vi "myRIO_BRig_RT_v0,76__PortC.vi"() -> ()   [LabVIEW 2014]
uses:
  <vilib>/Platform/TimedLoop/XDataNode/XDataNode.xnode
  <vilib>/Platform/TimedLoop/XDataNode/nitl_modes.ctl
  <vilib>/Platform/TimedLoop/XDataNode/XDNodeRunTimeDep.lvlib
  <vilib>/Platform/TimedLoop/XDataNode/wakeup.ctl
  <vilib>/Platform/TimedLoop/XDataNode/timing_clust.ctl
  <vilib>/rvi/interface/nirviReadWriteControl/nirviReadWriteControl.xnode
  <vilib>/rvi/interface/Simulation/niFpgaSimulationCallBeginRW.vi
  <vilib>/rvi/errors/niLvFpgaAdjustHostInterfaceError.vi
  <vilib>/rvi/interface/nirviCloseFPGA/nirviCloseFPGA.xnode
  <vilib>/myRIO/Instrument Drivers/Utilities/Utilities.lvlib
  <vilib>/rvi/interface/nirviOpenFPGA/nirviOpenFPGA.xnode
  myRIO_BRig_RT__Case_Exp_stateList.ctl
  <vilib>/WebDAVClient/Advanced/SessionHandle.ctl
  <vilib>/WebDAVClient/NI_WebDAV.lvlib
  myRIO_BRig_RT__Case_NonExp_stateList.ctl
  NiFpgaLv.dll
  <vilib>/Utility/error.llb/Error Cluster From Error Code.vi
  <vilib>/FPGAPlugInAG/Dynamic/niLvFpga_Close_Dynamic.vi
  myRIO_BRig_FPGA_v3,61__PortC__build.lvbitx
  myRIO_BRig_FPGA_v3,61__PortC.vi
  <vilib>/FPGAPlugInAG/myRIO-1900/niLvFpga_Open_myRIO-1900.vi
  <vilib>/rvi/interface/common/dynamic/niFpgaDynamicAddResources.vi
panel:
  in  "laser2_power_step":dbl
  in  "laser2_power_max":dbl
  in  "laser2_power_min":dbl
  in  "laser2_Tshutter":dbl=2.0
  in  "laser2_Freq":dbl=10.0
  in  "laser2_Tpeak":dbl=2.0
  in  "laser2_duration":u16
  in  "LC_l2_Sel_All_Count":u16
  in  "LC_l2_Sel_First_Count":u16
  in  "LC_l2_Sel_All_Probability":u16
  in  "LC_l2_Sel_All_Block":u16(slide) max=2 step=1 scale=0.0..2.0
  in  "LC_l2_Sel_All_OnOff":bool
  in  "LC_l2_Sel_First_Probability":u16
  in  "LC_l2_Sel_First_Block":u16(slide) max=2 step=1 scale=0.0..2.0
  in  "LC_l2_Sel_First_OnOff":bool
  in  "LC_l2_Sel_All_Tdelay":u16
  in  "LC_l2_Sel_First_Tdelay":u16
  in  "LC_l2_Cue1_All_Count":u16
  in  "LC_l2_Cue1_First_Count":u16
  in  "LC_l2_Cue1_All_delayOpt":bool
  in  "LC_l2_ENL1_All_delayOpt":bool
  in  "LC_l2_ENL1_All_Count":u16
  in  "LC_l2_ENL1_First_Count":u16
  in  "LC_l2_Cue1_First_delayOpt":bool
  in  "LC_l2_ENL1_First_delayOpt":bool
  in  "LC_l2_Cue1_All_Probability":u16
  in  "LC_l2_Cue1_All_Block":u16(slide) max=2 step=1 scale=0.0..2.0
  in  "LC_l2_Cue1_All_OnOff":bool
  in  "LC_l2_Cue1_First_Probability":u16
  in  "LC_l2_Cue1_First_Block":u16(slide) max=2 step=1 scale=0.0..2.0
  in  "LC_l2_Cue1_First_OnOff":bool
  in  "LC_l2_ENL1_All_Probability":u16 max=100 step=1
  in  "LC_l2_ENL1_All_Block":u16(slide) max=2 step=1 scale=0.0..2.0
  in  "LC_l2_ENL1_All_OnOff":bool
  in  "LC_l2_ENL1_First_Probability":u16 max=100 step=1
  in  "LC_l2_ENL1_First_Block":u16(slide) max=2 step=1 scale=0.0..2.0
  in  "LC_l2_Cue1_All_Tdelay":u16
  in  "LC_l2_ENL1_All_Tdelay":u16
  in  "LC_l2_Cue1_First_Tdelay":u16
  in  "LC_l2_ENL1_First_Tdelay":u16
  in  "LC_l2_ENL1_First_OnOff":bool
  in  "LC_l2_Wrong_Probability":u16
  in  "LC_l2_Wrong_Trial":u16(slide) max=2 step=1 scale=0.0..2.0
  in  "LC_l2_Wrong_Block":u16(slide) max=2 step=1 scale=0.0..2.0
  in  "LC_l2_Wrong_OnOff":bool
  in  "LC_l2_Reward_Probability":u16
  in  "LC_l2_Reward_Trial":u16(slide) max=2 step=1 scale=0.0..2.0
  in  "LC_l2_Reward_Block":u16(slide) max=2 step=1 scale=0.0..2.0
  in  "LC_l2_Reward_OnOff":bool
  in  "LC_l2_Wrong_Tdelay":u16
  in  "LC_l2_Reward_Tdelay":u16
  in  "LC_l1_Sel_All_Count":u16
  in  "LC_l1_Sel_First_Count":u16
  in  "LC_l1_Sel_All_Probability":u16
  in  "LC_l1_Sel_All_Block":u16(slide) max=2 step=1 scale=0.0..2.0
  in  "LC_l1_Sel_All_OnOff":bool
  in  "LC_l1_Sel_First_Probability":u16
  in  "LC_l1_Sel_First_Block":u16(slide) max=2 step=1 scale=0.0..2.0
  in  "LC_l1_Sel_First_OnOff":bool
  in  "LC_l1_Sel_All_Tdelay":u16
  in  "LC_l1_Sel_First_Tdelay":u16
  out "I_connect_TCP":bool
  out "error out 5":errorcluster
  in  "get_countPerMS":bool
  in  "count_warmup_R_reset":bool
  in  "count_warmup_L_reset":bool
  out "count_warmup_R":u16
  out "count_warmup_L":u16
  out "SolenoidReward":bool
  in  "SolenoidProbability_L":u16=50 caption="Reward Time [ms]" min=1 max=1000 step=1
  in  "SolenoidProbability_R":u16=50 caption="Reward Time [ms]" min=1 max=1000 step=1
  out "output_PortA":dbl caption="LaserPower"
  out "error out 4":errorcluster
  in  "laser1_power_step":dbl
  in  "laser1_power_max":dbl
  in  "Recording":bool
  out "error out 3":errorcluster
  out "error out 2":errorcluster
  in  "laser1_power_min":dbl
  in  "FPGA_count2ms":dbl=159.0
  in  "laser1_Tshutter":dbl=2.0
  in  "laser1_Freq":dbl=10.0
  in  "laser1_Tpeak":dbl=2.0
  in  "laser1_duration":u16
  out "error out":errorcluster
  in  "LC_l1_Cue1_All_Count":u16
  in  "LC_l1_Cue1_First_Count":u16
  in  "LC_l1_Cue1_All_delayOpt":bool
  in  "LC_l1_ENL1_All_delayOpt":bool
  in  "LC_l1_ENL1_All_Count":u16
  in  "LC_l1_ENL1_First_Count":u16
  in  "LC_l1_Cue1_First_delayOpt":bool
  in  "LC_l1_ENL1_First_delayOpt":bool
  in  "Tcycle_Cue_max":u16=1000 caption="Max" min=5 max=5000 step=5
  in  "Tcycle_Cue_min":u16=1000 caption="Min" min=5 max=5000 step=5
  in  "SendData":bool
  out "cSpout":enum16{"Left", "Right"}(ring) caption="Left or Right Spout"
  out "A4":u32 caption="LickCounter_Right"
  out "A2":u32 caption="LickCounter_Left"
  in  "laserResponse_wrong_LED":bool
  out "error_initTrial":errorcluster
  out "error_Selection_pre":errorcluster
  out "error_Selection":errorcluster
  out "SelectWrong":bool
  out "SelectReward":bool
  in  "Left(F)_or_Right(T)":bool
  in  "ignoreWrong":bool
  in  "SelectionState":bool
  in  "laserResponse_wrong":bool
  in  "laserResponse_reward":bool
  in  "laserResponse_reward_LED":bool
  out "nRewards_Right":u16 caption="# Rewards Total (Right)"
  out "nRewards_Left":u16 caption="# Rewards Total (Left)"
  out "nRewards_cur":u16 caption="# Rewards in Current Block"
  out "TpB_target":u16 caption="Target Trials Per Block"
  out "cState_NonExp":T1 caption="WarmUp State"
  out "iBlock":u16 caption="Current Block"
  out "cState":T2 caption="Experimental State"
  out "iTrial":u16 caption="Current Trial"
  in  "warmupType":u8(slide) max=2 step=1 scale=0.0..2.0
  in  "TestConnection":bool
  in  "warmup":bool caption="WarmUp"
  in  "Data Set Prefix":string="Exp1_TM2"
  out "Connected To Host?":bool
  in  "Host Password":string="sabalab"
  in  "Host UserName":string="Test2"
  in  "sp_RightSpout":u16(slide)=2 max=2 step=1 scale=0.0..2.0
  in  "sp_LeftSpout":u16(slide)=2 max=2 step=1 scale=0.0..2.0
  in  "BUR_max":u16 caption="Count Reward Structure  (0 = off)"
  in  "LC_l1_Wrong_Probability":u16
  in  "LC_l1_Wrong_Trial":u16(slide) max=2 step=1 scale=0.0..2.0
  in  "LC_l1_Wrong_Block":u16(slide) max=2 step=1 scale=0.0..2.0
  in  "LC_l1_Wrong_OnOff":bool
  in  "LC_l1_Reward_Probability":u16
  in  "LC_l1_Reward_Trial":u16(slide) max=2 step=1 scale=0.0..2.0
  in  "LC_l1_Reward_Block":u16(slide) max=2 step=1 scale=0.0..2.0
  in  "LC_l1_Reward_OnOff":bool
  in  "LC_l1_Cue1_All_Probability":u16
  in  "LC_l1_Cue1_All_Block":u16(slide) max=2 step=1 scale=0.0..2.0
  in  "LC_l1_Cue1_All_OnOff":bool
  in  "LC_l1_Cue1_First_Probability":u16
  in  "LC_l1_Cue1_First_Block":u16(slide) max=2 step=1 scale=0.0..2.0
  in  "LC_l1_Cue1_First_OnOff":bool
  in  "LC_l1_ENL1_All_Probability":u16 max=100 step=1
  in  "LC_l1_ENL1_All_Block":u16(slide) max=2 step=1 scale=0.0..2.0
  in  "LC_l1_ENL1_All_OnOff":bool
  in  "LC_l1_ENL1_First_Probability":u16 max=100 step=1
  in  "LC_l1_ENL1_First_Block":u16(slide) max=2 step=1 scale=0.0..2.0
  in  "Tcycle_Timeout":u16=1000 caption="Timeout Time [ms]" min=10 max=10000 step=1
  in  "Tcycle_Wrong":u16=1000 caption="Wrong Time [ms]" min=10 max=10000 step=1
  in  "Tcycle_Selection":u16=1000 caption="Answer Time [ms]" min=1 max=10000 step=1
  in  "Tcycle_RewardPost":u16=1000 caption="Consumption Time [ms]" min=250 max=10000 step=250
  in  "Tcycle_Reward_L":u16=500 caption="Reward Time [ms]" min=1 max=1000 step=1
  in  "Tcycle_Reward_R":u16=500 caption="Reward Time [ms]" min=1 max=1000 step=1
  in  "TpB_Max_R":u16=4 caption="Max TrialsPerBlock" min=1 max=12 step=1
  in  "TpB_Min_R":u16=4 caption="Min TrialsPerBlock" min=1 max=12 step=1
  in  "TpB_Max_L":u16=4 caption="Max TrialsPerBlock" min=1 max=12 step=1
  in  "TpB_Min_L":u16=4 caption="Min TrialsPerBlock" min=1 max=12 step=1
  in  "BUR_min":u16 caption="Count Reward Structure\n(0 = off)"
  in  "TrialUntilReward":bool caption="Ignore Wrong Selection"
  in  "CueCycles":u16=1 caption="Cue Structure" min=1 max=1 step=1
  in  "MTrig_Laser_Tcycle":u16=10 caption="Time [ms]"
  in  "MTrig_Laser_trig":bool
  in  "MTrig_Audio_trig__R":bool caption="Trigger Audio"
  in  "MTrig_Audio_trig__L":bool caption="Trigger Audio"
  in  "RewCalib_Trig_R":bool caption="Calibrate_R"
  in  "RewCalib_Trig_L":bool caption="Calibrate_L"
  in  "MTrig_Solenoid_Tcycle__R":u16=300 caption="Time [ms]"
  in  "MTrig_Solenoid_Tcycle__L":u16=300 caption="Time [ms]"
  in  "MTrig_Solenoid_trig__R":bool caption="Solenoid"
  in  "MTrig_Solenoid_trig__L":bool caption="Solenoid"
  in  "STOP_abort":bool caption="Stop LabView\n(Stops myRio and FPGA)"
  in  "STOP_endBlock":bool caption="Stop Experiment\n@ End of Block"
  in  "STOP_endTrial":bool caption="Stop Experiment\n@ End of Trial"
  in  "START":bool caption="Start Experiment"
  in  "Tcycle_CuePenalty":u16=1000 caption="Penalty" min=1 max=10000 step=1
  in  "Audio_Amp__R":u16=100 caption="Amp"
  in  "Audio_Freq__R":u8=5 caption="Freq [kHz]" max=14 step=1
  in  "Audio_Amp__L":u16=100 caption="Amp"
  in  "Audio_Freq__L":u8=5 caption="Freq [kHz]" max=14 step=1
  in  "LC_l1_Wrong_Tdelay":u16
  in  "LC_l1_Cue1_All_Tdelay":u16
  in  "LC_l1_ENL1_All_Tdelay":u16
  in  "LC_l1_Reward_Tdelay":u16
  in  "LC_l1_Cue1_First_Tdelay":u16
  in  "LC_l1_ENL1_First_Tdelay":u16
  in  "LC_l1_ENL1_First_OnOff":bool
  in  "Tcycle_ENLPenalty":u16=100 caption="Penalty" min=10 max=10000 step=10
  in  "Tcycle_ENL_max":u16=1000 caption="Max" min=250 max=10000 step=250
  in  "Tcycle_ENL_min":u16=1000 caption="Min" min=250 max=10000 step=250
  # "Communication (Host PC)"
  # "Recording Rig"
  # "Experimental Run"
  # "Current State"
  # "STOP experiment at"
  # "Global Parameters                                                         Trial Parameters"
  # "Left/Right        Give Reward?        Laser Power [V]"
  # "FPGA Count per [ms]"
  # "Experiment Task Structure"
  # "Timing [ms]"
  # "Block                   Trial            Target Trials       # Rewards \n                                                            Per Block             Current"
  # "Min            Max            Penalty"
  # "(1) = Switching\n(2) = Two Choice"
  # "WarmUp State"
  # "Lick Counter"
  # "Enforced\nNonLick"
  # "WarmUp"
  # "Left           Right"
  # "Cue then reward (no lick)\n \nLeft                    Right"
  # "# Rewards Total\n                                                                  Left                    Right"
  # "Cue"
  # "Experimental State"
  # "Selection\n \n\n \nReward\n    Dispense\n    Time\n \n    Dispense\n    Probability\n \n\n    Consumption\n    Time\n\nWrong Choice\n \n \nTimeout Penalty"
  # "Laser1 Control\n                               On/Off      Block        Probability [%]   Delay [ms]                              Count"
  # "Left                  Right"
  # "Manual Control"
  # "Enforced\nNonLick\n      1"
  # "Min"
  # "Max"
  # "from end"
  # "Solenoid\n \nLeft              Right"
  # "Switch\nTrial"
  # "Speaker\n \nLeft                    Right"
  # "Laser"
  # "from start"
  # "Trial Per Block Structure \n               Left                        Right"
  # "from end"
  # "NonSwitch\nTrials"
  # "from start"
  # "Time\n[ms]"
  # "Time\n[ms]"
  # "Time = Cue Min"
  # "Min"
  # "Cue 1"
  # "Power = Min"
  # "from end"
  # "Switch\nTrial"
  # "Max"
  # "from start"
  # "Speaker Parameters"
  # "Laser1 Parameters"
  # "Left                  Right"
  # "from end"
  # "Laser1 Response\n                               On/Off      Block       Trial       Probability [%]   Delay [ms]"
  # "Frequency\n[Hz]"
  # "NonSwitch\nTrials"
  # "Frequency\n[kHz]"
  # "from start"
  # "Timing [ms]\n Duration     Peak Width   Shutter"
  # "Selection Reward"
  # "Selection"
  # "Amp\n(0 - 32,000)"
  # "from start"
  # "Switch\nTrial"
  # "Laser Power [V]\nMin          Max              Step"
  # "Speaker\nPattern\nDuring Cue"
  # "Selection Wrong"
  # "from start"
  # "NonSwitch\nTrials"
  # "Laser2 Parameters"
  # "Laser2 Response\n                               On/Off      Block       Trial       Probability [%]   Delay [ms]"
  # "Laser2 Control\n                               On/Off      Block        Probability [%]   Delay [ms]                              Count"
  # "Frequency\n[Hz]"
  # "Selection Reward"
  # "Enforced\nNonLick\n      1"
  # "from end"
  # "Timing [ms]\n Duration     Peak Width   Shutter"
  # "Switch\nTrial"
  # "from start"
  # "Selection Wrong"
  # "from end"
  # "Laser Power [V]\nMin          Max              Step"
  # "NonSwitch\nTrials"
  # "from start"
  # "Cue 1"
  # "from end"
  # "Switch\nTrial"
  # "from start"
  # "from end"
  # "NonSwitch\nTrials"
  # "from start"
  # "Selection"
  # "from start"
  # "Switch\nTrial"
  # "from start"
  # "NonSwitch\nTrials"
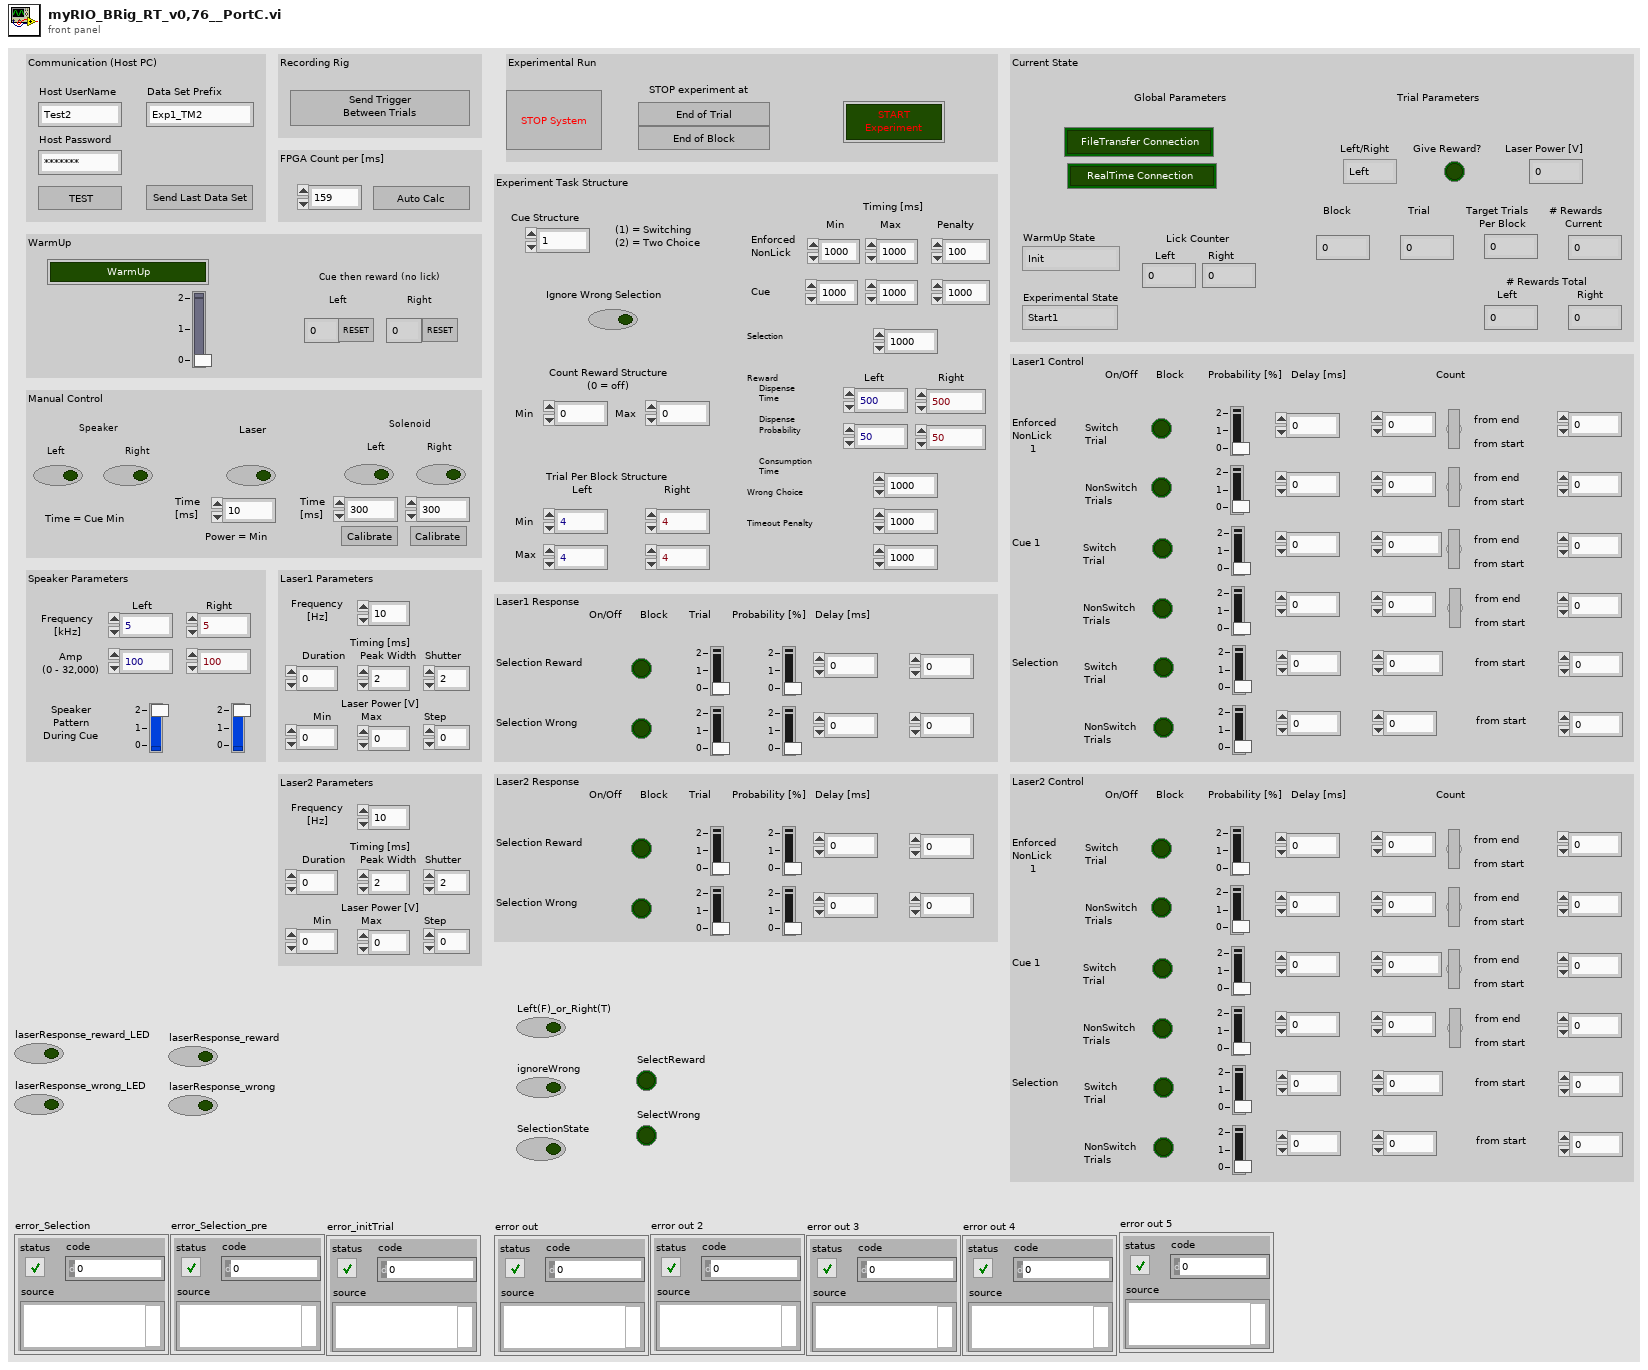
[diagram p1: front panel]
types:
  T1 = typedef "myRIO_BRig_RT__Case_NonExp_stateList.ctl" = enum16{"Init", "UploadSettings_pre", "UploadSettings_Read_dataExp", "UploadSettings_dataExp_1", "UploadSettings_dataExp_2", "UploadSettings_Read_dataLC", "UploadSettings_dataLC_1", "UploadSettings_dataLC_2", "UploadSettings_dataLC_3", "UploadSettings_dataLC_4", "UploadSettings_Read_dataMTrig", "UploadSettings_dataMTrig_1", "UploadSettings_post", "Idle_pre", "IdleEmpty", "IdleEmpty2", "IdleEmpty3", "IdleEmpty4", "Idle", "Idle_2", "Idle_3", "Idle_4", "Idle_5", "Idle_6", "Idle_post", "Cue_pre__pre", "Cue_pre", "Cue", "Cue_LED", "Cue_post", "RewardCalibration_pre", "DispenseWater_pre__pre", "DispenseWater_pre", "DispenseWater", "DispenseWater_post", "TestConnection", "SendData", "Get_FPGA_count_per_ms", "End"}
  T2 = typedef "myRIO_BRig_RT__Case_Exp_stateList.ctl" = enum16{"Start1", "Start2", "Start3", "saveSettings1", "saveSettings2", "saveSettings3", "saveSettings4", "saveSettings_LC_ENL_l1", "saveSettings_LC_ENL_l2", "saveSettings_LC_Cue_l1", "saveSettings_LC_Cue_l2", "saveSettings6_LC_l1_Other", "SaveSettings6_LC_l2_Other", "setSettings_Audio", "setSettings_Laser", "initBlock_pre", "initBlock", "initBlock2", "initBlock_post", "initTrial_pre", "initTrial", "initTrial2", "initTrial3", "initTrial4", "initTrial_LC_ENL1", "initTrial_LC_Cue1", "initTrial_LC_Cue1_2", "initTrial_LC_Sel", "initTrial_post", "ENL1_pre", "ENL1", "ENL1_post", "ENL1Penalty_pre", "ENL1Penalty", "ENL2_pre", "ENL2", "ENL2Penalty_pre", "ENL2Penalty", "Cue1_pre", "Cue1", "Cue1_post", "Cue1Penalty_pre", "Cue1Penalty", "Cue2_pre", "Cue2", "Cue2Penalty_pre", "Cue2Penalty", "Selection_pre", "Selection", "Select_post", "SelectReward_pre", "SelectReward", "SelectRewardPost_pre", "SelectRewardPost", "SelectWrong_pre", "SelectWrong", "SelectWrong_post", "SelectTimeout_pre", "SelectTimeout", "SelectTimeout_post", "endTrial_pre", "endTrial1", "endTrial2", "endTrial3", "endTrial_post", "endBlock_pre", "endBlock", "endBlock_post", "endExp", "commConnect", "commUpload_pre", "commUpload_dataBlock", "commUpload_dataCurrent", "commUpload_dataExp", "commUpload_dataLC", "commUpload_dataTrial", "commUpload_post", "saveData_pre", "saveData_dataBlock", "saveData_dataCurrent", "saveData_dataExp", "saveData_dataLC", "saveData_dataTrial", "saveData_post", "empty_endBlock1", "empty_endBlock2", "empty_endTrial1", "empty_endTrial2", "empty_endTrial3", "empty_endTrial4", "empty_endTrial5", "dummyState", "dummyState_endBlock"}
  T3 = typedef "XDNodeRunTimeDep.lvlib/timing_clust.ctl" = cluster{"Expected End [f-1]":u64, "Actual End [f-1]":u64, "Finished Late? [f-1]":bool, "Expected End [i-1]":u64, "Actual End [i-1]":u64, "Finished Late? [i-1]":bool, "Expected Start [i]":u64, "Actual Start [i]":u64, "Expected Start [f]":u64, "Actual Start [f]":u64, "Source Name":string, "Structure Name":string, "Period":i64, "Deadline":i64, "Offset":i64, "Start":i64, "Priority":i32, "Timeout":i32, "Mode":T4, "Wakeup Reason":T5, "Error":errorcluster, "Source Type":string, "Secondary Source Type":string, "Global End Time":u64, "Global Start Time":u64, "Frame Duration":u64, "Iteration Duration":u64, "Assigned CPU":i32, "I/O Scan Engine Mode":u32}
  T4 = typedef "XDNodeRunTimeDep.lvlib/nitl_modes.ctl" = enum32{"No Change", "Process missed periods, maintain original phase", "Discard missed periods, maintain original phase", "Process missed periods, ignore original phase", "Discard missed periods, ignore original phase"}
  T5 = typedef "XDNodeRunTimeDep.lvlib/wakeup.ctl" = enum32{"Normal", "Aborted", "Asynchronous wakeup", "Timing source error", "Timed loop error", "Timeout"}
  T6 = typedef "myRIO_BRig_RT__Case_Exp_stateList.ctl" = enum16{"Start1", "Start2", "Start3", "saveSettings1", "saveSettings2", "saveSettings3", "saveSettings4_LC_l1_ENL", "saveSettings4_LC_l2_ENL", "saveSettings5_LC_l1_Cue", "saveSettings5_LC_l2_Cue", "saveSettings6_LC_l1_Other", "SaveSettings6_LC_l2_Other", "setSettings_Audio", "setSettings_Laser", "initBlock_pre", "initBlock", "initBlock2", "initBlock_post", "initTrial_pre", "initTrial", "initTrial2", "initTrial3", "initTrial4", "initTrial_LC_ENL1", "initTrial_LC_Cue1", "initTrial_LC_Cue1_2", "initTrial_LC_Sel", "initTrial_post", "ENL1_pre", "ENL1", "ENL1_post", "ENL1Penalty_pre", "ENL1Penalty", "ENL2_pre", "ENL2", "ENL2Penalty_pre", "ENL2Penalty", "Cue1_pre", "Cue1", "Cue1_post", "Cue1Penalty_pre", "Cue1Penalty", "Cue2_pre", "Cue2", "Cue2Penalty_pre", "Cue2Penalty", "Selection_pre", "Selection", "Select_post", "SelectReward_pre", "SelectReward", "SelectRewardPost_pre", "SelectRewardPost", "SelectWrong_pre", "SelectWrong", "SelectWrong_post", "SelectTimeout_pre", "SelectTimeout", "SelectTimeout_post", "endTrial_pre", "endTrial1", "endTrial2", "endTrial3", "endTrial_post", "endBlock_pre", "endBlock", "endBlock_post", "endExp", "commConnect", "commUpload_pre", "commUpload_dataBlock", "commUpload_dataCurrent", "commUpload_dataExp", "commUpload_dataLC", "commUpload_dataTrial", "commUpload_post", "saveData_pre", "saveData_dataBlock", "saveData_dataCurrent", "saveData_dataExp", "saveData_dataLC", "saveData_dataTrial", "saveData_post", "empty_endBlock1", "empty_endBlock2", "empty_endTrial1", "empty_endTrial2", "empty_endTrial3", "empty_endTrial4", "empty_endTrial5", "dummyState", "dummyState_endBlock"}
  T7 = typedef "NI_WebDAV.lvlib/SessionHandle.ctl" = refnum<k1>
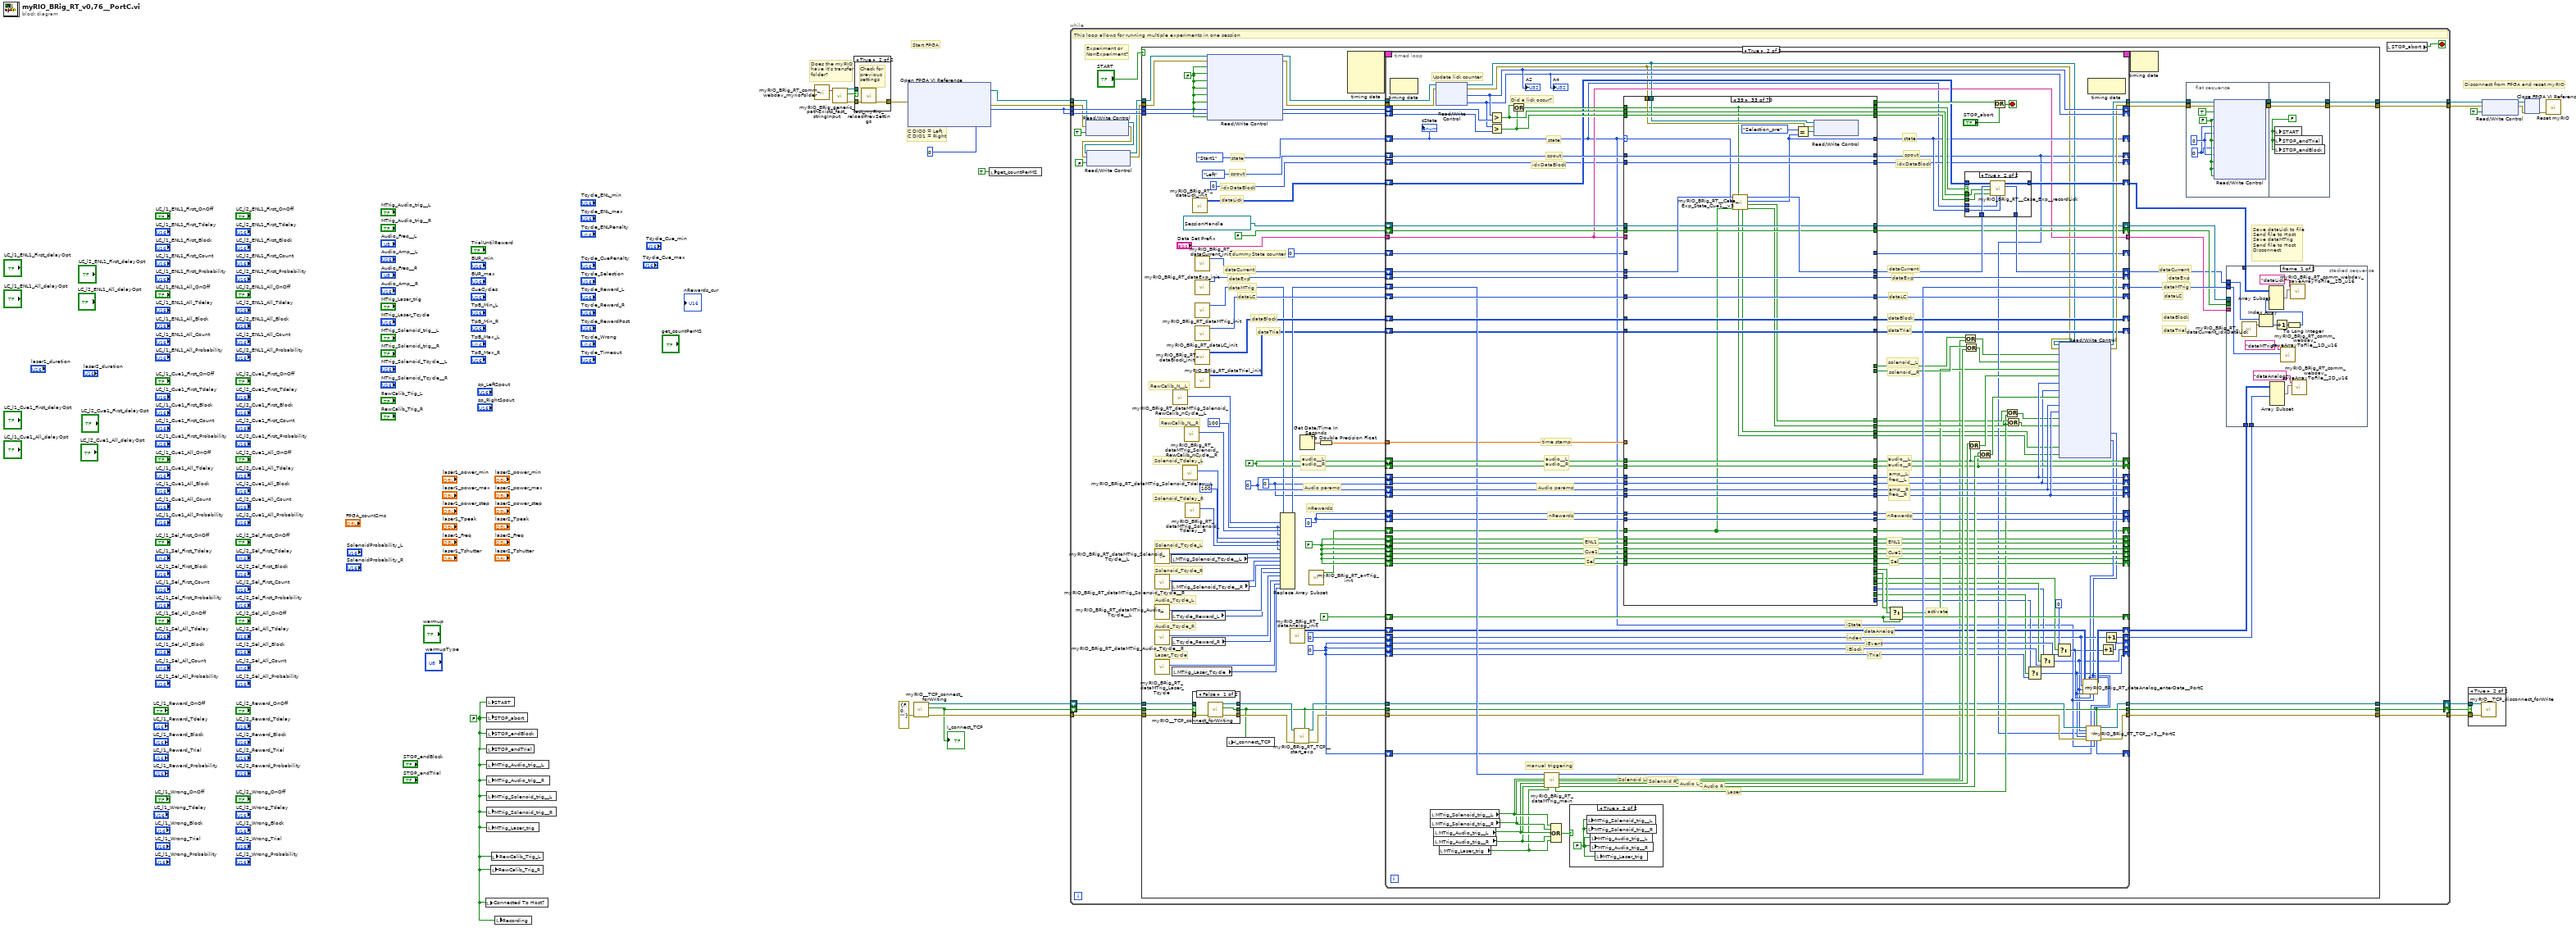
[diagram p0: block diagram]
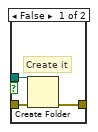
[diagram p3: hidden frame]
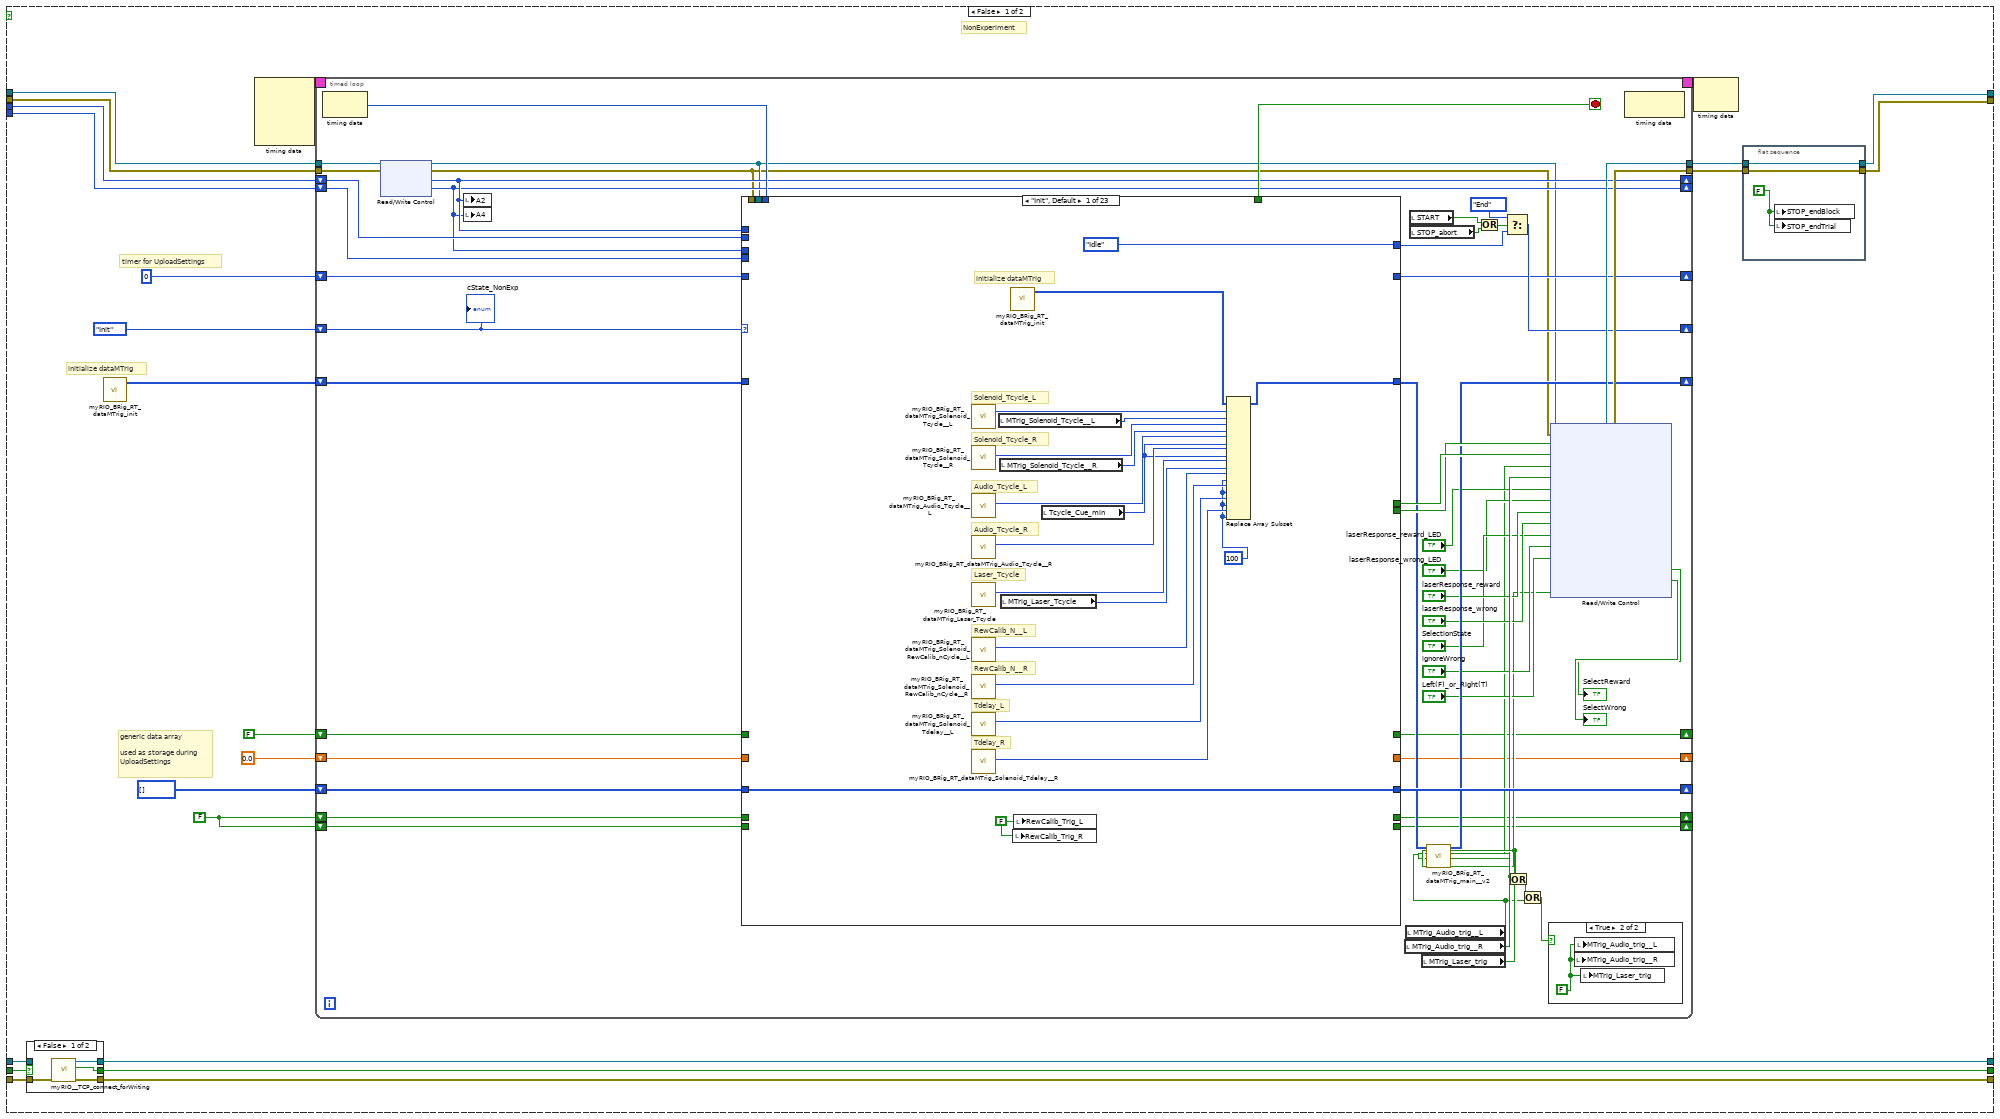
[diagram p4: hidden frame]
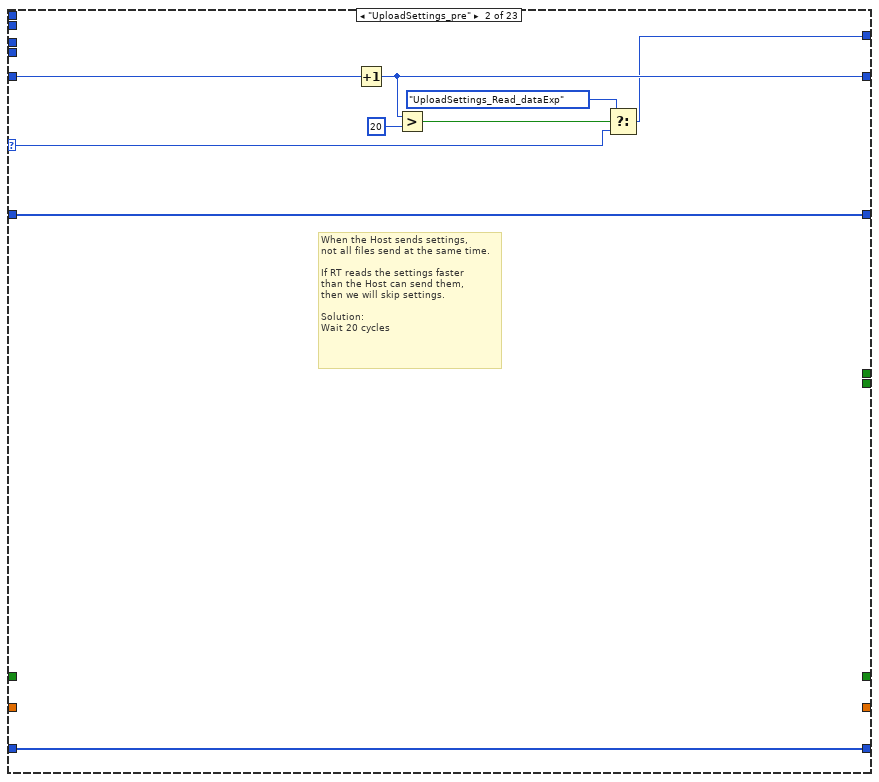
[diagram p7: hidden frame]
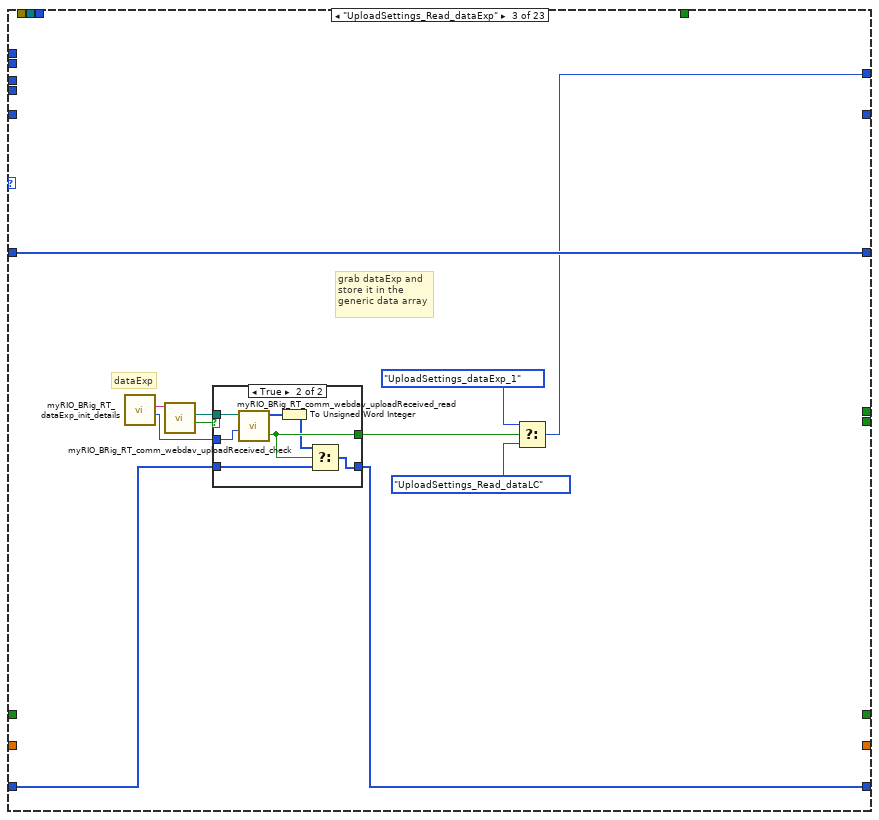
[diagram p8: hidden frame]
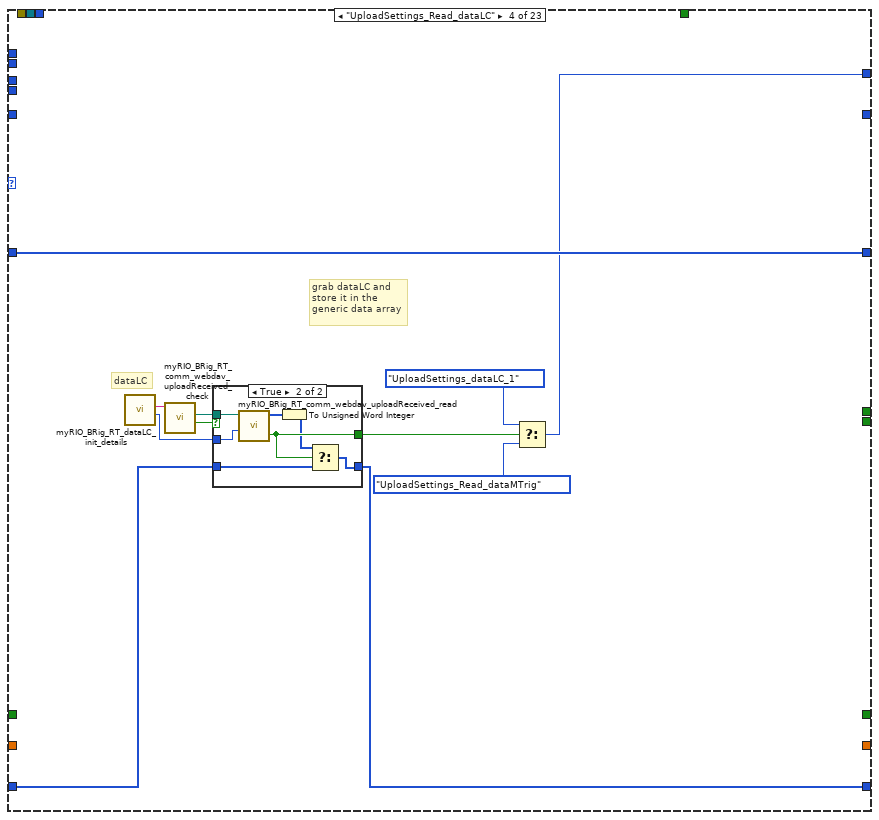
[diagram p10: hidden frame]
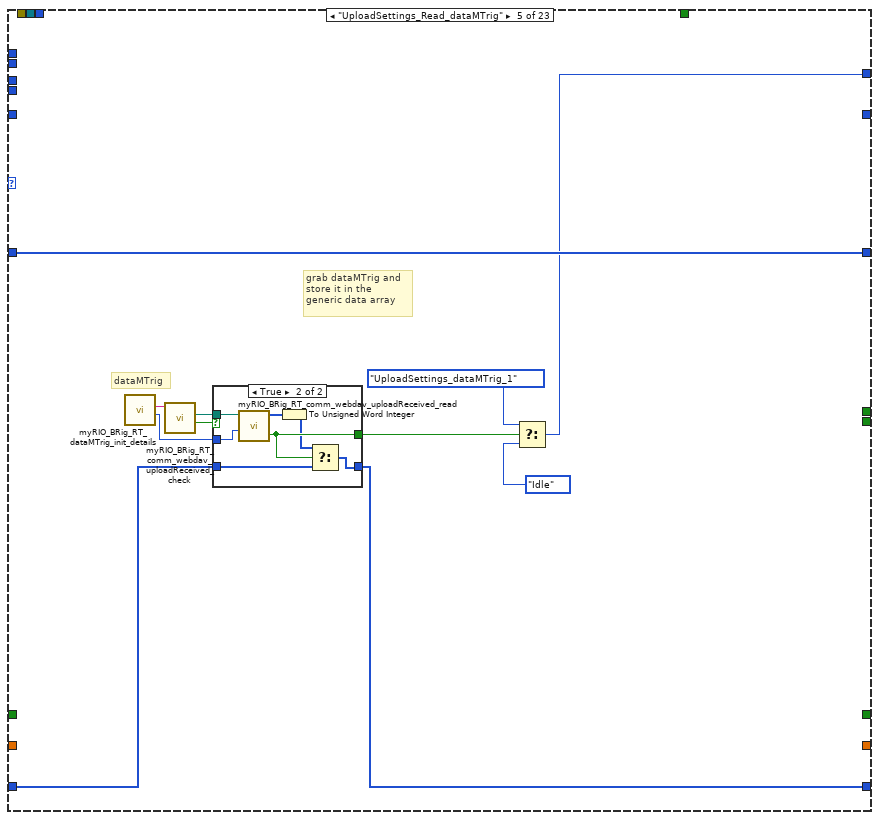
[diagram p12: hidden frame]
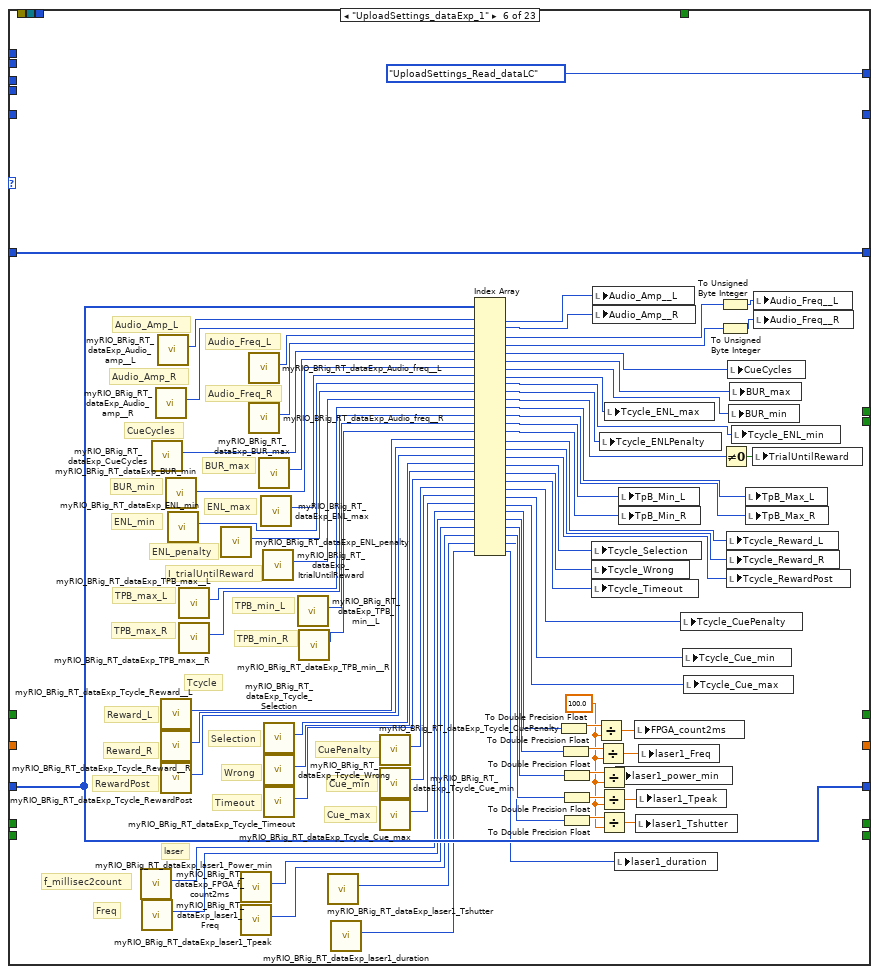
[diagram p14: hidden frame]
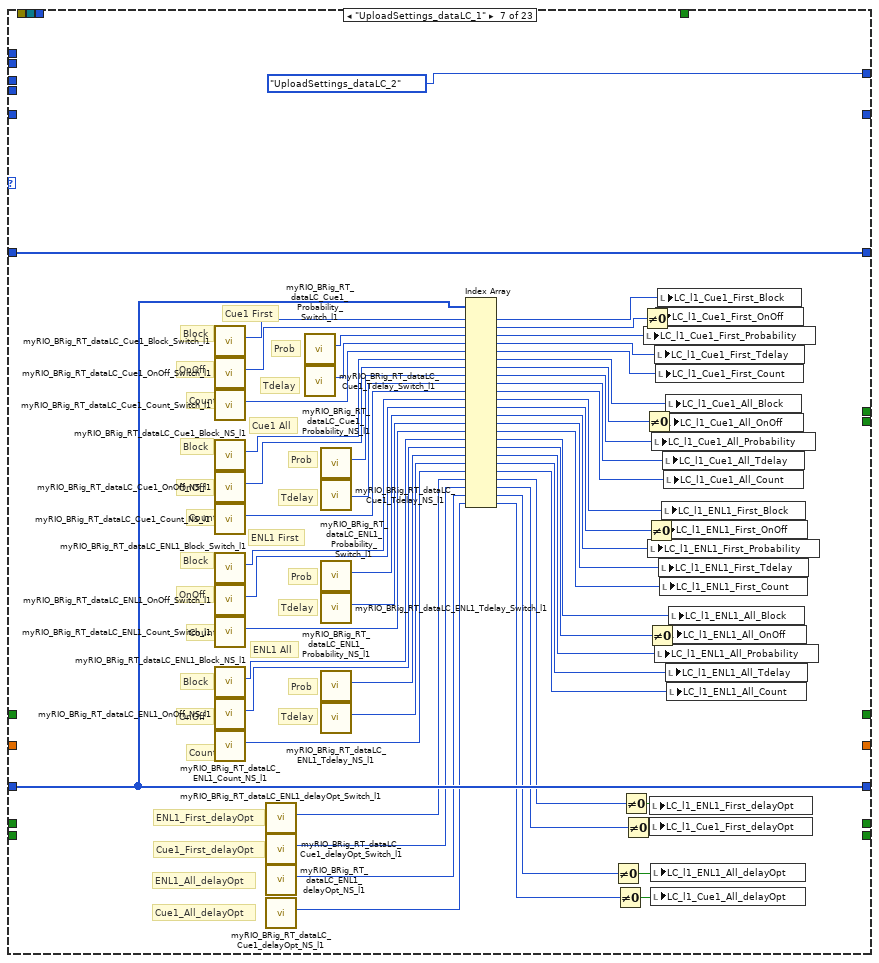
[diagram p15: hidden frame]
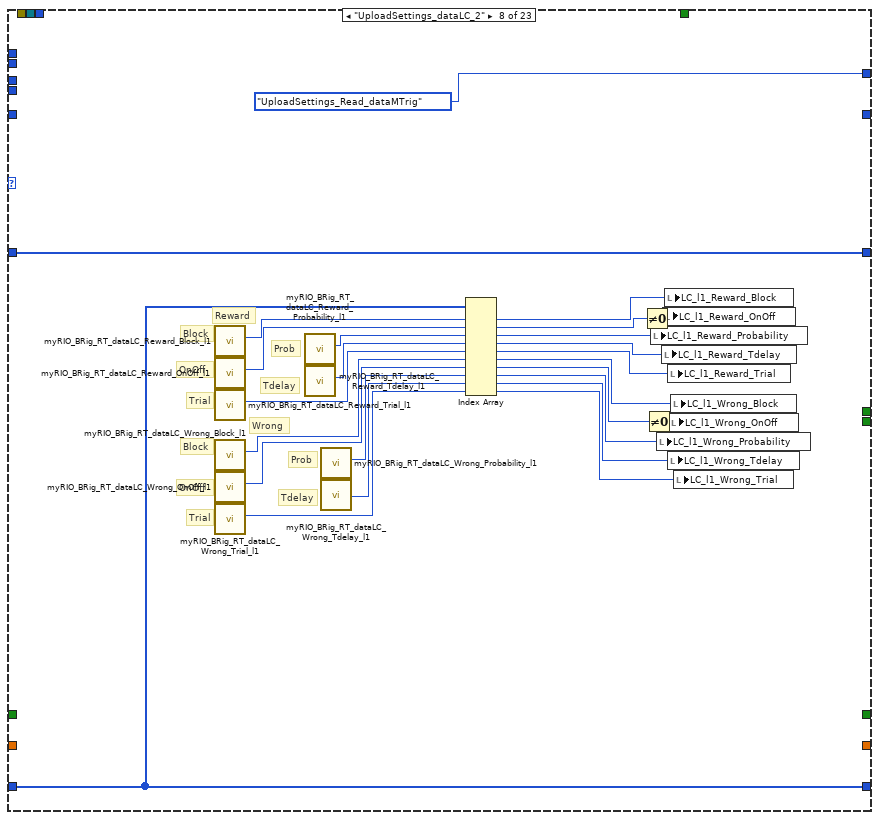
[diagram p16: hidden frame]
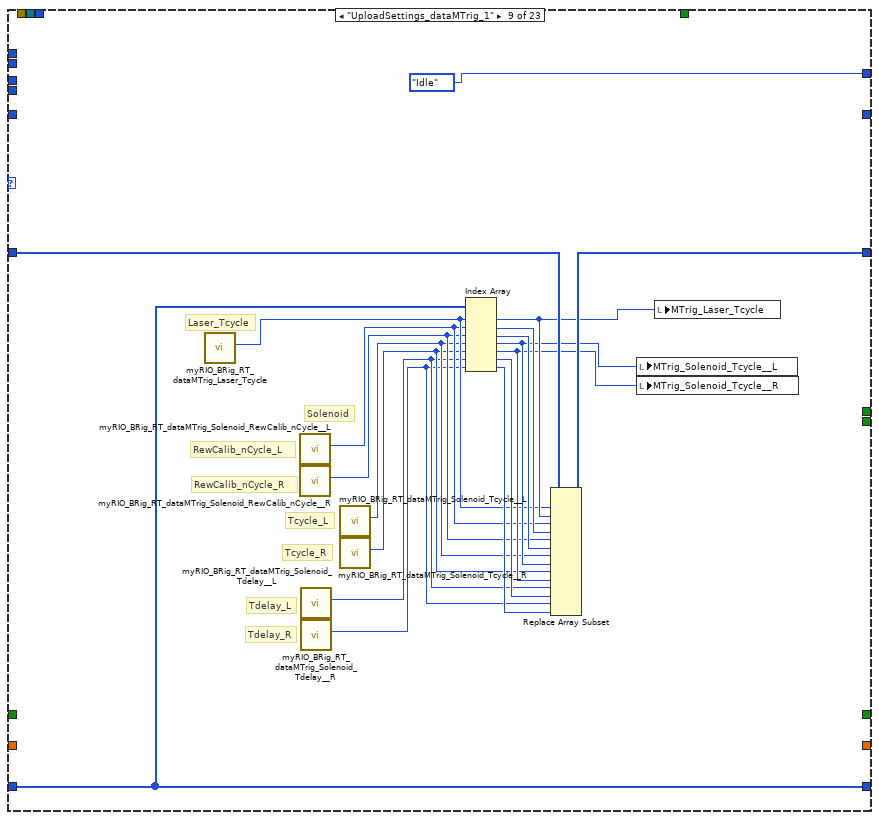
[diagram p17: hidden frame]
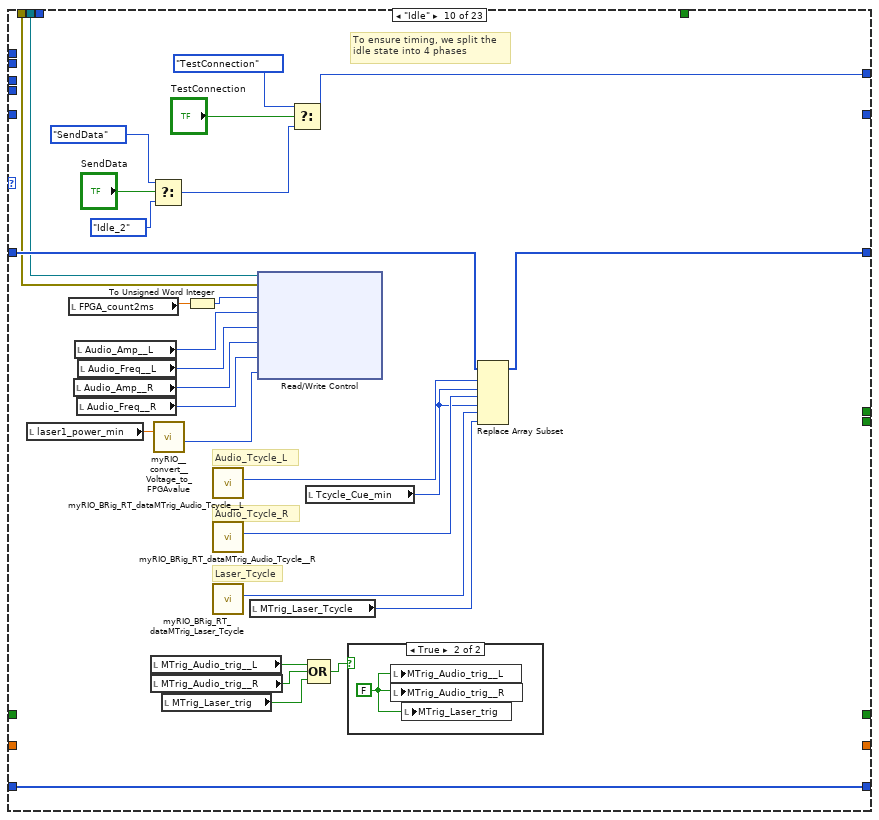
[diagram p18: hidden frame]
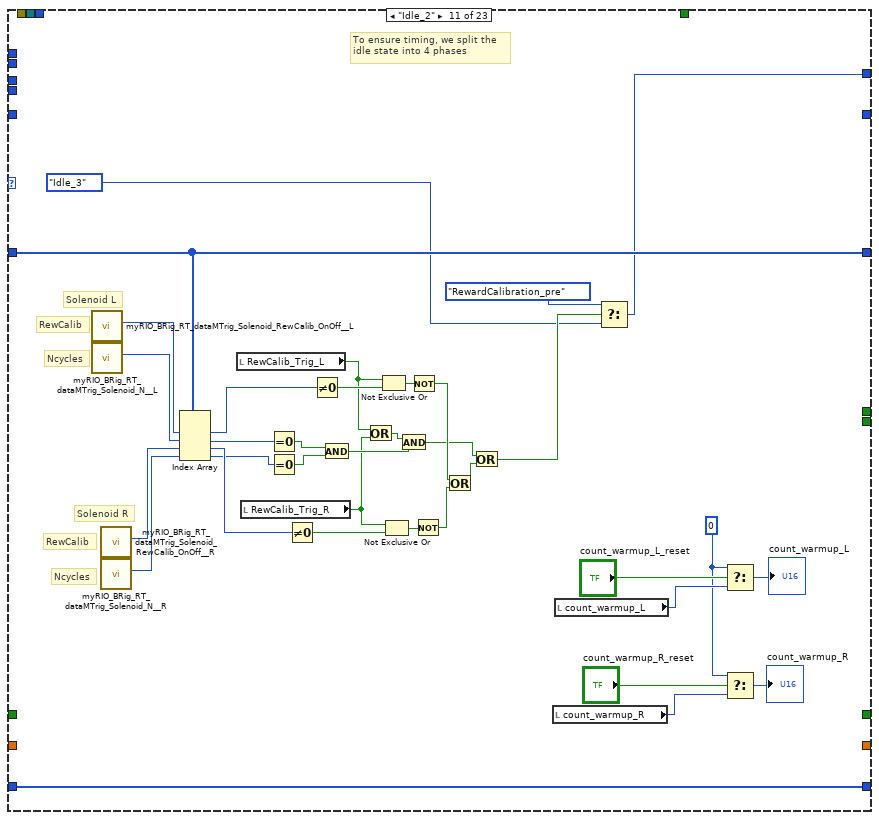
[diagram p20: hidden frame]
diagram:
  w17 = u32 0
  w1 = FALSE
  # "Does the myRIO\nhave it's transfer\nfolder?"
  # "C DIO0 = Left\nC DIO1 = Right"
  # "Start FPGA"
  # "Disconnect from FPGA and reset myRIO"
  n1 = local write "Connected To Host?"(w1) -> ()
  n2 = local write "START"(w1) -> ()
  n3 = local write "STOP_abort"(w1) -> ()
  n4 = local write "STOP_endBlock"(w1) -> ()
  n5 = local write "STOP_endTrial"(w1) -> ()
  n6 = local write "MTrig_Audio_trig__L"(w1) -> ()
  n7 = local write "MTrig_Audio_trig__R"(w1) -> ()
  n8 = local write "MTrig_Solenoid_trig__L"(w1) -> ()
  n9 = local write "MTrig_Solenoid_trig__R"(w1) -> ()
  n10 = local write "MTrig_Laser_trig"(w1) -> ()
  n11 = local write "RewCalib_Trig_R"(w1) -> ()
  n12 = local write "RewCalib_Trig_L"(w1) -> ()
  n13 = local write "Recording"(w1) -> ()
  n14 = call "myRIO_BRig_RT_comm_webdav_myrioFolder.vi"() -> ("output_myrioFolder"=w14:string)  [unwired: 11 in]
  n15 = call "myRIO_BRig_generic_pathExists_fast_stringInput.vi"("input_filePath"=w14) -> ("output_error"=w13:errorcluster, "output_Iexist"=w12:bool, "output_filePath"=w11:path)  [unwired: 8 in]
  n16 = case shown="True" w12 {
    tunnel: w11 -> [w26 _]
    tunnel: w13 -> [w25 w28]
    tunnel: [w24 w27] -> w9
    frame False {
      # "Create it"
      n17 = Create Folder(path (use dialog)=w26, error in=w25) -> (error out=w24:errorcluster)  [unwired: 1 in, 2 out]
    }
    frame True {
      # "Check for\nprevious\nsettings"
      n18 = call "test_myRio_reloadPrevSettings.vi"("input_error"=w28) -> ("output_error"=w27:errorcluster)  [unwired: 10 in]
    }
  }
  n19 = xnode "Open FPGA VI Reference"("error in"=w9) -> ("FPGA VI Reference Out"=w19:refnum<k20>, "error out"=w18:errorcluster)  [unwired: 1 in]
  n20 = call "myRIO__TCP_connect_forWriting.vi"("input_error"=errorcluster {"status"=FALSE, "code"=0, "source"=""}) -> ("output_error"=w7:errorcluster, "output_connected"=w6:bool, "output_hTCP"=w10:refnum<k5>)  [unwired: 8 in]
  "I_connect_TCP" <- w6
  n21 = local write "get_countPerMS"(TRUE ("get_countPerMS")) -> ()
  n22 = while {
    tunnel: w19 -> [w38]
    tunnel: w18 -> [w43]
    tunnel: w17 -> [w46]
    tunnel: w17 -> [w45]
    tunnel: [w36] -> w16
    tunnel: [w35] -> w15
    shift-right: [w32] -> w5
    shift-left: w6 -> [w33]
    tunnel: w7 -> [w31]
    shift-right: [w30] -> w4
    shift-left: w10 -> [w34]
    tunnel: [w29] -> w3
    stop <- w44 stop-if-true
    # "Experiment or\nNonExperiment?"
    # "This loop allows for running multiple experiments in one session"
    n23 = xnode "Read/Write Control"("FPGA VI Reference In"=w38, "error in"=w43, "Counts_Reset"=TRUE) -> ("FPGA VI Reference Out"=w40:refnum<k20>, "error out"=w41:errorcluster)
    n24 = xnode "Read/Write Control"("FPGA VI Reference In"=w40, "error in"=w41, "Counts_Reset"=FALSE) -> ("FPGA VI Reference Out"=w37:refnum<k20>, "error out"=w39:errorcluster)
    n25 = case shown="True" "START" {
      tunnel: w46 -> [w67 w996]
      tunnel: w45 -> [w66 w995]
      tunnel: w39 -> [w64 w946]
      tunnel: w37 -> [w65 w945]
      tunnel: [w62 w992] -> w36
      tunnel: [w60 w987] -> w35
      tunnel: w34 -> [w53 w933]
      tunnel: [w51 w937] -> w30
      tunnel: w33 -> [w52 w935]
      tunnel: [w50 w936] -> w32
      tunnel: w31 -> [w54 w934]
      tunnel: [w49 w932] -> w29
      frame False {
        w57 = FALSE
        # "generic data array\n\nused as storage during\nUploadSettings"
        # "timer for UploadSettings"
        # "initialize dataMTrig"
        # "NonExperiment"
        n26 = case shown="False" w52 {
          selector: w52 -> [_ w76]
          tunnel: w54 -> [w73 w78]
          tunnel: [w74 w78] -> w49
          tunnel: w53 -> [_ w77]
          tunnel: [w75 w77] -> w51
          tunnel: [w72 w76] -> w50
          frame False {
            n27 = call "myRIO__TCP_connect_forWriting.vi"("input_error"=w73) -> ("output_error"=w74:errorcluster, "output_connected"=w72:bool, "output_hTCP"=w75:refnum<k5>)  [unwired: 8 in]
          }
          frame True {
          }
        }
        n28 = call "myRIO_BRig_RT_dataMTrig_init.vi"() -> ("output_dataMTrig"=w68:u16[])  [unwired: 5 in]
        n29 = node-c288() -> (w71:T3)  [unwired: 4 in]
        n30 = timed-loop {
          timing: w71 -> [_]
          timing-out: [_] -> w70
          shift-right: [w121] -> _
          shift-left: w68 -> [w133]
          shift-right: [w110] -> _
          shift-left: myRIO_BRig_RT__Case_NonExp_stateList."Init" ("Enum") -> [w127]
          shift-right: [w94] -> _
          shift-left: w67 -> [w95]
          shift-right: [w92] -> _
          shift-left: w66 -> [w93]
          tunnel: [w129] -> w63
          tunnel: [w128] -> w61
          tunnel: w64 -> [w131]
          tunnel: w65 -> [w130]
          shift-right: [w126] -> _
          shift-left: u16[] [] ("output_data") -> [w125]
          shift-right: [w96] -> _
          shift-left: u16 0 ("Audio_Amp__L") -> [w97]
          shift-right: [w89] -> _
          shift-left: w57 -> [w91]
          shift-right: [w88] -> _
          shift-left: w57 -> [w90]
          shift-right: [w84] -> _
          shift-left: FALSE -> [w85]
          shift-right: [w82] -> _
          shift-left: 0.0 -> [w83]
          stop <- w134 stop-if-true
          n31 = node-c288() -> (w132:i64)  [unwired: 1 in]
          n32 = xnode "Read/Write Control"("FPGA VI Reference In"=w130, "error in"=w131) -> ("FPGA VI Reference Out"=w87:refnum<k20>, "error out"=w86:errorcluster, "A2_LickL"=w94:u32, "A4_LickR"=w92:u32)
          n33 = local write "A2"(w94) -> ()
          n34 = local write "A4"(w92) -> ()
          n35 = case shown="\"Init\", Default" w127 {
            selector: w127 -> [_ w159 _ _ _ _ _ _ _ _ _ _ _ _ w590 _ _ w798 _ _ _ w873 w917]
            tunnel: [myRIO_BRig_RT__Case_NonExp_stateList."Idle" ("Enum") w157 w164 w183 w202 myRIO_BRig_RT__Case_NonExp_stateList."UploadSettings_Read_dataLC" ("Enum") myRIO_BRig_RT__Case_NonExp_stateList."UploadSettings_dataLC_2" ("Enum") myRIO_BRig_RT__Case_NonExp_stateList."UploadSettings_Read_dataMTrig" ("f") myRIO_BRig_RT__Case_NonExp_stateList."Idle" ("Enum") w421 w438 w477 w558 myRIO_BRig_RT__Case_NonExp_stateList."Cue" ("t") w585 myRIO_BRig_RT__Case_NonExp_stateList."DispenseWater_pre" ("Enum") w743 w796 w819 myRIO_BRig_RT__Case_NonExp_stateList."Idle" ("Enum") myRIO_BRig_RT__Case_NonExp_stateList."Idle" ("Enum") w872 w917] -> w111
            tunnel: [w146 w156 w174 w193 w212 w297 w356 w381 w397 w425 w453 w482 w556 w574 w591 w653 w780 w803 w830 w865 w871 w884 w915] -> w122
            tunnel: [_ _ _ _ _ _ _ _ _ _ _ _ _ _ _ _ _ _ _ _ _ _ TRUE] -> w134
            tunnel: w133 -> [_ w156 w174 w193 w212 w297 w356 w381 w398 w424 w453 w483 w556 w575 w592 w639 w776 w804 w831 w865 w871 w884 w915]
            tunnel: w132 -> [_ _ _ _ _ _ _ _ _ _ _ _ _ _ _ _ _ w808 _ _ _ _ _]
            tunnel: [w139 w155 w165 w184 w203 w246 w312 w357 w382 w416 w437 w471 w555 w564 w599 w634 w728 w781 w812 w857 w869 w883 w914] -> w126
            tunnel: w125 -> [w139 w155 w166 w185 w204 w246 w312 w357 w382 w416 w437 w471 w555 w564 w599 w634 w728 w781 w812 w857 w869 w883 w914]
            tunnel: [_ _ _ _ _ _ _ _ _ _ _ _ _ _ _ _ _ w805 _ _ _ _ _] -> w124
            tunnel: [_ _ _ _ _ _ _ _ _ _ _ _ _ _ _ _ _ w787 _ _ _ _ _] -> w123
            tunnel: w97 -> [_ w163 _ _ _ _ _ _ _ _ _ _ _ _ _ _ _ _ _ _ _ _ _]
            tunnel: [_ w162 _ _ _ _ _ _ _ _ _ _ _ _ _ _ _ _ _ _ _ _ _] -> w96
            tunnel: w95 -> [_ _ _ _ _ _ _ _ _ _ _ _ _ _ w596 _ _ _ _ _ _ _ _]
            tunnel: w94 -> [_ _ _ _ _ _ _ _ _ _ _ _ _ _ w597 _ _ _ _ _ _ _ _]
            tunnel: w93 -> [_ _ _ _ _ _ _ _ _ _ _ _ _ _ w594 _ _ _ _ _ _ _ _]
            tunnel: w92 -> [_ _ _ _ _ _ _ _ _ _ _ _ _ _ w595 _ _ _ _ _ _ _ _]
            tunnel: w91 -> [_ _ _ _ _ _ _ _ _ _ _ _ _ _ w582 _ _ _ _ _ _ _ _]
            tunnel: w90 -> [_ _ _ _ _ _ _ _ _ _ _ _ _ _ w581 _ _ _ _ _ _ _ _]
            tunnel: [_ _ _ _ _ _ _ _ _ _ _ _ _ w563 w582 _ _ _ _ _ _ _ _] -> w89
            tunnel: [_ _ _ _ _ _ _ _ _ _ _ _ _ w562 w581 _ _ _ _ _ _ _ _] -> w88
            tunnel: w87 -> [_ _ _ _ _ _ _ _ _ w407 _ _ _ _ _ _ _ _ _ _ _ w878 _]
            tunnel: w86 -> [_ _ _ _ _ _ _ _ _ w406 _ _ _ _ _ _ _ _ _ _ _ w877 _]
            tunnel: w85 -> [_ _ _ _ _ _ _ _ _ _ _ _ _ _ _ _ _ _ _ _ _ w882 _]
            tunnel: [_ _ _ _ _ _ _ _ _ _ _ _ _ _ _ _ _ _ _ _ _ TRUE _] -> w84
            tunnel: w83 -> [_ _ _ _ _ _ _ _ _ _ _ _ _ _ _ _ _ _ _ _ _ w880 _]
            tunnel: [_ _ _ _ _ _ _ _ _ _ _ _ _ _ _ _ _ _ _ _ _ w879 _] -> w82
            frame "Init", Default {
              w140 = FALSE ("RewCalib_Trig_L")
              w136 = u16 100 ("new element/subarray")
              # "Tdelay_R"
              # "Tdelay_L"
              # "RewCalib_N__R"
              # "RewCalib_N__L"
              # "Solenoid_Tcycle_R"
              # "Solenoid_Tcycle_L"
              # "Laser_Tcycle"
              # "Audio_Tcycle_R"
              # "Audio_Tcycle_L"
              # "initialize dataMTrig"
              n36 = call "myRIO_BRig_RT_dataMTrig_Solenoid_Tcycle__L.vi"() -> ("output_Solenoid_Tcycle__L"=w148:i32)  [unwired: 11 in]
              n37 = call "myRIO_BRig_RT_dataMTrig_Solenoid_Tcycle__R.vi"() -> ("output_Solenoid_Tcycle__R"=w149:i32)  [unwired: 11 in]
              n38 = call "myRIO_BRig_RT_dataMTrig_Audio_Tcycle__L.vi"() -> ("output_Audio_Tcycle__L"=w150:i32)  [unwired: 11 in]
              n39 = call "myRIO_BRig_RT_dataMTrig_Audio_Tcycle__R.vi"() -> ("output_Audio_Tcycle__R"=w151:i32)  [unwired: 11 in]
              n40 = call "myRIO_BRig_RT_dataMTrig_Laser_Tcycle.vi"() -> ("output_Laser_Tcycle"=w152:i32)  [unwired: 11 in]
              n41 = call "myRIO_BRig_RT_dataMTrig_Solenoid_RewCalib_nCycle__L.vi"() -> ("output_Solenoid_RewCalib_nCycle__L"=w144:i32)  [unwired: 11 in]
              n42 = call "myRIO_BRig_RT_dataMTrig_Solenoid_RewCalib_nCycle__R.vi"() -> ("output_Solenoid_RewCalib_nCycle__R"=w143:i32)  [unwired: 11 in]
              n43 = call "myRIO_BRig_RT_dataMTrig_Solenoid_Tdelay__L.vi"() -> ("output_Solenoid_Tdelay__L"=w142:i32)  [unwired: 11 in]
              n44 = call "myRIO_BRig_RT_dataMTrig_Solenoid_Tdelay__R.vi"() -> ("output_Solenoid_Tdelay__R"=w141:i32)  [unwired: 11 in]
              n45 = local read "MTrig_Solenoid_Tcycle__L"() -> (w153:u16)
              n46 = local read "MTrig_Solenoid_Tcycle__R"() -> (w154:u16)
              n47 = local read "MTrig_Laser_Tcycle"() -> (w137:u16)
              n48 = call "myRIO_BRig_RT_dataMTrig_init.vi"() -> ("output_dataMTrig"=w147:u16[])  [unwired: 5 in]
              n49 = local write "RewCalib_Trig_R"(w140) -> ()
              n50 = local write "RewCalib_Trig_L"(w140) -> ()
              n51 = local read "Tcycle_Cue_min"() -> (w138:u16)
              n52 = Replace Array Subset(array=w147, new element #1=w153, index #1=w148, new element #2=w154, index #2=w149, new element #3=w138, index #3=w150, new element #4=w138, index #4=w151, new element #5=w137, index #5=w152, new element #6=w136, index #6=w144, new element #7=w136, index #7=w143, new element #8=w136, index #8=w142, new element #9=w136, index #9=w141) -> (w146:u16[])
            }
            frame "UploadSettings_pre" {
              # "When the Host sends settings,\nnot all files send at the same time.\n\nIf RT reads the settings faster\nthan the Host can send them,\nthen we will skip settings.\n\nSolution:\nWait 20 cycles"
              n53 = Increment(x=w163) -> (x+1=w162:u16)
              n54 = Greater?(x=w162, y=u16 20) -> (0:w160:bool)
              n55 = Select(t=myRIO_BRig_RT__Case_NonExp_stateList."UploadSettings_Read_dataExp", s=w160, f=w159) -> (s? t:f=w157:T1)
            }
            frame "UploadSettings_Read_dataExp" {
              # "grab dataExp and\nstore it in the\ngeneric data array"
              # "dataExp"
              n56 = call "myRIO_BRig_RT_dataExp_init_details.vi"() -> ("output_dataSize"=w170:i32, "output_dataName"=w173:string)  [unwired: 10 in]
              n57 = call "myRIO_BRig_RT_comm_webdav_uploadReceived_check.vi"("input_dataName"=w173) -> ("output_Iexist"=w172:bool, "output_dataPath"=w171:path)  [unwired: 9 in]
              n58 = case shown="True" w172 {
                tunnel: w171 -> [_ w182]
                tunnel: w170 -> [_ w181]
                tunnel: [_ w180] -> w169
                tunnel: w166 -> [w175 w179]
                tunnel: [w175 w176] -> w165
                frame False {
                }
                frame True {
                  n59 = call "myRIO_BRig_RT_comm_webdav_uploadReceived_read.vi"("input_dataSize"=w181, "input_filePath"=w182) -> ("output_Ivalid"=w180:bool, "output_data"=w178:i64[])  [unwired: 8 in]
                  n60 = To Unsigned Word Integer(number=w178) -> (unsigned 16bit integer=w177:u16[])
                  n61 = Select(t=w177, s=w180, f=w179) -> (s? t:f=w176:u16[])
                }
              }
              n62 = Select(t=myRIO_BRig_RT__Case_NonExp_stateList."UploadSettings_dataExp_1", s=w169, f=myRIO_BRig_RT__Case_NonExp_stateList."UploadSettings_Read_dataLC" ("t")) -> (s? t:f=w164:T1)
            }
            frame "UploadSettings_Read_dataLC" {
              # "grab dataLC and\nstore it in the\ngeneric data array"
              # "dataLC"
              n63 = call "myRIO_BRig_RT_dataLC_init_details.vi"() -> ("output_dataSize"=w189:i32, "output_dataName"=w192:string)  [unwired: 10 in]
              n64 = call "myRIO_BRig_RT_comm_webdav_uploadReceived_check.vi"("input_dataName"=w192) -> ("output_Iexist"=w191:bool, "output_dataPath"=w190:path)  [unwired: 9 in]
              n65 = case shown="True" w191 {
                tunnel: w190 -> [_ w201]
                tunnel: w189 -> [_ w200]
                tunnel: [_ w199] -> w188
                tunnel: w185 -> [w194 w198]
                tunnel: [w194 w195] -> w184
                frame False {
                }
                frame True {
                  n66 = call "myRIO_BRig_RT_comm_webdav_uploadReceived_read.vi"("input_dataSize"=w200, "input_filePath"=w201) -> ("output_Ivalid"=w199:bool, "output_data"=w197:i64[])  [unwired: 8 in]
                  n67 = To Unsigned Word Integer(number=w197) -> (unsigned 16bit integer=w196:u16[])
                  n68 = Select(t=w196, s=w199, f=w198) -> (s? t:f=w195:u16[])
                }
              }
              n69 = Select(t=myRIO_BRig_RT__Case_NonExp_stateList."UploadSettings_dataLC_1", s=w188, f=myRIO_BRig_RT__Case_NonExp_stateList."UploadSettings_Read_dataMTrig" ("t")) -> (s? t:f=w183:T1)
            }
            frame "UploadSettings_Read_dataMTrig" {
              # "grab dataMTrig and\nstore it in the\ngeneric data array"
              # "dataMTrig"
              n70 = call "myRIO_BRig_RT_dataMTrig_init_details.vi"() -> ("output_dataSize"=w208:i32, "output_dataName"=w211:string)  [unwired: 10 in]
              n71 = call "myRIO_BRig_RT_comm_webdav_uploadReceived_check.vi"("input_dataName"=w211) -> ("output_Iexist"=w210:bool, "output_dataPath"=w209:path)  [unwired: 9 in]
              n72 = case shown="True" w210 {
                tunnel: w209 -> [_ w220]
                tunnel: w208 -> [_ w219]
                tunnel: [_ w218] -> w207
                tunnel: w204 -> [w213 w217]
                tunnel: [w213 w214] -> w203
                frame False {
                }
                frame True {
                  n73 = call "myRIO_BRig_RT_comm_webdav_uploadReceived_read.vi"("input_dataSize"=w219, "input_filePath"=w220) -> ("output_Ivalid"=w218:bool, "output_data"=w216:i64[])  [unwired: 8 in]
                  n74 = To Unsigned Word Integer(number=w216) -> (unsigned 16bit integer=w215:u16[])
                  n75 = Select(t=w215, s=w218, f=w217) -> (s? t:f=w214:u16[])
                }
              }
              n76 = Select(t=myRIO_BRig_RT__Case_NonExp_stateList."UploadSettings_dataMTrig_1", s=w207, f=myRIO_BRig_RT__Case_NonExp_stateList."Idle" ("t")) -> (s? t:f=w202:T1)
            }
            frame "UploadSettings_dataExp_1" {
              w229 = 100.0 ("y")
              # "Freq"
              # "f_millisec2count"
              # "laser"
              # "Cue_max"
              # "Cue_min"
              # "CuePenalty"
              # "Timeout"
              # "Wrong"
              # "Selection"
              # "RewardPost"
              # "Reward_R"
              # "Reward_L"
              # "Tcycle"
              # "TPB_min_R"
              # "TPB_min_L"
              # "TPB_max_R"
              # "TPB_max_L"
              # "I_trialUntilReward"
              # "ENL_penalty"
              # "ENL_min"
              # "ENL_max"
              # "BUR_max"
              # "BUR_min"
              # "CueCycles"
              # "Audio_Freq_R"
              # "Audio_Freq_L"
              # "Audio_Amp_R"
              # "Audio_Amp_L"
              n77 = call "myRIO_BRig_RT_dataExp_FPGA_f_count2ms.vi"() -> ("output_FPGA_f_count2ms"=w243:i32)  [unwired: 11 in]
              n78 = call "myRIO_BRig_RT_dataExp_laser1_Freq.vi"() -> ("output_laser1_Freq"=w242:i32)  [unwired: 11 in]
              n79 = call "myRIO_BRig_RT_dataExp_CueCycles.vi"() -> ("output_CueCycles"=w289:i32)  [unwired: 11 in]
              n80 = call "myRIO_BRig_RT_dataExp_Audio_amp__R.vi"() -> ("output_Audio_amp__R"=w293:i32)  [unwired: 11 in]
              n81 = call "myRIO_BRig_RT_dataExp_Audio_amp__L.vi"() -> ("output_Audio_amp__L"=w295:i32)  [unwired: 11 in]
              n82 = call "myRIO_BRig_RT_dataExp_Tcycle_Reward__L.vi"() -> ("output_Tcycle_Reward__L"=w266:i32)  [unwired: 11 in]
              n83 = call "myRIO_BRig_RT_dataExp_Tcycle_Reward__R.vi"() -> ("output_Tcycle_Reward__R"=w265:i32)  [unwired: 11 in]
              n84 = call "myRIO_BRig_RT_dataExp_Tcycle_RewardPost.vi"() -> ("output_Tcycle_RewardPost"=w264:i32)  [unwired: 11 in]
              n85 = call "myRIO_BRig_RT_dataExp_BUR_min.vi"() -> ("output_BUR_min"=w286:i32)  [unwired: 11 in]
              n86 = call "myRIO_BRig_RT_dataExp_ENL_min.vi"() -> ("output_ENL_min"=w282:i32)  [unwired: 11 in]
              n87 = call "myRIO_BRig_RT_dataExp_TPB_max__L.vi"() -> ("output_TPB_max__L"=w274:i32)  [unwired: 11 in]
              n88 = call "myRIO_BRig_RT_dataExp_TPB_max__R.vi"() -> ("output_TPB_max__R"=w273:i32)  [unwired: 11 in]
              n89 = call "myRIO_BRig_RT_dataExp_ENL_penalty.vi"() -> ("output_ENL_penalty"=w281:i32)  [unwired: 11 in]
              n90 = call "myRIO_BRig_RT_dataExp_laser1_Power_min.vi"() -> ("output_laser1_Power_min"=w241:i32)  [unwired: 11 in]
              n91 = call "myRIO_BRig_RT_dataExp_laser1_Tpeak.vi"() -> ("output_laser1_Tpeak"=w240:i32)  [unwired: 11 in]
              n92 = call "myRIO_BRig_RT_dataExp_Audio_freq__L.vi"() -> ("output_Audio_freq__L"=w291:i32)  [unwired: 11 in]
              n93 = call "myRIO_BRig_RT_dataExp_Audio_freq__R.vi"() -> ("output_Audio_freq__R"=w290:i32)  [unwired: 11 in]
              n94 = call "myRIO_BRig_RT_dataExp_BUR_max.vi"() -> ("output_BUR_max"=w287:i32)  [unwired: 11 in]
              n95 = call "myRIO_BRig_RT_dataExp_ENL_max.vi"() -> ("output_ENL_max"=w283:i32)  [unwired: 11 in]
              n96 = call "myRIO_BRig_RT_dataExp_ItrialUntilReward.vi"() -> ("output_I_trialUntilReward"=w277:i32)  [unwired: 11 in]
              n97 = call "myRIO_BRig_RT_dataExp_Tcycle_Selection.vi"() -> ("output_Tcycle_Selection"=w263:i32)  [unwired: 11 in]
              n98 = call "myRIO_BRig_RT_dataExp_Tcycle_Wrong.vi"() -> ("output_Tcycle_Wrong"=w262:i32)  [unwired: 11 in]
              n99 = call "myRIO_BRig_RT_dataExp_Tcycle_Timeout.vi"() -> ("output_Tcycle_Timeout"=w261:i32)  [unwired: 11 in]
              n100 = call "myRIO_BRig_RT_dataExp_TPB_min__L.vi"() -> ("output_TPB_min__L"=w272:i32)  [unwired: 11 in]
              n101 = call "myRIO_BRig_RT_dataExp_TPB_min__R.vi"() -> ("output_TPB_min__R"=w271:i32)  [unwired: 11 in]
              n102 = call "myRIO_BRig_RT_dataExp_laser1_Tshutter.vi"() -> ("output_laser1_Tshutter"=w239:i32)  [unwired: 11 in]
              n103 = call "myRIO_BRig_RT_dataExp_laser1_duration.vi"() -> ("output_laser1_duration"=w238:i32)  [unwired: 11 in]
              n104 = call "myRIO_BRig_RT_dataExp_Tcycle_CuePenalty.vi"() -> ("output_Tcycle_CuePenalty"=w254:i32)  [unwired: 11 in]
              n105 = call "myRIO_BRig_RT_dataExp_Tcycle_Cue_min.vi"() -> ("output_Tcycle_Cue_min"=w253:i32)  [unwired: 11 in]
              n106 = call "myRIO_BRig_RT_dataExp_Tcycle_Cue_max.vi"() -> ("output_Tcycle_Cue_max"=w252:i32)  [unwired: 11 in]
              n107 = Index Array(array=w246, index #1=w295, index #2=w293, index #3=w291, index #4=w290, index #5=w289, index #6=w287, index #7=w286, index #8=w283, index #9=w282, index #10=w281, index #11=w277, index #12=w274, index #13=w273, index #14=w272, index #15=w271, index #16=w266, index #17=w265, index #18=w264, index #19=w263, index #20=w262, index #21=w261, index #22=w254, index #23=w253, index #24=w252, index #25=w243, index #26=w242, index #27=w241, index #28=w240, index #29=w239, index #30=w238) -> (element #1=w294:u16, element #2=w292:u16, element #3=w249:u16, element #4=w248:u16, element #5=w288:u16, element #6=w285:u16, element #7=w284:u16, element #8=w280:u16, element #9=w279:u16, element #10=w278:u16, element #11=w275:u16, element #12=w270:u16, element #13=w269:u16, element #14=w268:u16, element #15=w267:u16, element #16=w260:u16, element #17=w259:u16, element #18=w258:u16, element #19=w257:u16, element #20=w256:u16, element #21=w255:u16, element #22=w251:u16, element #23=w245:u16, element #24=w244:u16, element #25=w237:u16, element #26=w228:u16, element #27=w227:u16, element #28=w226:u16, element #29=w225:u16, element #30=w221:u16)
              n108 = To Double Precision Float(number=w237) -> (double precision float=w236:dbl)
              n109 = To Double Precision Float(number=w228) -> (double precision float=w234:dbl)
              n110 = To Double Precision Float(number=w227) -> (double precision float=w232:dbl)
              n111 = To Double Precision Float(number=w226) -> (double precision float=w231:dbl)
              n112 = To Double Precision Float(number=w225) -> (double precision float=w230:dbl)
              n113 = local write "Tcycle_Selection"(w257) -> ()
              n114 = local write "Tcycle_Wrong"(w256) -> ()
              n115 = local write "Tcycle_Timeout"(w255) -> ()
              n116 = local write "Audio_Amp__L"(w294) -> ()
              n117 = local write "Audio_Amp__R"(w292) -> ()
              n118 = Divide(x=w236, y=w229) -> (x/y=w235:dbl)
              n119 = Divide(x=w234, y=w229) -> (x/y=w233:dbl)
              n120 = Divide(x=w232, y=w229) -> (x/y=w224:dbl)
              n121 = Divide(x=w231, y=w229) -> (x/y=w223:dbl)
              n122 = Divide(x=w230, y=w229) -> (x/y=w222:dbl)
              n123 = local write "Tcycle_ENLPenalty"(w278) -> ()
              n124 = local write "Tcycle_ENL_max"(w280) -> ()
              n125 = local write "laser1_duration"(w221) -> ()
              n126 = local write "laser1_power_min"(w224) -> ()
              n127 = local write "TpB_Min_L"(w268) -> ()
              n128 = local write "TpB_Min_R"(w267) -> ()
              n129 = local write "FPGA_count2ms"(w235) -> ()
              n130 = local write "laser1_Tshutter"(w222) -> ()
              n131 = local write "laser1_Tpeak"(w223) -> ()
              n132 = local write "laser1_Freq"(w233) -> ()
              n133 = local write "Tcycle_CuePenalty"(w251) -> ()
              n134 = local write "Tcycle_Cue_min"(w245) -> ()
              n135 = local write "Tcycle_Cue_max"(w244) -> ()
              n136 = To Unsigned Byte Integer(number=w249) -> (unsigned 8bit integer=w250:u8)
              n137 = To Unsigned Byte Integer(number=w248) -> (unsigned 8bit integer=w247:u8)
              n138 = Not Equal To 0?(x=w275) -> (x != 0?=w276:bool)
              n139 = local write "Tcycle_Reward_L"(w260) -> ()
              n140 = local write "Tcycle_Reward_R"(w259) -> ()
              n141 = local write "Tcycle_RewardPost"(w258) -> ()
              n142 = local write "CueCycles"(w288) -> ()
              n143 = local write "BUR_min"(w284) -> ()
              n144 = local write "BUR_max"(w285) -> ()
              n145 = local write "Tcycle_ENL_min"(w279) -> ()
              n146 = local write "TpB_Max_L"(w270) -> ()
              n147 = local write "TpB_Max_R"(w269) -> ()
              n148 = local write "TrialUntilReward"(w276) -> ()
              n149 = local write "Audio_Freq__L"(w250) -> ()
              n150 = local write "Audio_Freq__R"(w247) -> ()
            }
            frame "UploadSettings_dataLC_1" {
              # "Cue1_All_delayOpt"
              # "ENL1_All_delayOpt"
              # "Cue1_First_delayOpt"
              # "ENL1_First_delayOpt"
              # "ENL1 First"
              # "Cue1 All"
              # "Cue1 First"
              # "Count"
              # "Tdelay"
              # "Prob"
              # "OnOff"
              # "Block"
              # "ENL1 All"
              # "Count"
              # "Tdelay"
              # "Prob"
              # "OnOff"
              # "Block"
              # "Count"
              # "Tdelay"
              # "Prob"
              # "Block"
              # "OnOff"
              # "Count"
              # "Tdelay"
              # "Prob"
              # "OnOff"
              # "Block"
              n151 = call "myRIO_BRig_RT_dataLC_Cue1_Block_Switch_l1.vi"() -> ("output_Cue1_Block_Switch_l1"=w354:i32)  [unwired: 11 in]
              n152 = call "myRIO_BRig_RT_dataLC_Cue1_OnOff_Switch_l1.vi"() -> ("output_Cue1_OnOff_Switch_l1"=w352:i32)  [unwired: 11 in]
              n153 = call "myRIO_BRig_RT_dataLC_Cue1_Count_Switch_l1.vi"() -> ("output_Cue1_Count_Switch_l1"=w349:i32)  [unwired: 11 in]
              n154 = call "myRIO_BRig_RT_dataLC_Cue1_Block_NS_l1.vi"() -> ("output_Cue1_Block_NS_l1"=w336:i32)  [unwired: 11 in]
              n155 = call "myRIO_BRig_RT_dataLC_Cue1_OnOff_NS_l1.vi"() -> ("output_Cue1_OnOff_NS_l1"=w335:i32)  [unwired: 11 in]
              n156 = call "myRIO_BRig_RT_dataLC_Cue1_Count_NS_l1.vi"() -> ("output_Cue1_Count_NS_l1"=w346:i32)  [unwired: 11 in]
              n157 = call "myRIO_BRig_RT_dataLC_ENL1_Block_Switch_l1.vi"() -> ("output_ENL1_Block_Switch_l1"=w334:i32)  [unwired: 11 in]
              n158 = call "myRIO_BRig_RT_dataLC_ENL1_OnOff_Switch_l1.vi"() -> ("output_ENL1_OnOff_Switch_l1"=w345:i32)  [unwired: 11 in]
              n159 = call "myRIO_BRig_RT_dataLC_ENL1_Count_Switch_l1.vi"() -> ("output_ENL1_Count_Switch_l1"=w342:i32)  [unwired: 11 in]
              n160 = call "myRIO_BRig_RT_dataLC_ENL1_Block_NS_l1.vi"() -> ("output_ENL1_All_Block"=w341:i32)  [unwired: 11 in]
              n161 = call "myRIO_BRig_RT_dataLC_ENL1_OnOff_NS_l1.vi"() -> ("output_ENL1_OnOff_NS_l1"=w340:i32)  [unwired: 11 in]
              n162 = call "myRIO_BRig_RT_dataLC_ENL1_Count_NS_l1.vi"() -> ("output_ENL1_Count_NS_l1"=w337:i32)  [unwired: 11 in]
              n163 = call "myRIO_BRig_RT_dataLC_ENL1_delayOpt_Switch_l1.vi"() -> ("output_ENL1_delayOpt_Switch_l1"=w311:i32)  [unwired: 11 in]
              n164 = call "myRIO_BRig_RT_dataLC_Cue1_delayOpt_Switch_l1.vi"() -> ("output_Cue1_delayOpt_Switch_l1"=w310:i32)  [unwired: 11 in]
              n165 = call "myRIO_BRig_RT_dataLC_ENL1_delayOpt_NS_l1.vi"() -> ("output_ENL1_delayOpt_NS_l1"=w303:i32)  [unwired: 11 in]
              n166 = call "myRIO_BRig_RT_dataLC_Cue1_delayOpt_NS_l1.vi"() -> ("output_Cue1_delayOpt_NS_l1"=w302:i32)  [unwired: 11 in]
              n167 = call "myRIO_BRig_RT_dataLC_Cue1_Probability_Switch_l1.vi"() -> ("output_Cue1_Probability_Switch_l1"=w351:i32)  [unwired: 11 in]
              n168 = call "myRIO_BRig_RT_dataLC_Cue1_Tdelay_Switch_l1.vi"() -> ("output_Cue1_Tdelay_Switch_l1"=w350:i32)  [unwired: 11 in]
              n169 = call "myRIO_BRig_RT_dataLC_Cue1_Probability_NS_l1.vi"() -> ("output_Cue1_l1_All_Probability"=w348:i32)  [unwired: 11 in]
              n170 = call "myRIO_BRig_RT_dataLC_Cue1_Tdelay_NS_l1.vi"() -> ("output_Cue1_Tdelay_NS_l1"=w347:i32)  [unwired: 11 in]
              n171 = call "myRIO_BRig_RT_dataLC_ENL1_Probability_Switch_l1.vi"() -> ("output_ENL1_Probability_Switch_l1"=w344:i32)  [unwired: 11 in]
              n172 = call "myRIO_BRig_RT_dataLC_ENL1_Tdelay_Switch_l1.vi"() -> ("output_ENL1_Tdelay_Switch_l1"=w343:i32)  [unwired: 11 in]
              n173 = call "myRIO_BRig_RT_dataLC_ENL1_Probability_NS_l1.vi"() -> ("output_ENL1_Probability_NS_l1"=w339:i32)  [unwired: 11 in]
              n174 = call "myRIO_BRig_RT_dataLC_ENL1_Tdelay_NS_l1.vi"() -> ("output_ENL1_Tdelay_NS_l1"=w338:i32)  [unwired: 11 in]
              n175 = Index Array(array=w312, index #1=w354, index #2=w352, index #3=w351, index #4=w350, index #5=w349, index #6=w336, index #7=w335, index #8=w348, index #9=w347, index #10=w346, index #11=w334, index #12=w345, index #13=w344, index #14=w343, index #15=w342, index #16=w341, index #17=w340, index #18=w339, index #19=w338, index #20=w337, index #21=w311, index #22=w310, index #23=w303, index #24=w302) -> (element #1=w353:u16, element #2=w332:u16, element #3=w331:u16, element #4=w330:u16, element #5=w329:u16, element #6=w325:u16, element #7=w324:u16, element #8=w323:u16, element #9=w322:u16, element #10=w321:u16, element #11=w320:u16, element #12=w319:u16, element #13=w318:u16, element #14=w317:u16, element #15=w304:u16, element #16=w316:u16, element #17=w315:u16, element #18=w314:u16, element #19=w313:u16, element #20=w305:u16, element #21=w308:u16, element #22=w306:u16, element #23=w299:u16, element #24=w298:u16)
              n176 = Not Equal To 0?(x=w299) -> (x != 0?=w301:bool)
              n177 = Not Equal To 0?(x=w298) -> (x != 0?=w300:bool)
              n178 = Not Equal To 0?(x=w308) -> (x != 0?=w309:bool)
              n179 = Not Equal To 0?(x=w306) -> (x != 0?=w307:bool)
              n180 = Not Equal To 0?(x=w332) -> (x != 0?=w333:bool)
              n181 = local write "LC_l1_Cue1_First_Probability"(w331) -> ()
              n182 = Not Equal To 0?(x=w324) -> (x != 0?=w328:bool)
              n183 = Not Equal To 0?(x=w319) -> (x != 0?=w327:bool)
              n184 = Not Equal To 0?(x=w315) -> (x != 0?=w326:bool)
              n185 = local write "LC_l1_ENL1_First_Probability"(w318) -> ()
              n186 = local write "LC_l1_ENL1_First_delayOpt"(w309) -> ()
              n187 = local write "LC_l1_Cue1_First_delayOpt"(w307) -> ()
              n188 = local write "LC_l1_ENL1_All_delayOpt"(w301) -> ()
              n189 = local write "LC_l1_Cue1_All_delayOpt"(w300) -> ()
              n190 = local write "LC_l1_Cue1_All_Probability"(w323) -> ()
              n191 = local write "LC_l1_Cue1_First_Tdelay"(w330) -> ()
              n192 = local write "LC_l1_ENL1_All_Probability"(w314) -> ()
              n193 = local write "LC_l1_Cue1_First_OnOff"(w333) -> ()
              n194 = local write "LC_l1_Cue1_First_Count"(w329) -> ()
              n195 = local write "LC_l1_Cue1_First_Block"(w353) -> ()
              n196 = local write "LC_l1_ENL1_First_Tdelay"(w317) -> ()
              n197 = local write "LC_l1_ENL1_First_OnOff"(w327) -> ()
              n198 = local write "LC_l1_ENL1_First_Count"(w304) -> ()
              n199 = local write "LC_l1_ENL1_First_Block"(w320) -> ()
              n200 = local write "LC_l1_Cue1_All_Tdelay"(w322) -> ()
              n201 = local write "LC_l1_Cue1_All_OnOff"(w328) -> ()
              n202 = local write "LC_l1_Cue1_All_Count"(w321) -> ()
              n203 = local write "LC_l1_Cue1_All_Block"(w325) -> ()
              n204 = local write "LC_l1_ENL1_All_Tdelay"(w313) -> ()
              n205 = local write "LC_l1_ENL1_All_OnOff"(w326) -> ()
              n206 = local write "LC_l1_ENL1_All_Count"(w305) -> ()
              n207 = local write "LC_l1_ENL1_All_Block"(w316) -> ()
            }
            frame "UploadSettings_dataLC_2" {
              # "Wrong"
              # "Reward"
              # "Trial"
              # "Tdelay"
              # "Prob"
              # "Block"
              # "OnOff"
              # "Trial"
              # "Tdelay"
              # "Prob"
              # "OnOff"
              # "Block"
              n208 = call "myRIO_BRig_RT_dataLC_Reward_Block_l1.vi"() -> ("output_Reward_Block_l1"=w379:i32)  [unwired: 11 in]
              n209 = call "myRIO_BRig_RT_dataLC_Reward_OnOff_l1.vi"() -> ("output_Reward_OnOff_l1"=w377:i32)  [unwired: 11 in]
              n210 = call "myRIO_BRig_RT_dataLC_Reward_Trial_l1.vi"() -> ("output_Reward_Trial_l1"=w374:i32)  [unwired: 11 in]
              n211 = call "myRIO_BRig_RT_dataLC_Wrong_Block_l1.vi"() -> ("output_Wrong_Block_l1"=w370:i32)  [unwired: 11 in]
              n212 = call "myRIO_BRig_RT_dataLC_Wrong_OnOff_l1.vi"() -> ("output_Wrong_OnOff_l1"=w369:i32)  [unwired: 11 in]
              n213 = call "myRIO_BRig_RT_dataLC_Wrong_Trial_l1.vi"() -> ("output_Wrong_Trial_l1"=w371:i32)  [unwired: 11 in]
              n214 = call "myRIO_BRig_RT_dataLC_Reward_Probability_l1.vi"() -> ("output_Reward_Probability_l1"=w376:i32)  [unwired: 11 in]
              n215 = call "myRIO_BRig_RT_dataLC_Reward_Tdelay_l1.vi"() -> ("output_Reward_Tdelay_l1"=w375:i32)  [unwired: 11 in]
              n216 = call "myRIO_BRig_RT_dataLC_Wrong_Probability_l1.vi"() -> ("output_Wrong_Probability_l1"=w373:i32)  [unwired: 11 in]
              n217 = call "myRIO_BRig_RT_dataLC_Wrong_Tdelay_l1.vi"() -> ("output_Wrong_Tdelay_l1"=w372:i32)  [unwired: 11 in]
              n218 = Index Array(array=w357, index #1=w379, index #2=w377, index #3=w376, index #4=w375, index #5=w374, index #6=w370, index #7=w369, index #8=w373, index #9=w372, index #10=w371) -> (element #1=w378:u16, element #2=w367:u16, element #3=w366:u16, element #4=w365:u16, element #5=w364:u16, element #6=w362:u16, element #7=w361:u16, element #8=w360:u16, element #9=w359:u16, element #10=w358:u16)
              n219 = Not Equal To 0?(x=w367) -> (x != 0?=w368:bool)
              n220 = Not Equal To 0?(x=w361) -> (x != 0?=w363:bool)
              n221 = local write "LC_l1_Reward_Probability"(w366) -> ()
              n222 = local write "LC_l1_Wrong_Probability"(w360) -> ()
              n223 = local write "LC_l1_Reward_Tdelay"(w365) -> ()
              n224 = local write "LC_l1_Reward_OnOff"(w368) -> ()
              n225 = local write "LC_l1_Reward_Block"(w378) -> ()
              n226 = local write "LC_l1_Reward_Trial"(w364) -> ()
              n227 = local write "LC_l1_Wrong_Tdelay"(w359) -> ()
              n228 = local write "LC_l1_Wrong_OnOff"(w363) -> ()
              n229 = local write "LC_l1_Wrong_Block"(w362) -> ()
              n230 = local write "LC_l1_Wrong_Trial"(w358) -> ()
            }
            frame "UploadSettings_dataMTrig_1" {
              # "Tdelay_R"
              # "Tdelay_L"
              # "Tcycle_R"
              # "Tcycle_L"
              # "RewCalib_nCycle_R"
              # "RewCalib_nCycle_L"
              # "Solenoid"
              # "Laser_Tcycle"
              n231 = call "myRIO_BRig_RT_dataMTrig_Laser_Tcycle.vi"() -> ("output_Laser_Tcycle"=w389:i32)  [unwired: 11 in]
              n232 = call "myRIO_BRig_RT_dataMTrig_Solenoid_RewCalib_nCycle__L.vi"() -> ("output_Solenoid_RewCalib_nCycle__L"=w388:i32)  [unwired: 11 in]
              n233 = call "myRIO_BRig_RT_dataMTrig_Solenoid_RewCalib_nCycle__R.vi"() -> ("output_Solenoid_RewCalib_nCycle__R"=w387:i32)  [unwired: 11 in]
              n234 = call "myRIO_BRig_RT_dataMTrig_Solenoid_Tdelay__L.vi"() -> ("output_Solenoid_Tdelay__L"=w384:i32)  [unwired: 11 in]
              n235 = call "myRIO_BRig_RT_dataMTrig_Solenoid_Tdelay__R.vi"() -> ("output_Solenoid_Tdelay__R"=w383:i32)  [unwired: 11 in]
              n236 = call "myRIO_BRig_RT_dataMTrig_Solenoid_Tcycle__L.vi"() -> ("output_Solenoid_Tcycle__L"=w386:i32)  [unwired: 11 in]
              n237 = call "myRIO_BRig_RT_dataMTrig_Solenoid_Tcycle__R.vi"() -> ("output_Solenoid_Tcycle__R"=w385:i32)  [unwired: 11 in]
              n238 = Index Array(array=w382, index #1=w389, index #2=w388, index #3=w387, index #4=w386, index #5=w385, index #6=w384, index #7=w383) -> (element #1=w396:u16, element #2=w395:u16, element #3=w394:u16, element #4=w393:u16, element #5=w392:u16, element #6=w391:u16, element #7=w390:u16)
              n239 = Replace Array Subset(array=w398, new element #1=w396, index #1=w389, new element #2=w395, index #2=w388, new element #3=w394, index #3=w387, new element #4=w393, index #4=w386, new element #5=w392, index #5=w385, new element #6=w391, index #6=w384, new element #7=w390, index #7=w383) -> (w397:u16[])
              n240 = local write "MTrig_Solenoid_Tcycle__L"(w393) -> ()
              n241 = local write "MTrig_Solenoid_Tcycle__R"(w392) -> ()
              n242 = local write "MTrig_Laser_Tcycle"(w396) -> ()
            }
            frame "Idle" {
              # "To ensure timing, we split the\nidle state into 4 phases"
              # "Laser_Tcycle"
              # "Audio_Tcycle_R"
              # "Audio_Tcycle_L"
              n243 = local read "laser1_power_min"() -> (w401:dbl)
              n244 = local read "FPGA_count2ms"() -> (w409:dbl)
              n245 = local read "Audio_Amp__R"() -> (w403:u16)
              n246 = local read "Audio_Amp__L"() -> (w405:u16)
              n247 = local read "Audio_Freq__R"() -> (w402:u8)
              n248 = local read "Audio_Freq__L"() -> (w404:u8)
              n249 = local read "MTrig_Audio_trig__L"() -> (w417:bool)
              n250 = local read "MTrig_Audio_trig__R"() -> (w419:bool)
              n251 = Select(t=myRIO_BRig_RT__Case_NonExp_stateList."SendData" ("Enum"), s="SendData", f=myRIO_BRig_RT__Case_NonExp_stateList."Idle_2" ("Enum")) -> (s? t:f=w412:T1)
              n252 = call "myRIO__convert__Voltage_to_FPGAvalue.vi"("input_voltage"=w401) -> ("output_PortC"=w400:i16)  [unwired: 9 in, 1 out]
              n253 = local read "MTrig_Laser_trig"() -> (w418:bool)
              n254 = To Unsigned Word Integer(number=w409) -> (unsigned 16bit integer=w408:u16)
              n255 = call "myRIO_BRig_RT_dataMTrig_Audio_Tcycle__L.vi"() -> ("output_Audio_Tcycle__L"=w428:i32)  [unwired: 11 in]
              n256 = call "myRIO_BRig_RT_dataMTrig_Audio_Tcycle__R.vi"() -> ("output_Audio_Tcycle__R"=w427:i32)  [unwired: 11 in]
              n257 = call "myRIO_BRig_RT_dataMTrig_Laser_Tcycle.vi"() -> ("output_Laser_Tcycle"=w426:i32)  [unwired: 11 in]
              n258 = local read "MTrig_Laser_Tcycle"() -> (w410:u16)
              n259 = xnode "Read/Write Control"("FPGA VI Reference In"=w407, "error in"=w406, "k1__counter_per_ms"=w408, "audioAmp_L"=w405, "audioFreq_L_kHz"=w404, "audioAmp_R"=w403, "audioFreq_R_kHz"=w402, "AnaOut_0"=w400) -> ()  [unwired: 2 out]
              n260 = Select(t=myRIO_BRig_RT__Case_NonExp_stateList."TestConnection" ("Enum"), s="TestConnection", f=w412) -> (s? t:f=w421:T1)
              n261 = local read "Tcycle_Cue_min"() -> (w411:u16)
              n262 = Compound Arithmetic op=OR(w417, w419, w418) -> (w420:bool)
              n263 = case shown="True" w420 {
                frame False {
                }
                frame True {
                  w429 = FALSE
                  n264 = local write "MTrig_Audio_trig__L"(w429) -> ()
                  n265 = local write "MTrig_Audio_trig__R"(w429) -> ()
                  n266 = local write "MTrig_Laser_trig"(w429) -> ()
                }
              }
              n267 = Replace Array Subset(array=w424, new element #1=w411, index #1=w428, new element #2=w411, index #2=w427, new element #3=w410, index #3=w426) -> (w425:u16[])
            }
            frame "Idle_2" {
              w431 = u16 0 ("t")
              # "To ensure timing, we split the\nidle state into 4 phases"
              # "Ncycles"
              # "Ncycles"
              # "RewCalib"
              # "RewCalib"
              # "Solenoid R"
              # "Solenoid L"
              n268 = call "myRIO_BRig_RT_dataMTrig_Solenoid_RewCalib_OnOff__L.vi"() -> ("output_Solenoid_RewCalib_OnOff__L"=w462:i32)  [unwired: 11 in]
              n269 = call "myRIO_BRig_RT_dataMTrig_Solenoid_N__L.vi"() -> ("output_Solenoid_N__L"=w450:i32)  [unwired: 11 in]
              n270 = call "myRIO_BRig_RT_dataMTrig_Solenoid_RewCalib_OnOff__R.vi"() -> ("output_Solenoid_RewCalib_OnOff__R"=w447:i32)  [unwired: 11 in]
              n271 = call "myRIO_BRig_RT_dataMTrig_Solenoid_N__R.vi"() -> ("output_Solenoid_N__R"=w446:i32)  [unwired: 11 in]
              n272 = Index Array(array=w453, index #1=w462, index #2=w450, index #3=w447, index #4=w446) -> (element #1=w449:u16, element #2=w444:u16, element #3=w445:u16, element #4=w443:u16)
              n273 = local read "RewCalib_Trig_L"() -> (w442:bool)
              n274 = local read "RewCalib_Trig_R"() -> (w441:bool)
              n275 = Equal To 0?(x=w444) -> (x = 0?=w452:bool)
              n276 = Equal To 0?(x=w443) -> (x = 0?=w451:bool)
              n277 = Not Equal To 0?(x=w445) -> (x != 0?=w463:bool)
              n278 = Not Equal To 0?(x=w449) -> (x != 0?=w464:bool)
              n279 = And(x=w452, y=w451) -> (x .and. y?=w456:bool)
              n280 = Or(x=w442, y=w441) -> (x .or. y?=w457:bool)
              n281 = Not Exclusive Or(1:w464, 2:w442) -> (0:w459:bool)
              n282 = Not Exclusive Or(1:w463, 2:w441) -> (0:w461:bool)
              n283 = And(x=w457, y=w456) -> (x .and. y?=w439:bool)
              n284 = Not(x=w459) -> (.not. x?=w458:bool)
              n285 = Not(x=w461) -> (.not. x?=w460:bool)
              n286 = Or(x=w458, y=w460) -> (x .or. y?=w440:bool)
              n287 = Or(x=w439, y=w440) -> (x .or. y?=w455:bool)
              n288 = local read "count_warmup_R"() -> (w430:u16)
              n289 = local read "count_warmup_L"() -> (w435:u16)
              n290 = Select(t=myRIO_BRig_RT__Case_NonExp_stateList."RewardCalibration_pre" ("Enum"), s=w455, f=myRIO_BRig_RT__Case_NonExp_stateList."Idle_3" ("Enum")) -> (s? t:f=w438:T1)
              n291 = Select(t=w431, s="count_warmup_L_reset", f=w435) -> (s? t:f=→"count_warmup_L":u16)
              n292 = Select(t=w431, s="count_warmup_R_reset", f=w430) -> (s? t:f=→"count_warmup_R":u16)
            }
            frame "Idle_3" {
              w487 = u8 0 ("f")
              # "To ensure timing, we split the\nidle state into 4 phases"
              n293 = local read "MTrig_Solenoid_trig__L"() -> (w478:bool)
              n294 = local read "MTrig_Solenoid_trig__R"() -> (w488:bool)
              n295 = local read "warmupType"() -> (w470:u8)
              n296 = local read "warmup"() -> (w480:bool)
              n297 = Not Equal To 0?(x=w470) -> (x != 0?=w469:bool)
              n298 = Not(x=w469) -> (.not. x?=w481:bool)
              n299 = Select(t=u8 1, s=w478, f=w487) -> (s? t:f=w486:u8)
              n300 = Select(t=u8 2, s=w488, f=w487) -> (s? t:f=w485:u8)
              n301 = And(x=w480, y=w481) -> (x .and. y?=w479:bool)
              n302 = And(x=w480, y=w469) -> (x .and. y?=w474:bool)
              n303 = Add(x=w486, y=w485) -> (x+y=w484:u8)
              n304 = case shown="3" w484 {
                tunnel: w483 -> [w491 w495 w513 w531]
                tunnel: [w491 w494 w512 w530] -> w482
                tunnel: w479 -> [_ w493 w511 w529]
                tunnel: [_ TRUE TRUE TRUE] -> w476
                frame 0, Default {
                }
                frame 1 {
                  n305 = case shown="True" w493 {
                    tunnel: w495 -> [w504 w509]
                    tunnel: [w503 w508] -> w494
                    frame True {
                      # "Audio_L"
                      # "Solenoid_L"
                      n306 = call "myRIO_BRig_RT_dataMTrig_Solenoid_N__L.vi"() -> ("output_Solenoid_N__L"=w500:i32)  [unwired: 11 in]
                      n307 = call "myRIO_BRig_RT_dataMTrig_Audio_N__L.vi"() -> ("output_Audio_N__L"=w498:i32)  [unwired: 11 in]
                      n308 = Index Array(array=w504, index #1=w500, index #2=w498) -> (element #1=w502:u16, element #2=w501:u16)
                      n309 = Increment(x=w502) -> (x+1=w499:u16)
                      n310 = Increment(x=w501) -> (x+1=w497:u16)
                      n311 = Replace Array Subset(array=w504, new element #1=w499, index #1=w500, new element #2=w497, index #2=w498) -> (w503:u16[])
                    }
                    frame False {
                      # "Solenoid_L"
                      n312 = call "myRIO_BRig_RT_dataMTrig_Solenoid_N__L.vi"() -> ("output_Solenoid_N__L"=w506:i32)  [unwired: 11 in]
                      n313 = Index Array(array=w509, index=w506) -> (element=w507:u16)
                      n314 = Increment(x=w507) -> (x+1=w505:u16)
                      n315 = Replace Array Subset(array=w509, new element=w505, index=w506) -> (w508:u16[])
                    }
                  }
                  n316 = local write "MTrig_Solenoid_trig__L"(FALSE) -> ()
                }
                frame 2 {
                  n317 = case shown="True" w511 {
                    tunnel: w513 -> [w522 w527]
                    tunnel: [w521 w526] -> w512
                    frame True {
                      # "Audio_R"
                      # "Solenoid_R"
                      n318 = call "myRIO_BRig_RT_dataMTrig_Solenoid_N__R.vi"() -> ("output_Solenoid_N__R"=w518:i32)  [unwired: 11 in]
                      n319 = call "myRIO_BRig_RT_dataMTrig_Audio_N__R.vi"() -> ("output_Audio_N__R"=w517:i32)  [unwired: 11 in]
                      n320 = Index Array(array=w522, index #1=w518, index #2=w517) -> (element #1=w520:u16, element #2=w519:u16)
                      n321 = Increment(x=w519) -> (x+1=w515:u16)
                      n322 = Increment(x=w520) -> (x+1=w516:u16)
                      n323 = Replace Array Subset(array=w522, new element #1=w516, index #1=w518, new element #2=w515, index #2=w517) -> (w521:u16[])
                    }
                    frame False {
                      # "Solenoid_R"
                      n324 = call "myRIO_BRig_RT_dataMTrig_Solenoid_N__R.vi"() -> ("output_Solenoid_N__R"=w523:i32)  [unwired: 11 in]
                      n325 = Index Array(array=w527, index=w523) -> (element=w525:u16)
                      n326 = Increment(x=w525) -> (x+1=w524:u16)
                      n327 = Replace Array Subset(array=w527, new element=w524, index=w523) -> (w526:u16[])
                    }
                  }
                  n328 = local write "MTrig_Solenoid_trig__R"(FALSE) -> ()
                }
                frame 3 {
                  w532 = FALSE
                  n329 = case shown="True" w529 {
                    tunnel: w531 -> [w546 w554]
                    tunnel: [w545 w553] -> w530
                    frame True {
                      # "Audio_R"
                      # "Solenoid_R"
                      # "Audio_L"
                      # "Solenoid_L"
                      n330 = call "myRIO_BRig_RT_dataMTrig_Solenoid_N__L.vi"() -> ("output_Solenoid_N__L"=w540:i32)  [unwired: 11 in]
                      n331 = call "myRIO_BRig_RT_dataMTrig_Audio_N__L.vi"() -> ("output_Audio_N__L"=w538:i32)  [unwired: 11 in]
                      n332 = call "myRIO_BRig_RT_dataMTrig_Solenoid_N__R.vi"() -> ("output_Solenoid_N__R"=w536:i32)  [unwired: 11 in]
                      n333 = call "myRIO_BRig_RT_dataMTrig_Audio_N__R.vi"() -> ("output_Audio_N__R"=w535:i32)  [unwired: 11 in]
                      n334 = Index Array(array=w546, index #1=w540, index #2=w538, index #3=w536, index #4=w535) -> (element #1=w544:u16, element #2=w543:u16, element #3=w542:u16, element #4=w541:u16)
                      n335 = Increment(x=w541) -> (x+1=w533:u16)
                      n336 = Increment(x=w544) -> (x+1=w539:u16)
                      n337 = Increment(x=w543) -> (x+1=w537:u16)
                      n338 = Increment(x=w542) -> (x+1=w534:u16)
                      n339 = Replace Array Subset(array=w546, new element #1=w539, index #1=w540, new element #2=w537, index #2=w538, new element #3=w534, index #3=w536, new element #4=w533, index #4=w535) -> (w545:u16[])
                    }
                    frame False {
                      # "Solenoid_R"
                      # "Solenoid_L"
                      n340 = call "myRIO_BRig_RT_dataMTrig_Solenoid_N__L.vi"() -> ("output_Solenoid_N__L"=w550:i32)  [unwired: 11 in]
                      n341 = call "myRIO_BRig_RT_dataMTrig_Solenoid_N__R.vi"() -> ("output_Solenoid_N__R"=w547:i32)  [unwired: 11 in]
                      n342 = Index Array(array=w554, index #1=w550, index #2=w547) -> (element #1=w552:u16, element #2=w551:u16)
                      n343 = Increment(x=w552) -> (x+1=w549:u16)
                      n344 = Increment(x=w551) -> (x+1=w548:u16)
                      n345 = Replace Array Subset(array=w554, new element #1=w549, index #1=w550, new element #2=w548, index #2=w547) -> (w553:u16[])
                    }
                  }
                  n346 = local write "MTrig_Solenoid_trig__L"(w532) -> ()
                  n347 = local write "MTrig_Solenoid_trig__R"(w532) -> ()
                }
              }
              n348 = local read "get_countPerMS"() -> (w468:bool)
              n349 = Select(t=myRIO_BRig_RT__Case_NonExp_stateList."Get_FPGA_count_per_ms" ("Enum"), s=w468, f=myRIO_BRig_RT__Case_NonExp_stateList."Idle_4" ("Enum")) -> (s? t:f=w466:T1)
              n350 = Select(t=myRIO_BRig_RT__Case_NonExp_stateList."Cue_pre", s=w474, f=myRIO_BRig_RT__Case_NonExp_stateList."DispenseWater_pre" ("Enum")) -> (s? t:f=w472:T1)
              n351 = Select(t=w472, s=w476, f=w466) -> (s? t:f=w477:T1)
            }
            frame "Idle_4" {
              # "use dataMTrig as it is one of the last to transfer"
              # "To ensure timing, we split the\nidle state into 4 phases"
              n352 = call "myRIO_BRig_RT_comm_webdav_uploadReceived_check_v2,0.vi"("input_dataName"="dataMTrig") -> ("output_Iexist"=w560:bool)  [unwired: 9 in, 1 out]
              n353 = Select(t=myRIO_BRig_RT__Case_NonExp_stateList."UploadSettings_pre" ("Enum"), s=w560, f=myRIO_BRig_RT__Case_NonExp_stateList."Idle") -> (s? t:f=w558:T1)
            }
            frame "Cue_pre" {
              w570 = u16 1 ("t")
              w569 = u16 0 ("new element/subarray")
              w566 = u16 0 ("new element/subarray")
              # "Ncycle"
              # "count"
              # "Audio_R"
              # "Solenoid_R"
              # "Solenoid_L"
              # "Ncycle"
              # "count"
              # "Audio_L"
              n354 = call "myRIO_BRig_RT_dataMTrig_Solenoid_N__L.vi"() -> ("output_Solenoid_N__L"=w579:i32)  [unwired: 11 in]
              n355 = call "myRIO_BRig_RT_dataMTrig_Solenoid_N__R.vi"() -> ("output_Solenoid_N__R"=w578:i32)  [unwired: 11 in]
              n356 = Index Array(array=w575, index #1=w579, index #2=w578) -> (element #1=w577:u16, element #2=w576:u16)
              n357 = Not Equal To 0?(x=w576) -> (x != 0?=w562:bool)
              n358 = Not Equal To 0?(x=w577) -> (x != 0?=w563:bool)
              n359 = Select(t=w570, s=w563, f=w569) -> (s? t:f=w571:u16)
              n360 = Select(t=w570, s=w562, f=w569) -> (s? t:f=w565:u16)
              n361 = call "myRIO_BRig_RT_dataMTrig_Audio_c__L.vi"() -> ("output_Audio_c__L"=w573:i32)  [unwired: 11 in]
              n362 = call "myRIO_BRig_RT_dataMTrig_Audio_N__L.vi"() -> ("output_Audio_N__L"=w572:i32)  [unwired: 11 in]
              n363 = call "myRIO_BRig_RT_dataMTrig_Audio_c__R.vi"() -> ("output_Audio_c__R"=w568:i32)  [unwired: 11 in]
              n364 = call "myRIO_BRig_RT_dataMTrig_Audio_N__R.vi"() -> ("output_Audio_N__R"=w567:i32)  [unwired: 11 in]
              n365 = Replace Array Subset(array=w575, new element #1=w566, index #1=w573, new element #2=w571, index #2=w572, new element #3=w566, index #3=w568, new element #4=w565, index #4=w567) -> (w574:u16[])
            }
            frame "Cue" {
              # "lick did not occur or warmupType==1"
              # "lick occurred?"
              # "Ncycle"
              # "Audio_R"
              # "Ncycle"
              # "Audio_L"
              n366 = local read "warmupType"() -> (w589:u8)
              n367 = Greater?(x=w595, y=w594) -> (0:w598:bool)
              n368 = Greater?(x=w597, y=w596) -> (0:w593:bool)
              n369 = Or(x=w593, y=w598) -> (x .or. y?=w587:bool)
              n370 = Equal?(x=w589, y=u8 1) -> (x = y?=w583:bool)
              n371 = Not(x=w587) -> (.not. x?=w586:bool)
              n372 = call "myRIO_BRig_RT_dataMTrig_Audio_N__L.vi"() -> ("output_Audio_N__L"=w601:i32)  [unwired: 11 in]
              n373 = call "myRIO_BRig_RT_dataMTrig_Audio_N__R.vi"() -> ("output_Audio_N__R"=w600:i32)  [unwired: 11 in]
              n374 = Or(x=w586, y=w583) -> (x .or. y?=w584:bool)
              n375 = case shown="True" w584 {
                tunnel: w601 -> [w607 w625]
                tunnel: w600 -> [w606 w624]
                tunnel: w592 -> [w609 w619]
                tunnel: [w608 w619] -> w591
                tunnel: w590 -> [_ w617]
                tunnel: [myRIO_BRig_RT__Case_NonExp_stateList."Idle" ("t") w616] -> w585
                tunnel: w583 -> [_ w615]
                tunnel: w582 -> [_ w611]
                tunnel: w581 -> [_ w610]
                frame False {
                  w602 = u16 0 ("new element/subarray")
                  # "lick occurred and warmupType==2"
                  n376 = call "myRIO_BRig_RT_dataMTrig_Solenoid_N__R.vi"() -> ("output_Solenoid_N__R"=w603:i32)  [unwired: 11 in]
                  n377 = call "myRIO_BRig_RT_dataMTrig_Solenoid_N__L.vi"() -> ("output_Solenoid_N__L"=w604:i32)  [unwired: 11 in]
                  n378 = Replace Array Subset(array=w609, new element #1=w602, index #1=w607, new element #2=w602, index #2=w606, new element #3=w602, index #3=w604, new element #4=w602, index #4=w603) -> (w608:u16[])
                }
                frame True {
                  n379 = Not(x=w615) -> (.not. x?=w614:bool)
                  n380 = Index Array(array=w619, index #1=w625, index #2=w624) -> (element #1=w623:u16, element #2=w622:u16)
                  n381 = Equal To 0?(x=w623) -> (x = 0?=w621:bool)
                  n382 = Equal To 0?(x=w622) -> (x = 0?=w620:bool)
                  n383 = And(x=w621, y=w620) -> (x .and. y?=w613:bool)
                  n384 = And(x=w613, y=w614) -> (x .and. y?=w612:bool)
                  n385 = case shown="True" w612 {
                    tunnel: w611 -> [_ w633]
                    tunnel: w610 -> [_ w628]
                    frame False {
                    }
                    frame True {
                      n386 = local read "count_warmup_R"() -> (w626:u16)
                      n387 = local read "count_warmup_L"() -> (w631:u16)
                      n388 = Increment(x=w626) -> (x+1=w629:u16)
                      n389 = Increment(x=w631) -> (x+1=w632:u16)
                      n390 = Select(t=w629, s=w628, f=w626) -> (s? t:f=w627:u16)
                      n391 = Select(t=w632, s=w633, f=w631) -> (s? t:f=w630:u16)
                      n392 = local write "count_warmup_R"(w627) -> ()
                      n393 = local write "count_warmup_L"(w630) -> ()
                    }
                  }
                  n394 = Select(t=myRIO_BRig_RT__Case_NonExp_stateList."DispenseWater_pre", s=w613, f=w617) -> (s? t:f=w616:T1)
                }
              }
            }
            frame "RewardCalibration_pre" {
              (unwired) FALSE
              w635 = FALSE
              w646 = u8 0
              w662 = u8 0
              # "Are we starting a RewardCalibration?\nOr are we stopping a RewardCalibration?\nOr is a RewardCalibration over?"
              # "RewCalib\nOnOff"
              # "N"
              # "Solenoid R"
              # "RewCalib\nOnOff"
              # "N"
              # "Solenoid L"
              n395 = local read "RewCalib_Trig_L"() -> (w669:bool)
              n396 = local read "RewCalib_Trig_R"() -> (w638:bool)
              n397 = call "myRIO_BRig_RT_dataMTrig_Solenoid_N__R.vi"() -> ("output_Solenoid_N__R"=w640:i32)  [unwired: 11 in]
              n398 = call "myRIO_BRig_RT_dataMTrig_Solenoid_RewCalib_OnOff__R.vi"() -> ("output_Solenoid_RewCalib_OnOff__R"=w637:i32)  [unwired: 11 in]
              n399 = call "myRIO_BRig_RT_dataMTrig_Solenoid_N__L.vi"() -> ("output_Solenoid_N__L"=w655:i32)  [unwired: 11 in]
              n400 = call "myRIO_BRig_RT_dataMTrig_Solenoid_RewCalib_OnOff__L.vi"() -> ("output_Solenoid_RewCalib_OnOff__L"=w656:i32)  [unwired: 11 in]
              n401 = Index Array(array=w639, index #1=w640, index #2=w637) -> (element #1=w650:u16, element #2=w645:u16)
              n402 = Index Array(array=w639, index #1=w655, index #2=w656) -> (element #1=w666:u16, element #2=w661:u16)
              n403 = Equal To 0?(x=w650) -> (x = 0?=w651:bool)
              n404 = Not Equal To 0?(x=w645) -> (x != 0?=w648:bool)
              n405 = Equal To 0?(x=w666) -> (x = 0?=w667:bool)
              n406 = Not Equal To 0?(x=w661) -> (x != 0?=w664:bool)
              n407 = local write "MTrig_Solenoid_trig__L"(w635) -> ()
              n408 = local write "MTrig_Solenoid_trig__R"(w635) -> ()
              n409 = Select(t=u8 1, s=w638, f=w646) -> (s? t:f=w642:u8)
              n410 = Select(t=u8 1, s=w669, f=w662) -> (s? t:f=w658:u8)
              n411 = Select(t=u8 2, s=w651, f=w646) -> (s? t:f=w643:u8)
              n412 = Select(t=u8 4, s=w648, f=w646) -> (s? t:f=w644:u8)
              n413 = Select(t=u8 2, s=w667, f=w662) -> (s? t:f=w659:u8)
              n414 = Select(t=u8 4, s=w664, f=w662) -> (s? t:f=w660:u8)
              n415 = Compound Arithmetic op=ADD(w642, w643, w644) -> (w641:u8)
              n416 = Compound Arithmetic op=ADD(w658, w659, w660) -> (w657:u8)
              n417 = case shown="7" w657 {
                tunnel: w639 -> [w699 w704 w706 w711 w716 w718 w721 w726]
                tunnel: [w699 w705 w706 w712 w717 w718 w722 w727] -> w654
                tunnel: w656 -> [_ w702 _ w709 w714 _ w720 w725]
                tunnel: w655 -> [_ w703 _ w710 w715 _ _ _]
                frame 0, Default {
                }
                frame 1 {
                  n418 = Replace Array Subset(array=w704, new element #1=u16 100 ("new element/subarray"), index #1=w703, new element #2=u16 1 ("new element/subarray"), index #2=w702) -> (w705:u16[])
                }
                frame 2 {
                }
                frame 3 {
                  n419 = Replace Array Subset(array=w711, new element #1=u16 100 ("new element/subarray"), index #1=w710, new element #2=u16 1 ("new element/subarray"), index #2=w709) -> (w712:u16[])
                }
                frame 4 {
                  w713 = u16 0 ("new element/subarray")
                  n420 = Replace Array Subset(array=w716, new element #1=w713, index #1=w715, new element #2=w713, index #2=w714) -> (w717:u16[])
                }
                frame 5 {
                }
                frame 6 {
                  n421 = Replace Array Subset(array=w721, new element=u16 0 ("new element/subarray"), index=w720) -> (w722:u16[])
                }
                frame 7 {
                  n422 = local write "RewCalib_Trig_L"(FALSE ("RewCalib_Trig_L")) -> ()
                  n423 = Replace Array Subset(array=w726, new element=u16 0 ("new element/subarray"), index=w725) -> (w727:u16[])
                }
              }
              n424 = case shown="7" w641 {
                tunnel: w654 -> [w670 w675 w677 w682 w687 w689 w692 w697]
                tunnel: [w670 w676 w677 w683 w688 w689 w693 w698] -> w653
                tunnel: w637 -> [_ w673 _ w680 w685 _ w691 w696]
                tunnel: w640 -> [_ w674 _ w681 w686 _ _ _]
                frame 0, Default {
                }
                frame 1 {
                  n425 = Replace Array Subset(array=w675, new element #1=u16 100 ("new element/subarray"), index #1=w674, new element #2=u16 1 ("new element/subarray"), index #2=w673) -> (w676:u16[])
                }
                frame 2 {
                }
                frame 3 {
                  n426 = Replace Array Subset(array=w682, new element #1=u16 100 ("new element/subarray"), index #1=w681, new element #2=u16 1 ("new element/subarray"), index #2=w680) -> (w683:u16[])
                }
                frame 4 {
                  w684 = u16 0 ("new element/subarray")
                  n427 = Replace Array Subset(array=w687, new element #1=w684, index #1=w686, new element #2=w684, index #2=w685) -> (w688:u16[])
                }
                frame 5 {
                }
                frame 6 {
                  n428 = Replace Array Subset(array=w692, new element=u16 0 ("new element/subarray"), index=w691) -> (w693:u16[])
                }
                frame 7 {
                  n429 = local write "RewCalib_Trig_R"(FALSE ("RewCalib_Trig_L")) -> ()
                  n430 = Replace Array Subset(array=w697, new element=u16 0 ("new element/subarray"), index=w696) -> (w698:u16[])
                }
              }
            }
            frame "DispenseWater_pre" {
              w734 = u16 0 ("t")
              w777 = u16 0 ("new element/subarray")
              # "just trust me on this one"
              # "RewCalib\nOnOff"
              # "RewCalib\nOnOff"
              # "nCycle"
              # "Solenoid__R"
              # "Tdelay"
              # "delay"
              # "nCycle"
              # "Solenoid__L"
              # "Tdelay"
              # "delay"
              # "Solenoid__R"
              # "count"
              # "Solenoid_Tcycle_R"
              # "Solenoid_Tcycle_L"
              # "Solenoid__L"
              # "count"
              n431 = call "myRIO_BRig_RT_dataMTrig_Solenoid_RewCalib_OnOff__L.vi"() -> ("output_Solenoid_RewCalib_OnOff__L"=w741:i32)  [unwired: 11 in]
              n432 = call "myRIO_BRig_RT_dataMTrig_Solenoid_N__L.vi"() -> ("output_Solenoid_N__L"=w732:i32)  [unwired: 11 in]
              n433 = call "myRIO_BRig_RT_dataMTrig_Solenoid_delay__L.vi"() -> ("output_Solenoid_delay__L"=w775:i32)  [unwired: 11 in]
              n434 = call "myRIO_BRig_RT_dataMTrig_Solenoid_Tdelay__L.vi"() -> ("output_Solenoid_Tdelay__L"=w774:i32)  [unwired: 11 in]
              n435 = call "myRIO_BRig_RT_dataMTrig_Solenoid_N__R.vi"() -> ("output_Solenoid_N__R"=w730:i32)  [unwired: 11 in]
              n436 = call "myRIO_BRig_RT_dataMTrig_Solenoid_delay__R.vi"() -> ("output_Solenoid_delay__R"=w764:i32)  [unwired: 11 in]
              n437 = call "myRIO_BRig_RT_dataMTrig_Solenoid_Tdelay__R.vi"() -> ("output_Solenoid_Tdelay__R"=w763:i32)  [unwired: 11 in]
              n438 = call "myRIO_BRig_RT_dataMTrig_Solenoid_RewCalib_OnOff__R.vi"() -> ("output_Solenoid_RewCalib_OnOff__R"=w737:i32)  [unwired: 11 in]
              n439 = Index Array(array=w776, index #1=w732, index #2=w775, index #3=w774, index #4=w730, index #5=w764, index #6=w763, index #7=w741, index #8=w737) -> (element #1=w733:u16, element #2=w773:u16, element #3=w768:u16, element #4=w736:u16, element #5=w758:u16, element #6=w757:u16, element #7=w742:u16, element #8=w739:u16)
              n440 = Equal To 0?(x=w773) -> (x = 0?=w772:bool)
              n441 = Equal To 0?(x=w758) -> (x = 0?=w762:bool)
              n442 = local read "RewCalib_Trig_L"() -> (w753:bool)
              n443 = local read "RewCalib_Trig_R"() -> (w748:bool)
              n444 = Not Equal To 0?(x=w733) -> (x != 0?=w771:bool)
              n445 = Not Equal To 0?(x=w736) -> (x != 0?=w761:bool)
              n446 = local read "MTrig_Solenoid_Tcycle__L"() -> (w770:u16)
              n447 = local read "MTrig_Solenoid_Tcycle__R"() -> (w756:u16)
              n448 = Not Equal To 0?(x=w742) -> (x != 0?=w752:bool)
              n449 = Not Equal To 0?(x=w739) -> (x != 0?=w750:bool)
              n450 = Not(x=w753) -> (.not. x?=w751:bool)
              n451 = Not(x=w748) -> (.not. x?=w749:bool)
              n452 = And(x=w752, y=w751) -> (x .and. y?=w747:bool)
              n453 = And(x=w750, y=w749) -> (x .and. y?=w746:bool)
              n454 = call "myRIO_BRig_RT_dataMTrig_Solenoid_c__L.vi"() -> ("output_Solenoid_c__L"=w779:i32)  [unwired: 11 in]
              n455 = call "myRIO_BRig_RT_dataMTrig_Solenoid_c__R.vi"() -> ("output_Solenoid_c__R"=w778:i32)  [unwired: 11 in]
              n456 = Select(t=w770, s=w771, f=u16 0) -> (s? t:f=w767:u16)
              n457 = Or(x=w747, y=w746) -> (x .or. y?=w735:bool)
              n458 = Select(t=w756, s=w761, f=u16 0) -> (s? t:f=w759:u16)
              n459 = Select(t=w767, s=w772, f=w768) -> (s? t:f=w765:u16)
              n460 = Select(t=w759, s=w762, f=w757) -> (s? t:f=w754:u16)
              n461 = call "myRIO_BRig_RT_dataMTrig_Solenoid_Tcycle__L.vi"() -> ("output_Solenoid_Tcycle__L"=w766:i32)  [unwired: 11 in]
              n462 = call "myRIO_BRig_RT_dataMTrig_Solenoid_Tcycle__R.vi"() -> ("output_Solenoid_Tcycle__R"=w755:i32)  [unwired: 11 in]
              n463 = Select(t=w734, s=w735, f=w733) -> (s? t:f=w731:u16)
              n464 = Select(t=w734, s=w735, f=w736) -> (s? t:f=w729:u16)
              n465 = Select(t=myRIO_BRig_RT__Case_NonExp_stateList."Idle" ("Enum"), s=w735, f=myRIO_BRig_RT__Case_NonExp_stateList."DispenseWater" ("Enum")) -> (s? t:f=w743:T1)
              n466 = Select(t=w734, s=w735, f=w742) -> (s? t:f=w740:u16)
              n467 = Select(t=w734, s=w735, f=w739) -> (s? t:f=w738:u16)
              n468 = Replace Array Subset(array=w776, new element #1=w777, index #1=w779, new element #2=w777, index #2=w778, new element #3=w765, index #3=w766, new element #4=w754, index #4=w755, new element #5=w740, index #5=w741, new element #6=w738, index #6=w737, new element #7=w731, index #7=w732, new element #8=w729, index #8=w730) -> (w780:u16[])
            }
            frame "DispenseWater" {
              # "D"
              # "C"
              # "B"
              # "A"
              # "(A) Add COUNT and INCREMENT\n(B) Is (A) smaller than Tcycle?\n(C) Are we dispensing water or in the delay phase?\n(D) If (A) is smaller than Tcycle   AND   if we are dispensing water\n      then send TRUE to solenoid"
              # "delay"
              # "Tcycle"
              # "Solenoid__R"
              # "count"
              # "delay"
              # "Tcycle"
              # "Solenoid__L"
              # "count"
              n469 = To Unsigned Word Integer(number=w808) -> (unsigned 16bit integer=w790:u16)
              n470 = call "myRIO_BRig_RT_dataMTrig_Solenoid_delay__R.vi"() -> ("output_Solenoid_delay__R"=w794:i32)  [unwired: 11 in]
              n471 = call "myRIO_BRig_RT_dataMTrig_Solenoid_c__R.vi"() -> ("output_Solenoid_c__R"=w793:i32)  [unwired: 11 in]
              n472 = call "myRIO_BRig_RT_dataMTrig_Solenoid_Tcycle__R.vi"() -> ("output_Solenoid_Tcycle__R"=w795:i32)  [unwired: 11 in]
              n473 = call "myRIO_BRig_RT_dataMTrig_Solenoid_delay__L.vi"() -> ("output_Solenoid_delay__L"=w810:i32)  [unwired: 11 in]
              n474 = call "myRIO_BRig_RT_dataMTrig_Solenoid_c__L.vi"() -> ("output_Solenoid_c__L"=w802:i32)  [unwired: 11 in]
              n475 = call "myRIO_BRig_RT_dataMTrig_Solenoid_Tcycle__L.vi"() -> ("output_Solenoid_Tcycle__L"=w811:i32)  [unwired: 11 in]
              n476 = Index Array(array=w804, index #1=w802, index #2=w811, index #3=w810, index #4=w793, index #5=w795, index #6=w794) -> (element #1=w809:u16, element #2=w799:u16, element #3=w807:u16, element #4=w789:u16, element #5=w786:u16, element #6=w785:u16)
              n477 = Add(x=w809, y=w790) -> (x+y=w800:u16)
              n478 = Add(x=w789, y=w790) -> (x+y=w791:u16)
              n479 = Less?(x=w800, y=w799) -> (x < y?=w783:bool)
              n480 = Equal To 0?(x=w807) -> (x = 0?=w806:bool)
              n481 = Less?(x=w791, y=w786) -> (x < y?=w784:bool)
              n482 = Equal To 0?(x=w785) -> (x = 0?=w792:bool)
              n483 = And(x=w783, y=w806) -> (x .and. y?=w805:bool)
              n484 = Or(x=w783, y=w784) -> (x .or. y?=w782:bool)
              n485 = And(x=w784, y=w792) -> (x .and. y?=w787:bool)
              n486 = Select(t=w800, s=w783, f=w799) -> (s? t:f=w801:u16)
              n487 = Select(t=w791, s=w784, f=w786) -> (s? t:f=w788:u16)
              n488 = Replace Array Subset(array=w804, new element #1=w801, index #1=w802, new element #2=w788, index #2=w793) -> (w803:u16[])
              n489 = Select(t=w798, s=w782, f=myRIO_BRig_RT__Case_NonExp_stateList."DispenseWater_post" ("Enum")) -> (s? t:f=w796:T1)
            }
            frame "DispenseWater_post" {
              # "nCycle"
              # "delay"
              # "Solenoid__R"
              # "nCycle"
              # "delay"
              # "Solenoid__L"
              n490 = call "myRIO_BRig_RT_dataMTrig_Solenoid_N__L.vi"() -> ("output_Solenoid_N__L"=w829:i32)  [unwired: 11 in]
              n491 = call "myRIO_BRig_RT_dataMTrig_Solenoid_delay__L.vi"() -> ("output_Solenoid_delay__L"=w828:i32)  [unwired: 11 in]
              n492 = call "myRIO_BRig_RT_dataMTrig_Solenoid_N__R.vi"() -> ("output_Solenoid_N__R"=w825:i32)  [unwired: 11 in]
              n493 = call "myRIO_BRig_RT_dataMTrig_Solenoid_delay__R.vi"() -> ("output_Solenoid_delay__R"=w824:i32)  [unwired: 11 in]
              n494 = Index Array(array=w831, index #1=w829, index #2=w828, index #3=w825, index #4=w824) -> (element #1=w833:u16, element #2=w832:u16, element #3=w816:u16, element #4=w818:u16)
              n495 = Not Equal To 0?(x=w833) -> (x != 0?=w834:bool)
              n496 = Not Equal To 0?(x=w816) -> (x != 0?=w817:bool)
              n497 = case shown="True" w817 {
                selector: w817 -> [_ w838]
                tunnel: w816 -> [w836 w844]
                tunnel: w818 -> [_ w845]
                tunnel: [w836 w842] -> w815
                tunnel: [u16 0 w841] -> w814
                tunnel: [_ w838] -> w813
                frame False {
                }
                frame True {
                  n498 = Equal To 0?(x=w845) -> (x = 0?=w837:bool)
                  n499 = Decrement(x=w844) -> (x-1=w843:u16)
                  n500 = Select(t=w843, s=w837, f=w844) -> (s? t:f=w842:u16)
                  n501 = Select(t=u16 1, s=w837, f=u16 0) -> (s? t:f=w841:u16)
                }
              }
              n502 = case shown="True" w834 {
                selector: w834 -> [_ w849]
                tunnel: w833 -> [w847 w855]
                tunnel: w832 -> [_ w856]
                tunnel: [w847 w853] -> w827
                tunnel: [u16 0 w852] -> w826
                tunnel: [_ w849] -> w823
                frame False {
                }
                frame True {
                  n503 = Equal To 0?(x=w856) -> (x = 0?=w848:bool)
                  n504 = Decrement(x=w855) -> (x-1=w854:u16)
                  n505 = Select(t=w854, s=w848, f=w855) -> (s? t:f=w853:u16)
                  n506 = Select(t=u16 1, s=w848, f=u16 0) -> (s? t:f=w852:u16)
                }
              }
              n507 = Or(x=w823, y=w813) -> (x .or. y?=w822:bool)
              n508 = Replace Array Subset(array=w831, new element #1=w827, index #1=w829, new element #2=w826, index #2=w828, new element #3=w815, index #3=w825, new element #4=w814, index #4=w824) -> (w830:u16[])
              n509 = Select(t=myRIO_BRig_RT__Case_NonExp_stateList."DispenseWater_pre" ("Enum"), s=w822, f=myRIO_BRig_RT__Case_NonExp_stateList."Idle" ("Enum")) -> (s? t:f=w819:T1)
            }
            frame "TestConnection" {
              n510 = local read "Host Password"() -> (w863:string)
              n511 = local read "Host UserName"() -> (w864:string)
              n512 = call "myRIO_BRig_RT_comm_webdav_testConnect.vi"("input_password"=w863, "input_username"=w864) -> ("output_Iconnected"=w861:bool)  [unwired: 9 in]
              n513 = Select(t="Connection accepted!" ("message"), s=w861, f="Error!") -> (s? t:f=w859:string)
              n514 = One Button Dialog(message=w859) -> ()  [unwired: 1 in, 1 out]
            }
            frame "SendData" {
              n515 = local read "Data Set Prefix"() -> (w866:string)
              n516 = local read "Host Password"() -> (w867:string)
              n517 = local read "Host UserName"() -> (w868:string)
              n518 = call "myRIO_BRig_RT_comm_webdav_sendData_all.vi"("Host Filename Prefix"=w866, "Host Password"=w867, "Host UserName"=w868) -> ()  [unwired: 9 in]
            }
            frame "Get_FPGA_count_per_ms" {
              n519 = case shown="False" w882 {
                selector: w882 -> [w885 _]
                tunnel: w880 -> [_ w898]
                tunnel: [w889 w898] -> w879
                tunnel: w878 -> [w888 w896]
                tunnel: w877 -> [w887 w895]
                tunnel: [w886 w893] -> w876
                tunnel: [w885 w892] -> w875
                frame False {
                  n520 = Get Date/Time In Seconds() -> (seconds since 1Jan1904=w890:timestamp)
                  n521 = xnode "Read/Write Control"("FPGA VI Reference In"=w888, "error in"=w887, "timeTrial"=TRUE) -> ("error out"=w886:errorcluster)  [unwired: 1 out]
                  n522 = To Double Precision Float(number=w890) -> (double precision float=w889:dbl)
                  n523 = local write "get_countPerMS"(w885) -> ()
                }
                frame True {
                  w894 = 1.0
                  n524 = Get Date/Time In Seconds() -> (seconds since 1Jan1904=w899:timestamp)
                  n525 = To Double Precision Float(number=w899) -> (double precision float=w900:dbl)
                  n526 = Subtract(x=w900, y=w898) -> (x-y=w897:dbl)
                  n527 = Less Or Equal?(x=w894, y=w897) -> (x <= y?=w892:bool)
                  n528 = case shown="True" w892 {
                    tunnel: w896 -> [_ w913]
                    tunnel: w895 -> [w901 w912]
                    tunnel: w894 -> [_ w903]
                    tunnel: [w901 w902] -> w893
                    frame False {
                    }
                    frame True {
                      n529 = xnode "Read/Write Control"("FPGA VI Reference In"=w913, "error in"=w912) -> ("FPGA VI Reference Out"=w910:refnum<k20>, "error out"=w909:errorcluster, "count_timeTrial"=w904:u32)
                      n530 = Multiply(x=w903, y=1000.0) -> (x*y=w907:dbl)
                      n531 = To Double Precision Float(number=w904) -> (double precision float=w906:dbl)
                      n532 = Divide(x=w906, y=w907) -> (x/y=w908:dbl)
                      n533 = local write "FPGA_count2ms"(w908) -> ()
                      n534 = xnode "Read/Write Control"("FPGA VI Reference In"=w910, "error in"=w909, "timeTrial"=FALSE) -> ("error out"=w902:errorcluster)  [unwired: 1 out]
                    }
                  }
                }
              }
              "error out 5" <- w876
              n535 = Select(t=myRIO_BRig_RT__Case_NonExp_stateList."Idle" ("Enum"), s=w875, f=w873) -> (s? t:f=w872:T1)
            }
            frame "End" {
            }
          }
          n536 = local read "MTrig_Audio_trig__R"() -> (w119:bool)
          n537 = local read "MTrig_Audio_trig__L"() -> (w118:bool)
          n538 = local read "START"() -> (w114:bool)
          n539 = local read "STOP_abort"() -> (w113:bool)
          n540 = local read "MTrig_Laser_trig"() -> (w120:bool)
          n541 = call "myRIO_BRig_RT_dataMTrig_main__v2.vi"("input_dataMTrig"=w122, "input_Audio_trig_L"=w118, "input_Audio_trig_R"=w119, "input_Laser_trig"=w120) -> ("output_dataMTrig"=w121:u16[], "output_Audio_L"=w98:bool, "output_Audio_R"=w109:bool, "output_Laser"=w101:bool)  [unwired: 12 in]
          n542 = Or(x=w114, y=w113) -> (x .or. y?=w112:bool)
          n543 = Select(t=myRIO_BRig_RT__Case_NonExp_stateList."End" ("Enum"), s=w112, f=w111) -> (s? t:f=w110:T1)
          n544 = Or(x=w119, y=w120) -> (x .or. y?=w117:bool)
          n545 = Or(x=w117, y=w118) -> (x .or. y?=w116:bool)
          n546 = case shown="True" w116 {
            frame False {
            }
            frame True {
              w135 = FALSE
              n547 = local write "MTrig_Audio_trig__R"(w135) -> ()
              n548 = local write "MTrig_Audio_trig__L"(w135) -> ()
              n549 = local write "MTrig_Laser_trig"(w135) -> ()
            }
          }
          n550 = xnode "Read/Write Control"("FPGA VI Reference In"=w87, "error in"=w86, "A1_SR"=w123, "A3_SL"=w124, "audioTrigger_L"=w98, "audioTrigger_R"=w109, "laserResponse_reward_LED"="laserResponse_reward_LED", "laserResponse_wrong_LED"="laserResponse_wrong_LED", "laserResponse_reward"="laserResponse_reward", "laserResponse_wrong"="laserResponse_wrong", "SelectionState"="SelectionState", "ignoreWrong"="ignoreWrong", "Left(F)_or_Right(T)"="Left(F)_or_Right(T)", "laser1_On"=w101) -> ("FPGA VI Reference Out"=w129:refnum<k20>, "error out"=w128:errorcluster, "SelectReward"=→"SelectReward":bool, "SelectWrong"=→"SelectWrong":bool)
          n551 = node-c288() -> ()  [unwired: 1 in, 1 out]
          "cState_NonExp" <- w127
        }
        n552 = node-c288(w70) -> ()  [unwired: 1 out]
        n553 = flat-sequence {
          tunnel: w63 -> [w81]
          tunnel: [w81] -> w62
          tunnel: w61 -> [w80]
          tunnel: [w80] -> w60
          frame #0 {
            w79 = FALSE
            n554 = local write "STOP_endBlock"(w79) -> ()
            n555 = local write "STOP_endTrial"(w79) -> ()
          }
        }
      }
      frame True {
        w924 = u16 0
        w943 = u8 0
        w944 = FALSE ("SelectionState")
        w949 = u16 0 ("idxDataBlock")
        w951 = u16 100 ("new element/subarray")
        w952 = u16 100 ("new element/subarray")
        w972 = T7 refnum items=["Session NI_WebDAV"] ("output_hSession")
        w981 = FALSE
        w982 = u16 0
        w931 = FALSE
        # "dummyState counter"
        # "audio__L\naudio__R"
        # "Audio params"
        # "nRewards"
        # "idxDataBlock"
        # "Solenoid_Tdelay_R"
        # "Solenoid_Tdelay_L"
        # "RewCalib_N__R"
        # "RewCalib_N__L"
        # "Save dataLick to file\nSend file to Host\nSave dataMTrig\nSend file to Host\nDisconnect"
        # "dataTrial"
        # "dataTrial"
        # "Solenoid_Tcycle_R"
        # "Solenoid_Tcycle_L"
        # "Laser_Tcycle"
        # "Audio_Tcycle_R"
        # "Audio_Tcycle_L"
        # "dataLick"
        # "dataLC"
        # "dataLC"
        # "dataBlock"
        # "dataBlock"
        # "dataMTrig"
        # "dataMTrig"
        # "dataExp"
        # "dataCurrent"
        # "dataExp"
        # "dataCurrent"
        # "spout"
        # "state"
        n556 = call "myRIO_BRig_RT_dataMTrig_Solenoid_Tcycle__L.vi"() -> ("output_Solenoid_Tcycle__L"=w978:i32)  [unwired: 11 in]
        n557 = call "myRIO_BRig_RT_dataMTrig_Solenoid_Tcycle__R.vi"() -> ("output_Solenoid_Tcycle__R"=w977:i32)  [unwired: 11 in]
        n558 = call "myRIO_BRig_RT_dataMTrig_Audio_Tcycle__L.vi"() -> ("output_Audio_Tcycle__L"=w976:i32)  [unwired: 11 in]
        n559 = call "myRIO_BRig_RT_dataMTrig_Audio_Tcycle__R.vi"() -> ("output_Audio_Tcycle__R"=w975:i32)  [unwired: 11 in]
        n560 = call "myRIO_BRig_RT_dataMTrig_Laser_Tcycle.vi"() -> ("output_Laser_Tcycle"=w974:i32)  [unwired: 11 in]
        n561 = local read "MTrig_Solenoid_Tcycle__L"() -> (w957:u16)
        n562 = local read "MTrig_Solenoid_Tcycle__R"() -> (w956:u16)
        n563 = local read "Tcycle_Reward_L"() -> (w953:u16)
        n564 = local read "Tcycle_Reward_R"() -> (w954:u16)
        n565 = local read "MTrig_Laser_Tcycle"() -> (w955:u16)
        n566 = call "myRIO_BRig_RT_dataMTrig_Solenoid_RewCalib_nCycle__L.vi"() -> ("output_Solenoid_RewCalib_nCycle__L"=w960:i32)  [unwired: 11 in]
        n567 = call "myRIO_BRig_RT_dataMTrig_Solenoid_Tdelay__L.vi"() -> ("output_Solenoid_Tdelay__L"=w962:i32)  [unwired: 11 in]
        n568 = call "myRIO_BRig_RT_dataMTrig_Solenoid_RewCalib_nCycle__R.vi"() -> ("output_Solenoid_RewCalib_nCycle__R"=w961:i32)  [unwired: 11 in]
        n569 = call "myRIO_BRig_RT_dataMTrig_Solenoid_Tdelay__R.vi"() -> ("output_Solenoid_Tdelay__R"=w963:i32)  [unwired: 11 in]
        n570 = case shown="False" w935 {
          selector: w935 -> [_ w1004]
          tunnel: w934 -> [w1001 w1006]
          tunnel: [w1002 w1006] -> w929
          tunnel: w933 -> [_ w1005]
          tunnel: [w1003 w1005] -> w930
          tunnel: [w1000 w1004] -> w928
          frame False {
            n571 = call "myRIO__TCP_connect_forWriting.vi"("input_error"=w1001) -> ("output_error"=w1002:errorcluster, "output_connected"=w1000:bool, "output_hTCP"=w1003:refnum<k5>)  [unwired: 8 in]
          }
          frame True {
          }
        }
        n572 = call "myRIO_BRig_RT_dataLick_init.vi"() -> ("output_dataLick"=w984:u16[][])  [unwired: 11 in]
        n573 = call "myRIO_BRig_RT_dataCurrent_init.vi"() -> ("output_dataCurrent"=w991:u16[])  [unwired: 11 in]
        n574 = call "myRIO_BRig_RT_dataExp_init.vi"() -> ("output_dataExp"=w990:u16[])  [unwired: 11 in]
        n575 = call "myRIO_BRig_RT_dataMTrig_init.vi"() -> ("output_dataMTrig"=w980:u16[])  [unwired: 5 in]
        n576 = call "myRIO_BRig_RT_dataLC_init.vi"() -> ("output_dataLC"=w988:u16[])  [unwired: 11 in]
        n577 = call "myRIO_BRig_RT_dataBlock_init.vi"() -> ("output_dataBlock"=w989:u16[][])  [unwired: 11 in]
        n578 = call "myRIO_BRig_RT_dataTrial_init.vi"() -> ("output_dataTrial"=w973:u16[][])  [unwired: 11 in]
        n579 = xnode "Read/Write Control"("FPGA VI Reference In"=w945, "error in"=w946, "SelectionState"=w944, "laserResponse_reward"=w944, "laserResponse_wrong"=w944, "laserResponse_reward_LED"=w944, "laserResponse_wrong_LED"=w944, "Left(F)_or_Right(T)"=w944, "ignoreWrong"=w944, "SelectionState"=w944) -> ("FPGA VI Reference Out"=w947:refnum<k20>, "error out"=w948:errorcluster)
        n580 = local write "I_connect_TCP"(w928) -> ()
        n581 = Replace Array Subset(array=w980, new element #1=w952, index #1=w960, new element #2=w952, index #2=w961, new element #3=w951, index #3=w962, new element #4=w951, index #4=w963, new element #5=w957, index #5=w978, new element #6=w956, index #6=w977, new element #7=w953, index #7=w976, new element #8=w954, index #8=w975, new element #9=w955, index #9=w974) -> (w979:u16[])
        n582 = call "myRIO_BRig_RT_dataAnalog_init.vi"() -> ("output_dataAnalog"=w940:u16[][])  [unwired: 11 in]
        n583 = call "myRIO_BRig_RT_TCP__start_exp.vi"("input_hTCP"=w930, "input_I_connected_TCP"=w928, "input_error"=w929) -> ("output_hTCP"=w927:refnum<k5>, "output_error"=w926:errorcluster)  [unwired: 11 in]
        n584 = Get Date/Time In Seconds() -> (seconds since 1Jan1904=w959:timestamp)
        n585 = call "myRIO_BRig_RT_arrTrig_init.vi"() -> ("output_arrTrig"=w923:bool[])  [unwired: 11 in]
        n586 = To Double Precision Float(number=w959) -> (double precision float=w958:dbl)
        n587 = node-c288() -> (w999:T3)  [unwired: 4 in]
        n588 = timed-loop {
          timing: w999 -> [_]
          timing-out: [_] -> w998
          shift-right: [w1129] -> _
          shift-left: myRIO_BRig_RT__Case_Exp_stateList."Start1" ("Enum") -> [w1064]
          shift-right: [w1061] -> _
          shift-left: enum16{"Left", "Right"}."Left" -> [w1178]
          tunnel: w947 -> [w1176]
          tunnel: w948 -> [w1175]
          shift-right: [w1170] -> _
          shift-left: w996 -> [w1174]
          shift-right: [w1169] -> _
          shift-left: w995 -> [w1173]
          tunnel: [w1152] -> w993
          tunnel: [w1153] -> w994
          shift-right: [w1154] -> w964
          shift-left: w991 -> [w1121]
          shift-right: [w1168] -> _
          shift-left: w990 -> [w1118]
          shift-right: [w1141] -> w968
          shift-left: w979 -> [w1142]
          shift-right: [w1166] -> _
          shift-left: w989 -> [w1167]
          shift-right: [w1164] -> _
          shift-left: w988 -> [w1165]
          shift-right: [w1156] -> w970
          shift-left: w984 -> [w1157]
          shift-right: [w1143] -> _
          shift-left: w982 -> [w1151]
          shift-right: [w1115] -> _
          shift-left: w943 -> [w1150]
          shift-right: [w1144] -> _
          shift-left: w982 -> [w1149]
          shift-right: [w1145] -> _
          shift-left: w943 -> [w1148]
          shift-right: [w1116] -> _
          shift-left: w981 -> [w1146]
          shift-right: [w1117] -> _
          shift-left: w981 -> [w1147]
          shift-right: [w1127] -> _
          shift-left: w973 -> [w1128]
          shift-right: [w1126] -> w966
          shift-left: w972 -> [w1124]
          shift-right: [w1125] -> w967
          shift-left: FALSE ("output_Iconnected") -> [w1123]
          tunnel: "Data Set Prefix" -> [w1122]
          tunnel: [w1122] -> w965
          shift-right: [w1100] -> _
          shift-left: w931 -> [w1120]
          tunnel: w958 -> [w1119]
          shift-right: [w1113] -> _
          shift-left: 0 ("idxDataBlock") -> [w1114]
          shift-right: [w1110] -> _
          shift-left: w949 -> [w1112]
          shift-right: [w1109] -> _
          shift-left: w949 -> [w1111]
          shift-right: [w1099] -> _
          shift-left: w931 -> [w1105]
          shift-right: [w1102] -> _
          shift-left: w931 -> [w1104]
          shift-right: [w1101] -> _
          shift-left: w931 -> [w1103]
          shift-right: [w1087] -> w938
          shift-left: 0 -> [w1071]
          shift-right: [w1062] -> _
          shift-left: w924 -> [w1082]
          shift-right: [w1063] -> _
          shift-left: w924 -> [w1078]
          shift-right: [w1091] -> _
          shift-left: FALSE -> [w1091]
          shift-right: [w1077] -> _
          shift-left: w924 -> [w1085]
          shift-right: [w1088] -> w939
          shift-left: w940 -> [w1089]
          tunnel: w927 -> [w1076]
          tunnel: [w1075] -> w937
          tunnel: w928 -> [w1072]
          tunnel: [w1072] -> w936
          tunnel: w926 -> [w1074]
          tunnel: [w1073] -> w932
          shift-right: [w1067] -> _
          shift-left: w931 -> [w1068]
          shift-right: [w1065] -> _
          shift-left: w931 -> [w1066]
          shift-right: [w1059] -> _
          shift-left: u16 0 -> [w1060]
          shift-right: [w1057] -> _
          shift-left: w924 -> [w1058]
          shift-right: [w1054] -> _
          shift-left: w923 -> [w1055]
          stop <- w1163 stop-if-true
          # "Sel"
          # "Sel"
          # "Cue1"
          # "Cue1"
          # "ENL1"
          # "ENL1"
          # "iState"
          # "dataAnalog"
          # "index"
          # "iEvent"
          # "iBlock"
          # "iTrial"
          # "Laser"
          # "Audio R"
          # "Audio L"
          # "Solenoid R"
          # "Solenoid L"
          # "manual triggering"
          # "dataTrial"
          # "dataBlock"
          # "nRewards"
          # "dataExp"
          # "dataCurrent"
          # "audio__L\naudio__R"
          # "time stamp"
          # "Audio params"
          # "nRewards"
          # "idxDataBlock"
          # "idxDataBlock"
          # "activate"
          # "audio__L\naudio__R"
          # "amp__R\nfreq__R"
          # "amp__L\nfreq__L"
          # "dataLC"
          # "solenoid__R"
          # "solenoid__L"
          # "Did a lick occur?"
          # "Update lick counter"
          # "spout"
          # "spout"
          # "state"
          # "state"
          n589 = node-c288() -> ()  [unwired: 1 in, 1 out]
          n590 = local read "MTrig_Solenoid_trig__L"() -> (w1139:bool)
          n591 = local read "MTrig_Solenoid_trig__R"() -> (w1138:bool)
          n592 = local read "MTrig_Audio_trig__L"() -> (w1137:bool)
          n593 = local read "MTrig_Audio_trig__R"() -> (w1136:bool)
          n594 = xnode "Read/Write Control"("FPGA VI Reference In"=w1176, "error in"=w1175) -> ("FPGA VI Reference Out"=w1108:refnum<k20>, "error out"=w1107:errorcluster, "A2_LickL"=w1170:u32, "A4_LickR"=w1169:u32)
          "A2" <- w1170
          "A4" <- w1169
          n595 = local read "MTrig_Laser_trig"() -> (w1135:bool)
          n596 = Greater?(x=w1170, y=w1174) -> (0:w1172:bool)
          n597 = Greater?(x=w1169, y=w1173) -> (0:w1171:bool)
          n598 = Or(x=w1172, y=w1171) -> (x .or. y?=w1177:bool)
          n599 = call "myRIO_BRig_RT_dataMTrig_main.vi"("input_dataMTrig"=w1142, "input_Solenoid_trig_L"=w1139, "input_Solenoid_trig_R"=w1138, "input_Audio_trig_L"=w1137, "input_Audio_trig_R"=w1136, "input_Laser_trig"=w1135) -> ("output_Laser"=w1097:bool, "output_dataMTrig"=w1141:u16[], "output_Solenoid_L"=w1053:bool, "output_Solenoid_R"=w1131:bool, "output_Audio_L"=w1133:bool, "output_Audio_R"=w1134:bool)  [unwired: 8 in]
          n600 = Compound Arithmetic op=OR(w1139, w1138, w1137, w1136, w1135) -> (w1140:bool)
          n601 = case shown="True" w1140 {
            frame False {
            }
            frame True {
              w1179 = FALSE
              n602 = local write "MTrig_Solenoid_trig__L"(w1179) -> ()
              n603 = local write "MTrig_Solenoid_trig__R"(w1179) -> ()
              n604 = local write "MTrig_Audio_trig__L"(w1179) -> ()
              n605 = local write "MTrig_Audio_trig__R"(w1179) -> ()
              n606 = local write "MTrig_Laser_trig"(w1179) -> ()
            }
          }
          n607 = case shown="39" w1064 {
            selector: w1064 -> [_ _ _ _ _ _ _ _ _ _ _ _ _ _ _ _ _ _ _ _ _ _ _ _ w2147 _ w2214 _ _ _ _ _ w2359 _ w2436 _ _ _ _ _ w2591 _ w2665 _ w2729 _ w2773 _ _ w2843 _ _ _ _ _ w3014 _ _ _ _ _ _ _ _ _ _ _ _ w3295 w3328]
            tunnel: [myRIO_BRig_RT__Case_Exp_stateList."Start2" ("Enum") myRIO_BRig_RT__Case_Exp_stateList."Start3" ("Enum") myRIO_BRig_RT__Case_Exp_stateList."saveSettings1" ("Enum") myRIO_BRig_RT__Case_Exp_stateList."saveSettings2" ("Enum") myRIO_BRig_RT__Case_Exp_stateList."saveSettings3" ("Enum") myRIO_BRig_RT__Case_Exp_stateList."saveSettings4_LC_l1_ENL" ("Enum") myRIO_BRig_RT__Case_Exp_stateList."saveSettings4_LC_l2_ENL" ("Enum") myRIO_BRig_RT__Case_Exp_stateList."saveSettings5_LC_l1_Cue" ("Enum") myRIO_BRig_RT__Case_Exp_stateList."saveSettings5_LC_l2_Cue" ("Enum") myRIO_BRig_RT__Case_Exp_stateList."saveSettings6_LC_l1_Other" ("Enum") myRIO_BRig_RT__Case_Exp_stateList."SaveSettings6_LC_l2_Other" ("Enum") myRIO_BRig_RT__Case_Exp_stateList."setSettings_Audio" ("Enum") myRIO_BRig_RT__Case_Exp_stateList."setSettings_Laser" ("Enum") myRIO_BRig_RT__Case_Exp_stateList."commConnect" ("Enum") w1871 myRIO_BRig_RT__Case_Exp_stateList."initTrial" ("Enum") w1916 myRIO_BRig_RT__Case_Exp_stateList."initTrial3" ("Enum") myRIO_BRig_RT__Case_Exp_stateList."initTrial_LC_ENL1" ("Enum") myRIO_BRig_RT__Case_Exp_stateList."ENL1_pre" ("Enum") myRIO_BRig_RT__Case_Exp_stateList."initTrial_LC_Cue1" ("Enum") myRIO_BRig_RT__Case_Exp_stateList."initTrial_LC_Sel" ("Enum") myRIO_BRig_RT__Case_Exp_stateList."initTrial4" ("Enum") w2106 w2144 myRIO_BRig_RT__Case_Exp_stateList."ENL1Penalty" ("Enum") w2215 myRIO_BRig_RT__Case_Exp_stateList."endExp" ("Enum") myRIO_BRig_RT__Case_Exp_stateList."endExp" ("Enum") myRIO_BRig_RT__Case_Exp_stateList."endExp" ("Enum") myRIO_BRig_RT__Case_Exp_stateList."endExp" ("Enum") w2311 w2358 myRIO_BRig_RT__Case_Exp_stateList."Cue1Penalty" ("Enum") w2434 myRIO_BRig_RT__Case_Exp_stateList."endExp" ("Enum") myRIO_BRig_RT__Case_Exp_stateList."endExp" ("Enum") myRIO_BRig_RT__Case_Exp_stateList."endExp" ("Enum") myRIO_BRig_RT__Case_Exp_stateList."endExp" ("Enum") w2531 w2597 myRIO_BRig_RT__Case_Exp_stateList."SelectReward" ("Enum") w2666 myRIO_BRig_RT__Case_Exp_stateList."SelectRewardPost" ("Enum") w2730 myRIO_BRig_RT__Case_Exp_stateList."SelectWrong" ("Enum") w2769 myRIO_BRig_RT__Case_Exp_stateList."endTrial1" ("Enum") myRIO_BRig_RT__Case_Exp_stateList."SelectTimeout" ("Enum") w2845 myRIO_BRig_RT__Case_Exp_stateList."endTrial1" ("Enum") myRIO_BRig_RT__Case_Exp_stateList."endTrial2" ("Enum") myRIO_BRig_RT__Case_Exp_stateList."endTrial3" ("Enum") w2931 w2997 w3014 myRIO_BRig_RT__Case_Exp_stateList."initBlock" ("Enum") w3041 myRIO_BRig_RT__Case_Exp_stateList."commUpload_dataExp" ("Enum") myRIO_BRig_RT__Case_Exp_stateList."endBlock" ("Enum") myRIO_BRig_RT__Case_Exp_stateList."commUpload_dataLC" ("Enum") myRIO_BRig_RT__Case_Exp_stateList."commUpload_dataTrial" ("Enum") myRIO_BRig_RT__Case_Exp_stateList."commUpload_dataCurrent" ("Enum") myRIO_BRig_RT__Case_Exp_stateList."saveData_dataCurrent" ("Enum") myRIO_BRig_RT__Case_Exp_stateList."saveData_dataExp" ("Enum") myRIO_BRig_RT__Case_Exp_stateList."saveData_dataLC" ("Enum") myRIO_BRig_RT__Case_Exp_stateList."saveData_dataTrial" ("Enum") myRIO_BRig_RT__Case_Exp_stateList."commUpload_pre" ("Enum") w3294 w3327] -> w1129
            tunnel: [w1205 w1224 w1246 w1301 w1349 w1417 w1481 w1545 w1609 w1673 w1716 w1760 w1786 w1842 w1848 w1879 w1898 w1932 w1963 w1999 w2024 w2050 w2080 w2122 w2160 w2191 w2219 w2235 w2257 w2276 w2295 w2330 w2380 w2405 w2433 w2454 w2475 w2494 w2513 w2542 w2615 w2640 w2663 w2677 w2727 w2751 w2783 w2804 w2824 w2855 w2878 w2890 w2909 w2951 w2970 w3013 w3030 w3044 w3078 w3099 w3120 w3141 w3162 w3190 w3210 w3237 w3257 w3281 w3315 w3348] -> w1061
            tunnel: w1178 -> [w1205 w1224 w1246 w1301 w1349 w1417 w1481 w1545 w1609 w1673 w1716 w1760 w1786 w1842 w1870 w1879 w1898 w1932 w1963 w1999 w2024 w2050 w2080 w2122 w2160 w2191 w2219 w2235 w2257 w2276 w2295 w2330 w2380 w2405 w2433 w2454 w2475 w2494 w2513 w2542 w2615 w2640 w2663 w2677 w2727 w2751 w2783 w2804 w2824 w2855 w2878 w2890 w2909 w2951 w2970 w3013 w3030 w3044 w3078 w3099 w3120 w3141 w3162 w3190 w3210 w3237 w3257 w3281 w3315 w3348]
            tunnel: w1177 -> [w1208 w1227 w1243 w1304 w1352 w1420 w1484 w1548 w1612 w1676 w1719 w1763 w1789 w1845 w1864 w1890 w1917 w1950 w1979 w2013 w2037 w2063 w2093 w2109 w2141 w2194 w2222 w2241 w2260 w2279 w2298 w2310 w2357 w2413 w2440 w2459 w2478 w2497 w2516 w2540 w2613 w2650 w2673 w2708 w2735 w2762 w2786 w2803 w2836 w2860 w2875 w2898 w2908 w2962 w2996 w3017 w3027 w3053 w3081 w3102 w3123 w3144 w3165 w3193 w3213 w3240 w3260 w3284 w3318 w3351]
            tunnel: w1172 -> [w1207 w1226 w1244 w1303 w1351 w1419 w1483 w1547 w1611 w1675 w1718 w1762 w1788 w1844 w1863 w1889 w1918 w1949 w1980 w2014 w2038 w2064 w2094 w2132 w2162 w2193 w2221 w2240 w2259 w2278 w2297 w2344 w2381 w2412 w2439 w2458 w2477 w2496 w2515 w2541 w2612 w2649 w2672 w2707 w2734 w2761 w2785 w2802 w2835 w2859 w2876 w2899 w2907 w2961 w2995 w3016 w3028 w3054 w3080 w3101 w3122 w3143 w3164 w3192 w3212 w3239 w3259 w3283 w3317 w3350]
            tunnel: w1171 -> [w1206 w1225 w1245 w1302 w1350 w1418 w1482 w1546 w1610 w1674 w1717 w1761 w1787 w1843 w1862 w1888 w1919 w1948 w1981 w2015 w2039 w2065 w2095 w2131 w2161 w2192 w2220 w2239 w2258 w2277 w2296 w2343 w2382 w2411 w2438 w2457 w2476 w2495 w2514 w2559 w2616 w2648 w2671 w2706 w2733 w2760 w2784 w2801 w2834 w2858 w2877 w2900 w2906 w2960 w2994 w3015 w3029 w3055 w3079 w3100 w3121 w3142 w3163 w3191 w3211 w3238 w3258 w3282 w3316 w3349]
            tunnel: [w1208 w1227 w1243 w1304 w1352 w1420 w1484 w1548 w1612 w1676 w1719 w1763 w1789 w1845 w1864 w1890 w1917 w1950 w1979 w2013 w2037 w2063 w2093 w2109 w2141 w2194 w2222 w2241 w2260 w2279 w2298 w2310 w2357 w2413 w2440 w2459 w2478 w2497 w2516 w2540 w2613 w2650 w2673 w2708 w2735 w2762 w2786 w2803 w2836 w2860 w2875 w2898 w2908 w2962 w2996 w3017 w3027 w3053 w3081 w3102 w3123 w3144 w3165 w3193 w3213 w3240 w3260 w3284 w3318 w3351] -> w1160
            tunnel: [w1207 w1226 w1244 w1303 w1351 w1419 w1483 w1547 w1611 w1675 w1718 w1762 w1788 w1844 w1863 w1889 w1918 w1949 w1980 w2014 w2038 w2064 w2094 w2132 w2162 w2193 w2221 w2240 w2259 w2278 w2297 w2344 w2381 w2412 w2439 w2458 w2477 w2496 w2515 w2541 w2612 w2649 w2672 w2707 w2734 w2761 w2785 w2802 w2835 w2859 w2876 w2899 w2907 w2961 w2995 w3016 w3028 w3054 w3080 w3101 w3122 w3143 w3164 w3192 w3212 w3239 w3259 w3283 w3317 w3350] -> w1159
            tunnel: [w1206 w1225 w1245 w1302 w1350 w1418 w1482 w1546 w1610 w1674 w1717 w1761 w1787 w1843 w1862 w1888 w1919 w1948 w1981 w2015 w2039 w2065 w2095 w2131 w2161 w2192 w2220 w2239 w2258 w2277 w2296 w2343 w2382 w2411 w2438 w2457 w2476 w2495 w2514 w2559 w2616 w2648 w2671 w2706 w2733 w2760 w2784 w2801 w2834 w2858 w2877 w2900 w2906 w2960 w2994 w3015 w3029 w3055 w3079 w3100 w3121 w3142 w3163 w3191 w3211 w3238 w3258 w3282 w3316 w3349] -> w1158
            tunnel: w1121 -> [w1204 w1223 w1242 w1268 w1325 w1394 w1480 w1544 w1608 w1672 w1715 w1759 w1784 w1818 w1869 w1878 w1915 w1921 w1964 w1994 w2021 w2049 w2079 w2121 w2146 w2185 w2218 w2236 w2256 w2275 w2294 w2314 w2377 w2404 w2437 w2455 w2474 w2493 w2512 w2526 w2593 w2632 w2668 w2679 w2732 w2752 w2782 w2800 w2825 w2857 w2874 w2887 w2911 w2933 w2968 w3012 w3031 w3056 w3075 w3096 w3117 w3138 w3149 w3179 w3198 w3222 w3254 w3270 w3293 w3326]
            tunnel: w1118 -> [w1203 w1222 w1241 w1299 w1347 w1414 w1478 w1542 w1606 w1670 w1713 w1757 w1777 w1838 w1868 w1887 w1914 w1929 w1962 w2001 w2027 w2053 w2083 w2124 w2159 w2184 w2216 w2238 w2255 w2274 w2293 w2332 w2379 w2402 w2432 w2456 w2473 w2492 w2511 w2552 w2614 w2646 w2670 w2700 w2728 w2753 w2780 w2799 w2827 w2854 w2873 w2897 w2914 w2932 w2987 w3011 w3032 w3057 w3074 w3095 w3116 w3137 w3150 w3187 w3207 w3218 w3253 w3278 w3312 w3345]
            tunnel: [w1204 w1223 w1242 w1268 w1325 w1393 w1480 w1544 w1608 w1672 w1715 w1759 w1784 w1824 w1853 w1878 w1903 w1921 w1964 w1994 w2020 w2048 w2078 w2125 w2145 w2186 w2217 w2236 w2256 w2275 w2294 w2339 w2376 w2403 w2435 w2455 w2474 w2493 w2512 w2553 w2590 w2647 w2667 w2701 w2731 w2754 w2781 w2800 w2828 w2856 w2874 w2886 w2910 w2933 w2966 w3012 w3031 w3056 w3075 w3096 w3117 w3138 w3149 w3179 w3198 w3222 w3254 w3270 w3293 w3326] -> w1155
            tunnel: [w1203 w1222 w1241 w1298 w1346 w1409 w1478 w1542 w1606 w1670 w1713 w1757 w1777 w1838 w1867 w1887 w1913 w1929 w1962 w2001 w2027 w2053 w2083 w2124 w2159 w2184 w2216 w2238 w2255 w2274 w2293 w2332 w2379 w2402 w2432 w2456 w2473 w2492 w2511 w2552 w2614 w2646 w2670 w2700 w2728 w2753 w2780 w2799 w2827 w2854 w2873 w2897 w2914 w2932 w2987 w3011 w3032 w3057 w3074 w3095 w3116 w3137 w3150 w3187 w3207 w3221 w3253 w3278 w3312 w3345] -> w1168
            tunnel: [_ _ _ _ _ _ _ _ _ _ _ _ _ _ _ _ _ _ _ _ _ _ _ _ _ _ _ _ _ _ _ _ _ _ _ _ _ _ _ _ _ _ w2661 _ _ _ _ _ _ _ _ _ _ _ _ _ _ _ _ _ _ _ _ _ _ _ _ _ _ _] -> w1052
            tunnel: [_ _ _ _ _ _ _ _ _ _ _ _ _ _ _ _ _ _ _ _ _ _ _ _ _ _ _ _ _ _ _ _ _ _ _ _ _ _ _ _ _ _ w2662 _ _ _ _ _ _ _ _ _ _ _ _ _ _ _ _ _ _ _ _ _ _ _ _ _ _ _] -> w1132
            tunnel: w1167 -> [w1201 w1220 w1239 w1270 w1327 w1415 w1479 w1543 w1607 w1671 w1714 w1758 w1782 w1839 w1865 w1880 w1911 w1941 w1977 w2011 w2017 w2045 w2075 w2123 w2158 w2181 w2212 w2237 w2253 w2272 w2291 w2338 w2378 w2401 w2430 w2452 w2471 w2490 w2509 w2551 w2610 w2638 w2669 w2681 w2725 w2750 w2778 w2797 w2826 w2853 w2871 w2889 w2916 w2958 w2979 w3009 w3034 w3059 w3072 w3093 w3114 w3135 w3159 w3173 w3200 w3228 w3247 w3272 w3306 w3339]
            tunnel: [w1201 w1220 w1239 w1270 w1327 w1415 w1479 w1543 w1607 w1671 w1714 w1758 w1782 w1839 w1865 w1877 w1911 w1941 w1977 w2011 w2017 w2045 w2075 w2123 w2158 w2181 w2212 w2237 w2253 w2272 w2291 w2338 w2378 w2401 w2430 w2452 w2471 w2490 w2509 w2551 w2610 w2638 w2669 w2680 w2725 w2750 w2778 w2797 w2826 w2853 w2871 w2888 w2916 w2958 w2979 w3009 w3034 w3059 w3072 w3093 w3114 w3135 w3159 w3173 w3200 w3228 w3247 w3272 w3306 w3339] -> w1166
            tunnel: w1165 -> [w1202 w1221 w1240 w1269 w1326 w1416 w1476 w1540 w1604 w1668 w1711 w1755 w1783 w1840 w1866 w1886 w1912 w1920 w1978 w2012 w2025 w2051 w2081 w2120 w2140 w2182 w2213 w2234 w2254 w2273 w2292 w2337 w2356 w2400 w2431 w2453 w2472 w2491 w2510 w2550 w2611 w2639 w2664 w2698 w2726 w2749 w2779 w2798 w2823 w2852 w2872 w2896 w2915 w2959 w2986 w3010 w3033 w3058 w3073 w3094 w3115 w3136 w3160 w3186 w3206 w3234 w3245 w3277 w3311 w3344]
            tunnel: [w1202 w1221 w1240 w1269 w1326 w1416 w1477 w1541 w1605 w1669 w1712 w1756 w1783 w1840 w1866 w1886 w1912 w1920 w1978 w2012 w2025 w2051 w2081 w2120 w2140 w2182 w2213 w2234 w2254 w2273 w2292 w2337 w2356 w2400 w2431 w2453 w2472 w2491 w2510 w2550 w2611 w2639 w2664 w2698 w2726 w2749 w2779 w2798 w2823 w2852 w2872 w2896 w2915 w2959 w2986 w3010 w3033 w3058 w3073 w3094 w3115 w3136 w3160 w3186 w3206 w3234 w3245 w3277 w3311 w3344] -> w1164
            tunnel: [_ _ _ _ _ _ _ _ _ _ _ _ _ _ _ _ _ _ _ _ _ _ _ _ _ _ _ _ _ _ _ _ _ _ _ _ _ _ _ _ _ _ _ _ _ _ _ _ _ _ _ _ _ _ _ TRUE _ _ _ _ _ _ _ _ _ _ _ _ _ _] -> w1161
            tunnel: w1151 -> [w1199 w1218 w1237 w1260 w1320 w1404 w1463 w1527 w1591 w1655 w1683 w1727 _ w1830 w1861 w1885 w1910 w1940 w1976 w2010 w2036 w2062 w2092 w2119 w2157 w2179 w2211 w2232 w2251 w2270 w2289 w2336 w2373 w2398 w2429 w2450 w2469 w2488 w2507 w2549 w2609 w2628 w2660 w2696 w2724 w2747 w2777 w2796 w2821 w2851 w2870 w2894 w2920 w2957 w2983 w3007 w3025 w3052 w3070 w3091 w3112 w3133 w3157 w3184 w3204 w3232 w3251 w3276 w3310 w3343]
            tunnel: w1150 -> [w1198 w1217 w1236 w1259 w1319 w1403 w1462 w1526 w1590 w1654 w1684 w1728 _ w1829 w1860 w1884 w1909 w1939 w1975 w2009 w2035 w2061 w2091 w2118 w2156 w2178 w2210 w2231 w2250 w2269 w2288 w2335 w2372 w2397 w2428 w2449 w2468 w2487 w2506 w2548 w2608 w2627 w2659 w2695 w2723 w2746 w2776 w2795 w2820 w2850 w2869 w2893 w2919 w2956 w2982 w3006 w3024 w3051 w3069 w3090 w3111 w3132 w3156 w3183 w3203 w3231 w3250 w3275 w3309 w3342]
            tunnel: w1149 -> [w1197 w1216 w1235 w1258 w1318 w1402 w1461 w1525 w1589 w1653 w1685 w1729 _ w1828 w1859 w1883 w1908 w1938 w1974 w2008 w2034 w2060 w2090 w2117 w2155 w2177 w2209 w2230 w2249 w2268 w2287 w2334 w2371 w2396 w2427 w2448 w2467 w2486 w2505 w2547 w2607 w2626 w2658 w2694 w2722 w2745 w2775 w2794 w2819 w2849 w2868 w2892 w2918 w2955 w2981 w3005 w3023 w3050 w3068 w3089 w3110 w3131 w3155 w3182 w3202 w3230 w3249 w3274 w3308 w3341]
            tunnel: w1148 -> [w1196 w1215 w1234 w1257 w1317 w1401 w1460 w1524 w1588 w1652 w1686 w1730 _ w1827 w1858 w1882 w1907 w1937 w1973 w2007 w2033 w2059 w2089 w2116 w2154 w2176 w2208 w2229 w2248 w2267 w2286 w2333 w2370 w2395 w2426 w2447 w2466 w2485 w2504 w2546 w2606 w2625 w2657 w2693 w2721 w2744 w2774 w2793 w2818 w2848 w2867 w2891 w2917 w2954 w2980 w3004 w3022 w3049 w3067 w3088 w3109 w3130 w3154 w3181 w3201 w3229 w3248 w3273 w3307 w3340]
            tunnel: w1147 -> [_ _ _ _ _ _ _ _ _ _ _ _ _ _ _ _ _ _ _ _ _ _ _ _ _ _ _ _ _ _ _ _ w2375 _ _ _ _ _ _ _ _ _ _ _ _ _ _ _ _ _ _ _ _ _ _ _ _ _ _ _ _ _ _ _ _ _ _ _ _ _]
            tunnel: w1146 -> [_ _ _ _ _ _ _ _ _ _ _ _ _ _ _ _ _ _ _ _ _ _ _ _ _ _ _ _ _ _ _ _ w2374 _ _ _ _ _ _ _ _ _ _ _ _ _ _ _ _ _ _ _ _ _ _ _ _ _ _ _ _ _ _ _ _ _ _ _ _ _]
            tunnel: [w1199 w1218 w1237 w1260 w1320 w1404 w1463 w1527 w1591 w1655 w1683 w1727 w1776 w1830 w1861 w1885 w1910 w1940 w1976 w2010 w2036 w2062 w2092 w2119 w2157 w2179 w2211 w2232 w2251 w2270 w2289 w2336 w2373 w2398 w2429 w2450 w2469 w2488 w2507 w2549 w2609 w2628 w2660 w2696 w2724 w2747 w2777 w2796 w2821 w2851 w2870 w2894 w2920 w2957 w2983 w3007 w3025 w3052 w3070 w3091 w3112 w3133 w3157 w3184 w3204 w3232 w3251 w3276 w3310 w3343] -> w1143
            tunnel: [w1198 w1217 w1236 w1259 w1319 w1403 w1462 w1526 w1590 w1654 w1684 w1728 w1767 w1829 w1860 w1884 w1909 w1939 w1975 w2009 w2035 w2061 w2091 w2118 w2156 w2178 w2210 w2231 w2250 w2269 w2288 w2335 w2372 w2397 w2428 w2449 w2468 w2487 w2506 w2548 w2608 w2627 w2659 w2695 w2723 w2746 w2776 w2795 w2820 w2850 w2869 w2893 w2919 w2956 w2982 w3006 w3024 w3051 w3069 w3090 w3111 w3132 w3156 w3183 w3203 w3231 w3250 w3275 w3309 w3342] -> w1115
            tunnel: [w1197 w1216 w1235 w1258 w1318 w1402 w1461 w1525 w1589 w1653 w1685 w1729 w1775 w1828 w1859 w1883 w1908 w1938 w1974 w2008 w2034 w2060 w2090 w2117 w2155 w2177 w2209 w2230 w2249 w2268 w2287 w2334 w2371 w2396 w2427 w2448 w2467 w2486 w2505 w2547 w2607 w2626 w2658 w2694 w2722 w2745 w2775 w2794 w2819 w2849 w2868 w2892 w2918 w2955 w2981 w3005 w3023 w3050 w3068 w3089 w3110 w3131 w3155 w3182 w3202 w3230 w3249 w3274 w3308 w3341] -> w1144
            tunnel: [w1196 w1215 w1234 w1257 w1317 w1401 w1460 w1524 w1588 w1652 w1686 w1730 w1765 w1827 w1858 w1882 w1907 w1937 w1973 w2007 w2033 w2059 w2089 w2116 w2154 w2176 w2208 w2229 w2248 w2267 w2286 w2333 w2370 w2395 w2426 w2447 w2466 w2485 w2504 w2546 w2606 w2625 w2657 w2693 w2721 w2744 w2774 w2793 w2818 w2848 w2867 w2891 w2917 w2954 w2980 w3004 w3022 w3049 w3067 w3088 w3109 w3130 w3154 w3181 w3201 w3229 w3248 w3273 w3307 w3340] -> w1145
            tunnel: [_ _ _ _ _ _ _ _ _ _ _ _ _ _ _ _ _ _ _ _ _ _ _ _ _ _ _ _ _ _ _ w2323 w2375 _ _ _ _ _ _ _ _ _ _ _ _ _ _ _ _ _ _ _ _ _ _ _ _ _ _ _ _ _ _ _ _ _ _ _ _ _] -> w1117
            tunnel: [_ _ _ _ _ _ _ _ _ _ _ _ _ _ _ _ _ _ _ _ _ _ _ _ _ _ _ _ _ _ _ w2322 w2374 _ _ _ _ _ _ _ _ _ _ _ _ _ _ _ _ _ _ _ _ _ _ _ _ _ _ _ _ _ _ _ _ _ _ _ _ _] -> w1116
            tunnel: w1128 -> [w1195 w1214 w1233 w1256 w1316 w1400 w1459 w1523 w1587 w1651 w1682 w1726 w1774 w1837 w1857 w1881 w1906 w1923 w1966 w1993 w2019 w2047 w2077 w2115 w2153 w2175 w2207 w2228 w2247 w2266 w2285 w2321 w2369 w2394 w2425 w2446 w2465 w2484 w2503 w2545 w2605 w2622 w2656 w2692 w2720 w2741 w2768 w2792 w2815 w2842 w2866 w2885 w2913 w2947 w2978 w3003 w3035 w3060 w3071 w3092 w3113 w3134 w3158 w3185 w3205 w3233 w3252 w3267 w3305 w3338]
            tunnel: [w1195 w1214 w1233 w1256 w1316 w1400 w1459 w1523 w1587 w1651 w1682 w1726 w1774 w1837 w1857 w1881 w1906 w1922 w1965 w1986 w2018 w2046 w2076 w2115 w2153 w2175 w2207 w2228 w2247 w2266 w2285 w2321 w2369 w2394 w2425 w2446 w2465 w2484 w2503 w2545 w2605 w2622 w2656 w2692 w2720 w2741 w2768 w2792 w2815 w2842 w2866 w2885 w2912 w2947 w2978 w3003 w3035 w3060 w3071 w3092 w3113 w3134 w3158 w3185 w3205 w3233 w3252 w3267 w3305 w3338] -> w1127
            tunnel: [w1194 w1213 w1232 w1255 w1315 w1399 w1458 w1522 w1586 w1650 w1681 w1725 w1773 w1836 w1856 w1892 w1905 w1943 w1972 w2006 w2032 w2058 w2088 w2114 w2152 w2174 w2206 w2227 w2246 w2265 w2284 w2320 w2368 w2393 w2424 w2445 w2464 w2483 w2502 w2544 w2604 w2621 w2655 w2691 w2719 w2740 w2767 w2791 w2814 w2841 w2865 w2884 w2905 w2953 w2977 w3001 w3036 w3046 w3066 w3087 w3108 w3129 w3153 w3189 w3209 w3236 w3256 w3280 w3314 w3347] -> w1126
            tunnel: [w1193 w1212 w1231 w1254 w1314 w1398 w1457 w1521 w1585 w1649 w1680 w1724 w1772 w1835 w1855 w1891 w1904 w1942 w1971 w2005 w2031 w2057 w2087 w2113 w2151 w2173 w2205 w2226 w2245 w2264 w2283 w2319 w2367 w2392 w2423 w2444 w2463 w2482 w2501 w2543 w2603 w2620 w2654 w2690 w2718 w2739 w2766 w2790 w2813 w2840 w2864 w2883 w2904 w2952 w2976 w3002 w3018 w3043 w3076 w3097 w3118 w3139 w3161 w3188 w3208 w3235 w3255 w3279 w3313 w3346] -> w1125
            tunnel: w1124 -> [w1194 w1213 w1232 w1255 w1315 w1399 w1458 w1522 w1586 w1650 w1681 w1725 w1773 w1836 w1856 w1892 w1905 w1943 w1972 w2006 w2032 w2058 w2088 w2114 w2152 w2174 w2206 w2227 w2246 w2265 w2284 w2320 w2368 w2393 w2424 w2445 w2464 w2483 w2502 w2544 w2604 w2621 w2655 w2691 w2719 w2740 w2767 w2791 w2814 w2841 w2865 w2884 w2905 w2953 w2977 w3001 _ w3046 w3066 w3087 w3108 w3129 w3153 w3189 w3209 w3236 w3256 w3280 w3314 w3347]
            tunnel: w1123 -> [w1193 w1212 w1231 w1254 w1314 w1398 w1457 w1521 w1585 w1649 w1680 w1724 w1772 w1835 w1855 w1891 w1904 w1942 w1971 w2005 w2031 w2057 w2087 w2113 w2151 w2173 w2205 w2226 w2245 w2264 w2283 w2319 w2367 w2392 w2423 w2444 w2463 w2482 w2501 w2543 w2603 w2620 w2654 w2690 w2718 w2739 w2766 w2790 w2813 w2840 w2864 w2883 w2904 w2952 w2976 w3002 _ w3043 w3076 w3097 w3118 w3139 w3161 w3188 w3208 w3235 w3255 w3279 w3313 w3346]
            tunnel: w1122 -> [_ _ _ _ _ _ _ _ _ _ _ _ _ _ _ _ _ _ _ _ _ _ _ _ _ _ _ _ _ _ _ _ _ _ _ _ _ _ _ _ _ _ _ _ _ _ _ _ _ _ _ _ _ _ _ _ _ _ w3064 w3085 w3106 w3127 w3151 _ _ _ _ _ _ _]
            tunnel: w1120 -> [_ _ _ _ _ _ _ _ _ _ _ _ _ _ _ _ _ _ _ w1998 _ w2044 w2074 w2103 w2139 w2167 w2198 _ _ _ _ w2303 w2353 w2388 w2417 _ _ _ _ _ _ _ _ _ _ _ _ _ _ _ _ _ _ _ _ _ _ _ _ _ _ _ _ _ _ _ _ _ _ _]
            tunnel: w1119 -> [_ _ _ _ _ _ _ _ _ _ _ _ _ _ _ _ _ _ _ _ _ _ _ _ _ _ _ _ _ _ _ _ _ _ _ _ _ _ _ _ _ _ _ _ _ _ _ _ _ _ _ _ _ _ _ _ _ _ _ _ _ _ _ _ _ w3223 _ _ _ _]
            tunnel: [w1192 w1211 w1230 w1253 w1313 w1397 w1456 w1520 w1584 w1648 w1679 w1723 w1771 w1834 w1851 w1875 w1901 w1944 w1970 w2004 w2030 w2056 w2086 w2112 w2150 w2172 w2204 w2225 w2244 w2263 w2282 w2318 w2366 w2391 w2422 w2443 w2462 w2481 w2500 w2539 w2602 w2619 w2653 w2675 w2717 w2738 w2765 w2789 w2812 w2839 w2863 w2882 w2903 w2950 w2963 w3000 w3021 w3045 w3063 w3084 w3105 w3126 w3148 w3168 w3197 w3217 w3244 w3265 w3304 w3337] -> w1113
            tunnel: w1114 -> [w1192 w1211 w1230 w1253 w1313 w1397 w1456 w1520 w1584 w1648 w1679 w1723 w1771 w1834 w1851 _ w1901 w1944 w1970 w2004 w2030 w2056 w2086 w2112 w2150 w2172 w2204 w2225 w2244 w2263 w2282 w2318 w2366 w2391 w2422 w2443 w2462 w2481 w2500 w2539 w2602 w2619 w2653 w2675 w2717 w2738 w2765 w2789 w2812 w2839 w2863 w2882 w2903 w2950 w2964 w3000 w3021 w3045 w3063 w3084 w3105 w3126 w3148 w3168 w3197 w3217 w3244 w3265 w3304 w3337]
            tunnel: w1112 -> [w1191 w1210 w1229 w1252 w1312 w1396 w1455 w1519 w1583 w1647 w1678 w1722 w1770 w1833 w1850 w1874 w1900 w1936 w1969 w2003 w2029 w2055 w2085 w2111 w2149 w2171 w2203 w2224 w2243 w2262 w2281 w2317 w2365 w2390 w2421 w2442 w2461 w2480 w2499 w2538 w2601 w2618 w2652 w2689 w2716 w2737 w2764 w2788 w2811 w2838 w2862 w2881 w2902 w2949 w2975 w2999 w3020 w3048 w3062 w3083 w3104 w3125 w3147 w3167 w3196 w3216 w3243 w3264 w3303 w3336]
            tunnel: w1111 -> [w1190 w1209 w1228 w1251 w1311 w1395 w1454 w1518 w1582 w1646 w1677 w1721 w1769 w1832 w1849 w1873 w1899 w1935 w1968 w2002 w2028 w2054 w2084 w2110 w2148 w2170 w2202 w2223 w2242 w2261 w2280 w2316 w2364 w2389 w2420 w2441 w2460 w2479 w2498 w2537 w2600 w2617 w2651 w2686 w2715 w2736 w2763 w2787 w2810 w2837 w2861 w2880 w2901 w2948 w2974 w2998 w3019 w3047 w3061 w3082 w3103 w3124 w3146 w3166 w3195 w3215 w3242 w3263 w3302 w3335]
            tunnel: [w1191 w1210 w1229 w1252 w1312 w1396 w1455 w1519 w1583 w1647 w1678 w1722 w1770 w1833 w1850 w1874 w1900 w1936 w1969 w2003 w2029 w2055 w2085 w2111 w2149 w2171 w2203 w2224 w2243 w2262 w2281 w2317 w2365 w2390 w2421 w2442 w2461 w2480 w2499 w2538 w2601 w2618 w2652 w2688 w2716 w2737 w2764 w2788 w2811 w2838 w2862 w2881 w2902 w2949 w2975 w2999 w3020 w3048 w3062 w3083 w3104 w3125 w3147 w3167 w3196 w3216 w3243 w3264 w3303 w3336] -> w1110
            tunnel: [w1190 w1209 w1228 w1251 w1311 w1395 w1454 w1518 w1582 w1646 w1677 w1721 w1769 w1832 w1849 w1873 w1899 w1935 w1968 w2002 w2028 w2054 w2084 w2110 w2148 w2170 w2202 w2223 w2242 w2261 w2280 w2316 w2364 w2389 w2420 w2441 w2460 w2479 w2498 w2537 w2600 w2617 w2651 w2687 w2715 w2736 w2763 w2787 w2810 w2837 w2861 w2880 w2901 w2948 w2974 w2998 w3019 w3047 w3061 w3082 w3103 w3124 w3146 w3166 w3195 w3215 w3242 w3263 w3302 w3335] -> w1109
            tunnel: w1108 -> [_ _ _ _ _ _ _ _ _ _ _ _ _ w1825 _ _ _ w1947 w1958 _ _ _ _ _ _ _ _ _ _ _ _ _ w2361 _ _ _ _ _ _ w2535 w2599 _ _ _ _ _ _ _ w2809 _ _ _ _ w2929 _ _ _ _ _ _ _ _ _ _ _ _ _ _ _ _]
            tunnel: w1107 -> [_ _ _ _ _ _ _ _ _ _ _ _ _ w1826 _ _ _ w1946 w1957 _ _ _ _ _ _ _ _ _ _ _ _ _ w2360 _ _ _ _ _ _ w2536 w2598 _ _ _ _ _ _ _ w2808 _ _ _ _ w2928 _ _ _ _ _ _ _ _ _ _ _ _ _ _ _ _]
            tunnel: w1105 -> [_ _ _ _ _ _ _ _ _ _ _ _ _ _ _ _ _ _ _ w1997 _ w2043 w2073 w2102 w2138 w2166 w2199 _ _ _ _ w2302 w2352 w2387 w2416 _ _ _ _ _ _ _ _ _ _ _ _ _ _ _ _ _ _ _ _ _ _ _ _ _ _ _ _ _ _ _ _ _ _ _]
            tunnel: w1104 -> [_ _ _ _ _ _ _ _ _ _ _ _ _ _ _ _ _ _ _ w1996 _ _ w2070 w2105 w2143 w2169 w2200 _ _ _ _ w2308 w2355 w2386 w2419 _ _ _ _ _ _ _ _ _ _ _ _ _ _ _ _ _ _ _ _ _ _ _ _ _ _ _ _ _ _ _ _ _ _ _]
            tunnel: w1103 -> [_ _ _ _ _ _ _ _ _ _ _ _ _ _ _ _ _ _ _ w1995 _ _ w2069 w2104 w2142 w2168 w2201 _ _ _ _ w2307 w2354 w2385 w2418 _ _ _ _ _ _ _ _ _ _ _ _ _ _ _ _ _ _ _ _ _ _ _ _ _ _ _ _ _ _ _ _ _ _ _]
            tunnel: [_ _ _ _ _ _ _ _ _ _ _ _ _ _ _ _ _ _ _ w1996 _ _ w2070 w2105 w2143 w2169 w2200 _ _ _ _ w2308 w2355 w2386 w2419 _ _ _ _ _ _ _ _ _ _ _ _ _ _ _ _ _ _ _ _ _ _ _ _ _ _ _ _ _ _ _ _ _ _ _] -> w1102
            tunnel: [_ _ _ _ _ _ _ _ _ _ _ _ _ _ _ _ _ _ _ w1995 _ _ w2069 w2104 w2142 w2168 w2201 _ _ _ _ w2307 w2354 w2385 w2418 _ _ _ _ _ _ _ _ _ _ _ _ _ _ _ _ _ _ _ _ _ _ _ _ _ _ _ _ _ _ _ _ _ _ _] -> w1101
            tunnel: [_ _ _ _ _ _ _ _ _ _ _ _ _ _ _ _ _ _ _ w1998 w2022 w2044 w2074 w2103 w2139 w2167 w2198 _ _ _ _ w2303 w2353 w2388 w2417 _ _ _ _ _ _ _ _ _ _ _ _ _ _ _ _ _ _ _ _ _ _ _ _ _ _ _ _ _ _ _ _ _ _ _] -> w1100
            tunnel: [_ _ _ _ _ _ _ _ _ _ _ _ _ _ _ _ _ _ _ w1997 w2023 w2043 w2073 w2102 w2138 w2166 w2199 _ _ _ _ w2302 w2352 w2387 w2416 _ _ _ _ _ _ _ _ _ _ _ _ _ _ _ _ _ _ _ _ _ _ _ _ _ _ _ _ _ _ _ _ _ _ _] -> w1099
            tunnel: [_ _ _ _ _ _ _ _ _ _ _ _ _ _ _ _ _ _ _ _ _ _ _ _ w2137 _ _ _ _ _ _ _ w2348 _ _ _ _ _ _ w2518 w2577 _ _ _ _ _ _ _ _ _ _ _ _ _ _ _ _ _ _ _ _ _ _ _ _ _ _ _ _ _] -> w1096
            tunnel: [_ _ _ _ _ _ _ _ _ _ _ _ _ _ _ _ _ _ _ _ _ _ _ _ w2136 _ _ _ _ _ _ _ w2347 _ _ _ _ _ _ w2517 w2578 _ _ _ _ _ _ _ _ _ _ _ _ _ _ _ _ _ _ _ _ _ _ _ _ _ _ _ _ _] -> w1098
            tunnel: [_ _ _ _ _ _ _ _ _ _ _ _ _ _ _ _ _ _ _ _ _ w2042 w2072 _ _ _ _ _ _ _ _ _ _ _ _ _ _ _ _ _ _ _ _ _ _ _ _ _ _ _ _ _ _ _ _ _ _ _ _ _ _ _ _ _ _ _ _ _ _ _] -> w1093
            tunnel: [_ _ _ _ _ _ _ _ _ _ _ _ _ _ _ _ _ _ _ _ _ _ TRUE ("Recording") _ _ _ _ _ _ _ _ _ _ _ _ _ _ _ _ _ _ _ _ _ _ _ _ _ _ _ _ _ _ _ _ _ _ _ _ _ _ _ _ _ _ _ _ _ _ _] -> w1090
            tunnel: [_ _ _ _ _ _ _ _ _ _ _ _ _ _ _ _ _ _ _ _ _ w2042 _ _ _ _ _ _ _ _ _ _ _ _ _ _ _ _ _ _ _ _ _ _ _ _ _ _ _ _ _ _ _ _ _ _ _ _ _ _ _ _ _ _ _ _ _ _ _ _] -> w1086
            tunnel: [_ _ _ _ _ _ _ _ _ _ _ _ _ _ TRUE _ _ _ _ _ _ _ _ _ _ _ _ _ _ _ _ _ _ _ _ _ _ _ _ _ _ _ _ _ _ _ _ _ _ _ _ _ _ _ _ _ _ _ _ _ _ _ _ _ _ _ _ _ _ _] -> w1083
            tunnel: [_ _ _ _ _ _ _ _ _ _ _ _ _ _ w1846 _ _ _ _ _ _ _ _ _ _ _ _ _ _ _ _ _ _ _ _ _ _ _ _ _ _ _ _ _ _ _ _ _ _ _ _ _ _ _ _ _ _ _ _ _ _ _ _ _ _ _ _ _ _ _] -> w1081
            tunnel: [_ _ _ _ _ _ _ _ _ _ _ _ _ _ _ _ TRUE _ _ _ _ _ _ _ _ _ _ _ _ _ _ _ _ _ _ _ _ _ _ _ _ _ _ _ _ _ _ _ _ _ _ _ _ _ _ _ _ _ _ _ _ _ _ _ _ _ _ _ _ _] -> w1080
            tunnel: [_ _ _ _ _ _ _ _ _ _ _ _ _ _ _ _ w1893 _ _ _ _ _ _ _ _ _ _ _ _ _ _ _ _ _ _ _ _ _ _ _ _ _ _ _ _ _ _ _ _ _ _ _ _ _ _ _ _ _ _ _ _ _ _ _ _ _ _ _ _ _] -> w1079
            tunnel: w1068 -> [_ _ _ _ _ _ _ _ _ _ _ _ _ _ _ _ _ _ _ w1984 _ _ _ w2098 w2135 w2165 w2197 _ _ _ _ w2301 w2351 w2384 w2415 _ _ _ _ w2521 w2572 _ _ _ _ _ _ _ _ _ _ _ _ _ _ _ _ _ _ _ _ _ _ _ _ _ _ _ _ _]
            tunnel: [_ _ _ _ _ _ _ _ _ _ _ _ _ _ _ _ _ _ _ w1984 _ _ w2068 w2098 w2135 w2165 w2197 _ _ _ _ w2301 w2351 w2384 w2415 _ _ _ _ w2521 w2572 _ _ _ _ _ _ _ _ _ _ _ _ _ _ _ _ _ _ _ _ _ _ _ _ _ _ _ _ _] -> w1067
            tunnel: w1066 -> [_ _ _ _ _ _ _ _ _ _ _ _ _ _ _ _ _ _ _ w1983 _ _ _ w2097 w2134 w2164 w2196 _ _ _ _ w2300 w2350 w2383 w2414 _ _ _ _ w2519 w2576 _ _ _ _ _ _ _ _ _ _ _ _ _ _ _ _ _ _ _ _ _ _ _ _ _ _ _ _ _]
            tunnel: [_ _ _ _ _ _ _ _ _ _ _ _ _ _ _ _ _ _ _ w1983 _ _ w2067 w2097 w2134 w2164 w2196 _ _ _ _ w2300 w2350 w2383 w2414 _ _ _ _ w2519 w2576 _ _ _ _ _ _ _ _ _ _ _ _ _ _ _ _ _ _ _ _ _ _ _ _ _ _ _ _ _] -> w1065
            tunnel: w1060 -> [_ _ _ _ _ _ _ _ _ _ _ _ _ _ _ _ _ _ _ _ _ _ _ _ _ _ _ _ _ _ _ _ _ _ _ _ _ _ _ _ _ _ _ _ _ _ _ _ _ _ _ _ _ _ _ _ _ _ _ _ _ _ _ _ _ _ _ _ w3300 w3333]
            tunnel: [_ _ _ _ _ _ _ _ _ _ _ _ _ _ _ _ _ _ _ _ _ _ _ _ _ _ _ _ _ _ _ _ _ _ _ _ _ _ _ _ _ _ _ _ _ _ _ _ _ _ _ _ _ _ _ _ _ _ _ _ _ _ _ _ _ _ _ _ w3298 w3331] -> w1059
            tunnel: w1055 -> [_ _ _ _ _ _ _ _ _ _ _ _ _ _ _ _ _ _ _ w1982 w2016 w2041 w2066 w2096 w2133 w2163 w2195 _ _ _ _ w2299 w2349 _ _ _ _ _ _ _ _ _ _ _ _ _ _ _ _ _ _ _ _ _ _ _ _ _ _ _ _ _ _ _ _ _ _ _ _ _]
            tunnel: [_ _ _ _ _ _ _ _ _ _ _ _ _ _ _ _ _ _ w1953 w1982 w2016 w2040 w2066 w2096 w2133 w2163 w2195 _ _ _ _ w2299 w2349 _ _ _ _ _ _ _ _ _ _ _ _ _ _ _ _ _ _ _ _ _ _ _ _ _ _ _ _ _ _ _ _ _ _ _ _ _] -> w1054
            tunnel: [_ _ _ _ _ _ _ _ _ _ _ _ _ _ _ _ _ _ _ _ _ _ _ _ _ _ _ _ _ _ _ _ w2346 _ _ _ _ _ _ _ _ _ _ _ _ _ _ _ _ _ _ _ _ _ _ _ _ _ _ _ _ _ _ _ _ _ _ _ _ _] -> w1049
            tunnel: [_ _ _ _ _ _ _ _ _ _ _ _ _ _ _ _ _ _ _ _ _ _ _ _ _ _ _ _ _ _ _ _ w2345 _ _ _ _ _ _ _ _ _ _ _ _ _ _ _ _ _ _ _ _ _ _ _ _ _ _ _ _ _ _ _ _ _ _ _ _ _] -> w1048
            frame 0, Default {
            }
            frame 1 {
            }
            frame 2 {
            }
            frame 3 {
              n608 = call "myRIO_BRig_RT_dataExp_Audio_freq__L.vi"() -> ("output_Audio_freq__L"=w1276:i32)  [unwired: 11 in]
              n609 = call "myRIO_BRig_RT_dataExp_Audio_freq__R.vi"() -> ("output_Audio_freq__R"=w1275:i32)  [unwired: 11 in]
              n610 = call "myRIO_BRig_RT_dataExp_Audio_amp__L.vi"() -> ("output_Audio_amp__L"=w1274:i32)  [unwired: 11 in]
              n611 = call "myRIO_BRig_RT_dataExp_Audio_amp__R.vi"() -> ("output_Audio_amp__R"=w1272:i32)  [unwired: 11 in]
              n612 = call "myRIO_BRig_RT_dataExp_TPB_min__L.vi"() -> ("output_TPB_min__L"=w1284:i32)  [unwired: 11 in]
              n613 = call "myRIO_BRig_RT_dataExp_TPB_min__R.vi"() -> ("output_TPB_min__R"=w1282:i32)  [unwired: 11 in]
              n614 = call "myRIO_BRig_RT_dataExp_TPB_max__L.vi"() -> ("output_TPB_max__L"=w1280:i32)  [unwired: 11 in]
              n615 = call "myRIO_BRig_RT_dataExp_TPB_max__R.vi"() -> ("output_TPB_max__R"=w1278:i32)  [unwired: 11 in]
              n616 = call "myRIO_BRig_RT_dataExp_ItrialUntilReward.vi"() -> ("output_I_trialUntilReward"=w1297:i32)  [unwired: 11 in]
              n617 = call "myRIO_BRig_RT_dataExp_IblockUntilReward.vi"() -> ("output_I_blockUntilReward"=w1293:i32)  [unwired: 11 in]
              n618 = call "myRIO_BRig_RT_dataExp_CueCycles.vi"() -> ("output_CueCycles"=w1292:i32)  [unwired: 11 in]
              n619 = call "myRIO_BRig_RT_dataExp_ENL_min.vi"() -> ("output_ENL_min"=w1290:i32)  [unwired: 11 in]
              n620 = call "myRIO_BRig_RT_dataExp_ENL_max.vi"() -> ("output_ENL_max"=w1288:i32)  [unwired: 11 in]
              n621 = call "myRIO_BRig_RT_dataExp_ENL_penalty.vi"() -> ("output_ENL_penalty"=w1286:i32)  [unwired: 11 in]
              n622 = local read "Audio_Freq__L"() -> (w1250:u8)
              n623 = local read "Audio_Freq__R"() -> (w1248:u8)
              n624 = local read "Audio_Amp__L"() -> (w1273:u16)
              n625 = local read "TpB_Min_L"() -> (w1283:u16)
              n626 = local read "TpB_Min_R"() -> (w1281:u16)
              n627 = local read "TpB_Max_L"() -> (w1279:u16)
              n628 = local read "TpB_Max_R"() -> (w1277:u16)
              n629 = local read "Audio_Amp__R"() -> (w1271:u16)
              n630 = local read "TrialUntilReward"() -> (w1296:bool)
              n631 = local read "CueCycles"() -> (w1291:u16)
              n632 = local read "Tcycle_ENL_min"() -> (w1289:u16)
              n633 = local read "Tcycle_ENL_max"() -> (w1287:u16)
              n634 = local read "Tcycle_ENLPenalty"() -> (w1285:u16)
              n635 = To Unsigned Word Integer(number=w1248) -> (unsigned 16bit integer=w1247:u16)
              n636 = To Unsigned Word Integer(number=w1250) -> (unsigned 16bit integer=w1249:u16)
              n637 = Boolean To (0,1)(Boolean=w1296) -> (0, 1=w1295:i16)
              n638 = To Unsigned Word Integer(number=w1295) -> (unsigned 16bit integer=w1294:u16)
              n639 = local read "BUR_min"() -> (w1265:u16)
              n640 = local read "BUR_max"() -> (w1266:u16)
              n641 = Not Equal To 0?(x=w1265) -> (x != 0?=w1264:bool)
              n642 = Not Equal To 0?(x=w1266) -> (x != 0?=w1263:bool)
              n643 = And(x=w1264, y=w1263) -> (x .and. y?=w1262:bool)
              n644 = Boolean To (0,1)(Boolean=w1262) -> (0, 1=w1267:i16)
              n645 = To Unsigned Word Integer(number=w1267) -> (unsigned 16bit integer=w1261:u16)
              n646 = Replace Array Subset(array=w1299, new element #1=w1294, index #1=w1297, new element #2=w1261, index #2=w1293, new element #3=w1291, index #3=w1292, new element #4=w1289, index #4=w1290, new element #5=w1287, index #5=w1288, new element #6=w1285, index #6=w1286, new element #7=w1283, index #7=w1284, new element #8=w1281, index #8=w1282, new element #9=w1279, index #9=w1280, new element #10=w1277, index #10=w1278, new element #11=w1249, index #11=w1276, new element #12=w1247, index #12=w1275, new element #13=w1273, index #13=w1274, new element #14=w1271, index #14=w1272) -> (w1298:u16[])
            }
            frame 4 {
              n647 = call "myRIO_BRig_RT_dataExp_Tcycle_RewardPost.vi"() -> ("output_Tcycle_RewardPost"=w1336:i32)  [unwired: 11 in]
              n648 = call "myRIO_BRig_RT_dataExp_Tcycle_Wrong.vi"() -> ("output_Tcycle_Wrong"=w1334:i32)  [unwired: 11 in]
              n649 = call "myRIO_BRig_RT_dataExp_Tcycle_Timeout.vi"() -> ("output_Tcycle_Timeout"=w1332:i32)  [unwired: 11 in]
              n650 = call "myRIO_BRig_RT_dataExp_Tcycle_Cue_min.vi"() -> ("output_Tcycle_Cue_min"=w1330:i32)  [unwired: 11 in]
              n651 = call "myRIO_BRig_RT_dataExp_Tcycle_Cue_max.vi"() -> ("output_Tcycle_Cue_max"=w1329:i32)  [unwired: 11 in]
              n652 = call "myRIO_BRig_RT_dataExp_Tcycle_CuePenalty.vi"() -> ("output_Tcycle_CuePenalty"=w1328:i32)  [unwired: 11 in]
              n653 = call "myRIO_BRig_RT_dataExp_SolenoidProbability_L.vi"() -> ("output_SolenoidProbability_L"=w1308:i32)  [unwired: 11 in]
              n654 = call "myRIO_BRig_RT_dataExp_SolenoidProbability_R.vi"() -> ("output_SolenoidProbability_R"=w1307:i32)  [unwired: 11 in]
              n655 = call "myRIO_BRig_RT_dataExp_nBlock.vi"() -> ("output_nBlock"=w1345:i32)  [unwired: 11 in]
              n656 = call "myRIO_BRig_RT_dataExp_nTrial.vi"() -> ("output_nTrial"=w1344:i32)  [unwired: 11 in]
              n657 = call "myRIO_BRig_RT_dataExp_runTime_seconds.vi"() -> ("output_RunTime_minutes"=w1343:i32)  [unwired: 11 in]
              n658 = call "myRIO_BRig_RT_dataExp_Tcycle_Selection.vi"() -> ("output_Tcycle_Selection"=w1342:i32)  [unwired: 11 in]
              n659 = call "myRIO_BRig_RT_dataExp_Tcycle_Reward__L.vi"() -> ("output_Tcycle_Reward__L"=w1340:i32)  [unwired: 11 in]
              n660 = call "myRIO_BRig_RT_dataExp_Tcycle_Reward__R.vi"() -> ("output_Tcycle_Reward__R"=w1338:i32)  [unwired: 11 in]
              n661 = local read "Tcycle_RewardPost"() -> (w1335:u16)
              n662 = local read "Tcycle_Wrong"() -> (w1333:u16)
              n663 = local read "Tcycle_Timeout"() -> (w1331:u16)
              n664 = local read "Tcycle_CuePenalty"() -> (w1321:u16)
              n665 = local read "Tcycle_Cue_max"() -> (w1309:u16)
              n666 = local read "Tcycle_Cue_min"() -> (w1310:u16)
              n667 = local read "Tcycle_Selection"() -> (w1341:u16)
              n668 = local read "Tcycle_Reward_L"() -> (w1339:u16)
              n669 = local read "Tcycle_Reward_R"() -> (w1337:u16)
              n670 = local read "SolenoidProbability_R"() -> (w1305:u16)
              n671 = local read "SolenoidProbability_L"() -> (w1306:u16)
              n672 = Replace Array Subset(array=w1347, new element #1=u16 0, index #1=w1345, new element #2=u16 0, index #2=w1344, new element #3=u16 0, index #3=w1343, new element #4=w1341, index #4=w1342, new element #5=w1339, index #5=w1340, new element #6=w1337, index #6=w1338, new element #7=w1335, index #7=w1336, new element #8=w1333, index #8=w1334, new element #9=w1331, index #9=w1332, new element #10=w1310, index #10=w1330, new element #11=w1309, index #11=w1329, new element #12=w1321, index #12=w1328, new element #13=w1306, index #13=w1308, new element #14=w1305, index #14=w1307) -> (w1346:u16[])
            }
            frame 5 {
              w1358 = 100.0 ("y")
              n673 = call "myRIO_BRig_RT_dataExp_laser1_Freq.vi"() -> ("output_laser1_Freq"=w1391:i32)  [unwired: 11 in]
              n674 = call "myRIO_BRig_RT_dataExp_laser1_Tpeak.vi"() -> ("output_laser1_Tpeak"=w1386:i32)  [unwired: 11 in]
              n675 = call "myRIO_BRig_RT_dataExp_laser1_Tshutter.vi"() -> ("output_laser1_Tshutter"=w1381:i32)  [unwired: 11 in]
              n676 = call "myRIO_BRig_RT_dataExp_FPGA_f_count2ms.vi"() -> ("output_FPGA_f_count2ms"=w1376:i32)  [unwired: 11 in]
              n677 = call "myRIO_BRig_RT_dataExp_laser1_Power_min.vi"() -> ("output_laser1_Power_min"=w1371:i32)  [unwired: 11 in]
              n678 = call "myRIO_BRig_RT_dataExp_laser1_Power_max.vi"() -> ("output_laser1_Power_max"=w1364:i32)  [unwired: 11 in]
              n679 = call "myRIO_BRig_RT_dataExp_laser1_Power_step.vi"() -> ("output_laser1_Power_step"=w1363:i32)  [unwired: 11 in]
              n680 = call "myRIO_BRig_RT_dataExp_laser1_duration.vi"() -> ("output_laser1_duration"=w1366:i32)  [unwired: 11 in]
              n681 = call "myRIO_BRig_RT_dataExp_BUR_min.vi"() -> ("output_BUR_min"=w1413:i32)  [unwired: 11 in]
              n682 = call "myRIO_BRig_RT_dataExp_BUR_max.vi"() -> ("output_BUR_max"=w1411:i32)  [unwired: 11 in]
              n683 = call "myRIO_BRig_RT_dataExp_Audio_sp__L.vi"() -> ("output_Audio_sp__L"=w1408:i32)  [unwired: 11 in]
              n684 = call "myRIO_BRig_RT_dataExp_Audio_sp__R.vi"() -> ("output_Audio_sp__R"=w1407:i32)  [unwired: 11 in]
              n685 = local read "laser1_Tshutter"() -> (w1378:dbl)
              n686 = local read "laser1_Tpeak"() -> (w1383:dbl)
              n687 = local read "laser1_power_min"() -> (w1368:dbl)
              n688 = local read "laser1_power_max"() -> (w1357:dbl)
              n689 = local read "laser1_power_step"() -> (w1356:dbl)
              n690 = local read "FPGA_count2ms"() -> (w1373:dbl)
              n691 = local read "laser1_Freq"() -> (w1390:dbl)
              n692 = local read "sp_LeftSpout"() -> (w1406:u16)
              n693 = local read "BUR_max"() -> (w1410:u16)
              n694 = local read "sp_RightSpout"() -> (w1405:u16)
              n695 = local read "BUR_min"() -> (w1412:u16)
              n696 = Multiply(x=w1390, y=w1358) -> (x*y=w1389:dbl)
              n697 = Multiply(x=w1383, y=w1358) -> (x*y=w1385:dbl)
              n698 = Multiply(x=w1378, y=w1358) -> (x*y=w1380:dbl)
              n699 = Multiply(x=w1373, y=w1358) -> (x*y=w1375:dbl)
              n700 = Multiply(x=w1368, y=w1358) -> (x*y=w1370:dbl)
              n701 = Multiply(x=w1357, y=w1358) -> (x*y=w1362:dbl)
              n702 = Multiply(x=w1356, y=w1358) -> (x*y=w1360:dbl)
              n703 = Round To Nearest(number=w1389) -> (nearest integer value=w1388:dbl)
              n704 = Round To Nearest(number=w1385) -> (nearest integer value=w1384:dbl)
              n705 = Round To Nearest(number=w1380) -> (nearest integer value=w1379:dbl)
              n706 = Round To Nearest(number=w1375) -> (nearest integer value=w1374:dbl)
              n707 = Round To Nearest(number=w1370) -> (nearest integer value=w1369:dbl)
              n708 = Round To Nearest(number=w1362) -> (nearest integer value=w1361:dbl)
              n709 = Round To Nearest(number=w1360) -> (nearest integer value=w1359:dbl)
              n710 = To Unsigned Word Integer(number=w1388) -> (unsigned 16bit integer=w1387:u16)
              n711 = To Unsigned Word Integer(number=w1384) -> (unsigned 16bit integer=w1382:u16)
              n712 = To Unsigned Word Integer(number=w1379) -> (unsigned 16bit integer=w1377:u16)
              n713 = To Unsigned Word Integer(number=w1374) -> (unsigned 16bit integer=w1372:u16)
              n714 = To Unsigned Word Integer(number=w1369) -> (unsigned 16bit integer=w1367:u16)
              n715 = To Unsigned Word Integer(number=w1361) -> (unsigned 16bit integer=w1355:u16)
              n716 = To Unsigned Word Integer(number=w1359) -> (unsigned 16bit integer=w1354:u16)
              n717 = local read "laser1_duration"() -> (w1365:u16)
              n718 = call "myRIO_BRig_RT_dataCurrent_laser1_pulse_duration.vi"() -> ("output_laser1_pulse_duration"=w1392:i32)  [unwired: 11 in]
              n719 = Replace Array Subset(array=w1414, new element #1=w1412, index #1=w1413, new element #2=w1410, index #2=w1411, new element #3=w1406, index #3=w1408, new element #4=w1405, index #4=w1407, new element #5=w1387, index #5=w1391, new element #6=w1382, index #6=w1386, new element #7=w1377, index #7=w1381, new element #8=w1372, index #8=w1376, new element #9=w1367, index #9=w1371, new element #10=w1355, index #10=w1364, new element #11=w1354, index #11=w1363, new element #12=w1365, index #12=w1366) -> (w1409:u16[])
              n720 = Replace Array Subset(array=w1394, new element=w1365, index=w1392) -> (w1393:u16[])
            }
            frame 6 {
              # "Selection First"
              # "Count"
              # "Tdelay"
              # "Probability"
              # "OnOff"
              # "Block"
              # "delayOpt"
              # "Count"
              # "Tdelay"
              # "Probability"
              # "OnOff"
              # "Block"
              # "ENL1 All"
              # "delayOpt"
              # "Count"
              # "Tdelay"
              # "Probability"
              # "OnOff"
              # "Block"
              # "ENL1 First"
              n721 = call "myRIO_BRig_RT_dataLC_ENL1_Block_NS_l1.vi"() -> ("output_ENL1_All_Block"=w1449:i32)  [unwired: 11 in]
              n722 = call "myRIO_BRig_RT_dataLC_ENL1_OnOff_NS_l1.vi"() -> ("output_ENL1_OnOff_NS_l1"=w1439:i32)  [unwired: 11 in]
              n723 = call "myRIO_BRig_RT_dataLC_ENL1_Probability_NS_l1.vi"() -> ("output_ENL1_Probability_NS_l1"=w1438:i32)  [unwired: 11 in]
              n724 = call "myRIO_BRig_RT_dataLC_ENL1_Tdelay_NS_l1.vi"() -> ("output_ENL1_Tdelay_NS_l1"=w1437:i32)  [unwired: 11 in]
              n725 = call "myRIO_BRig_RT_dataLC_ENL1_Count_NS_l1.vi"() -> ("output_ENL1_Count_NS_l1"=w1436:i32)  [unwired: 11 in]
              n726 = call "myRIO_BRig_RT_dataLC_ENL1_delayOpt_NS_l1.vi"() -> ("output_ENL1_delayOpt_NS_l1"=w1435:i32)  [unwired: 11 in]
              n727 = local read "LC_l1_ENL1_First_delayOpt"() -> (w1452:bool)
              n728 = call "myRIO_BRig_RT_dataLC_ENL1_Block_Switch_l1.vi"() -> ("output_ENL1_Block_Switch_l1"=w1475:i32)  [unwired: 11 in]
              n729 = call "myRIO_BRig_RT_dataLC_ENL1_OnOff_Switch_l1.vi"() -> ("output_ENL1_OnOff_Switch_l1"=w1473:i32)  [unwired: 11 in]
              n730 = call "myRIO_BRig_RT_dataLC_ENL1_Probability_Switch_l1.vi"() -> ("output_ENL1_Probability_Switch_l1"=w1469:i32)  [unwired: 11 in]
              n731 = call "myRIO_BRig_RT_dataLC_ENL1_Tdelay_Switch_l1.vi"() -> ("output_ENL1_Tdelay_Switch_l1"=w1467:i32)  [unwired: 11 in]
              n732 = call "myRIO_BRig_RT_dataLC_ENL1_Count_Switch_l1.vi"() -> ("output_ENL1_Count_Switch_l1"=w1465:i32)  [unwired: 11 in]
              n733 = call "myRIO_BRig_RT_dataLC_ENL1_delayOpt_Switch_l1.vi"() -> ("output_ENL1_delayOpt_Switch_l1"=w1451:i32)  [unwired: 11 in]
              n734 = local read "LC_l1_ENL1_First_Count"() -> (w1464:u16)
              n735 = local read "LC_l1_ENL1_First_Probability"() -> (w1468:u16)
              n736 = local read "LC_l1_ENL1_First_Block"() -> (w1474:u16)
              n737 = local read "LC_l1_ENL1_First_Tdelay"() -> (w1466:u16)
              n738 = local read "LC_l1_ENL1_First_OnOff"() -> (w1472:bool)
              n739 = call "myRIO_BRig_RT_dataLC_Selection_Block_Switch_l1.vi"() -> ("output_Selection_Block_Switch_l1"=w1433:i32)  [unwired: 11 in]
              n740 = call "myRIO_BRig_RT_dataLC_Selection_OnOff_Switch_l1.vi"() -> ("output_Selection_OnOff_Switch_l1"=w1432:i32)  [unwired: 11 in]
              n741 = call "myRIO_BRig_RT_dataLC_Selection_Probability_Switch_l1.vi"() -> ("output_Selection_Probability_Switch_l1"=w1431:i32)  [unwired: 11 in]
              n742 = call "myRIO_BRig_RT_dataLC_Selection_Tdelay_Switch_l1.vi"() -> ("output_Selection_Tdelay_Switch_l1"=w1430:i32)  [unwired: 11 in]
              n743 = call "myRIO_BRig_RT_dataLC_Selection_Count_Switch_l1.vi"() -> ("output_Selection_Count_Switch_l1"=w1429:i32)  [unwired: 11 in]
              n744 = local read "LC_l1_ENL1_All_OnOff"() -> (w1445:bool)
              n745 = local read "LC_l1_ENL1_All_Probability"() -> (w1443:u16)
              n746 = local read "LC_l1_ENL1_All_delayOpt"() -> (w1441:bool)
              n747 = local read "LC_l1_ENL1_All_Tdelay"() -> (w1434:u16)
              n748 = local read "LC_l1_ENL1_All_Block"() -> (w1446:u16)
              n749 = local read "LC_l1_ENL1_All_Count"() -> (w1442:u16)
              n750 = local read "LC_l1_Sel_First_Probability"() -> (w1424:u16)
              n751 = local read "LC_l1_Sel_First_Tdelay"() -> (w1423:u16)
              n752 = local read "LC_l1_Sel_First_OnOff"() -> (w1427:bool)
              n753 = local read "LC_l1_Sel_First_Count"() -> (w1422:u16)
              n754 = local read "LC_l1_Sel_First_Block"() -> (w1426:u16)
              n755 = Boolean To (0,1)(Boolean=w1452) -> (0, 1=w1453:i16)
              n756 = Boolean To (0,1)(Boolean=w1472) -> (0, 1=w1471:i16)
              n757 = Boolean To (0,1)(Boolean=w1445) -> (0, 1=w1448:i16)
              n758 = To Unsigned Word Integer(number=w1453) -> (unsigned 16bit integer=w1450:u16)
              n759 = To Unsigned Word Integer(number=w1471) -> (unsigned 16bit integer=w1470:u16)
              n760 = Boolean To (0,1)(Boolean=w1441) -> (0, 1=w1447:i16)
              n761 = To Unsigned Word Integer(number=w1448) -> (unsigned 16bit integer=w1444:u16)
              n762 = Boolean To (0,1)(Boolean=w1427) -> (0, 1=w1428:i16)
              n763 = To Unsigned Word Integer(number=w1447) -> (unsigned 16bit integer=w1440:u16)
              n764 = To Unsigned Word Integer(number=w1428) -> (unsigned 16bit integer=w1425:u16)
              n765 = Replace Array Subset(array=w1476, new element #1=w1474, index #1=w1475, new element #2=w1470, index #2=w1473, new element #3=w1468, index #3=w1469, new element #4=w1466, index #4=w1467, new element #5=w1464, index #5=w1465, new element #6=w1450, index #6=w1451, new element #7=w1446, index #7=w1449, new element #8=w1444, index #8=w1439, new element #9=w1443, index #9=w1438, new element #10=w1434, index #10=w1437, new element #11=w1442, index #11=w1436, new element #12=w1440, index #12=w1435, new element #13=w1426, index #13=w1433, new element #14=w1425, index #14=w1432, new element #15=w1424, index #15=w1431, new element #16=w1423, index #16=w1430, new element #17=w1422, index #17=w1429) -> (w1477:u16[])
            }
            frame 7 {
              # "Selection First"
              # "Count"
              # "Tdelay"
              # "Probability"
              # "OnOff"
              # "Block"
              # "delayOpt"
              # "Count"
              # "Tdelay"
              # "Probability"
              # "OnOff"
              # "Block"
              # "ENL1 All"
              # "delayOpt"
              # "Count"
              # "Tdelay"
              # "Probability"
              # "OnOff"
              # "Block"
              # "ENL1 First"
              n766 = call "myRIO_BRig_RT_dataLC_ENL1_Block_NS_l1.vi"() -> ("output_ENL1_All_Block"=w1513:i32)  [unwired: 11 in]
              n767 = call "myRIO_BRig_RT_dataLC_ENL1_OnOff_NS_l1.vi"() -> ("output_ENL1_OnOff_NS_l1"=w1503:i32)  [unwired: 11 in]
              n768 = call "myRIO_BRig_RT_dataLC_ENL1_Probability_NS_l1.vi"() -> ("output_ENL1_Probability_NS_l1"=w1502:i32)  [unwired: 11 in]
              n769 = call "myRIO_BRig_RT_dataLC_ENL1_Tdelay_NS_l1.vi"() -> ("output_ENL1_Tdelay_NS_l1"=w1501:i32)  [unwired: 11 in]
              n770 = call "myRIO_BRig_RT_dataLC_ENL1_Count_NS_l1.vi"() -> ("output_ENL1_Count_NS_l1"=w1500:i32)  [unwired: 11 in]
              n771 = call "myRIO_BRig_RT_dataLC_ENL1_delayOpt_NS_l1.vi"() -> ("output_ENL1_delayOpt_NS_l1"=w1499:i32)  [unwired: 11 in]
              n772 = local read "LC_l1_ENL1_First_delayOpt"() -> (w1516:bool)
              n773 = call "myRIO_BRig_RT_dataLC_ENL1_Block_Switch_l1.vi"() -> ("output_ENL1_Block_Switch_l1"=w1539:i32)  [unwired: 11 in]
              n774 = call "myRIO_BRig_RT_dataLC_ENL1_OnOff_Switch_l1.vi"() -> ("output_ENL1_OnOff_Switch_l1"=w1537:i32)  [unwired: 11 in]
              n775 = call "myRIO_BRig_RT_dataLC_ENL1_Probability_Switch_l1.vi"() -> ("output_ENL1_Probability_Switch_l1"=w1533:i32)  [unwired: 11 in]
              n776 = call "myRIO_BRig_RT_dataLC_ENL1_Tdelay_Switch_l1.vi"() -> ("output_ENL1_Tdelay_Switch_l1"=w1531:i32)  [unwired: 11 in]
              n777 = call "myRIO_BRig_RT_dataLC_ENL1_Count_Switch_l1.vi"() -> ("output_ENL1_Count_Switch_l1"=w1529:i32)  [unwired: 11 in]
              n778 = call "myRIO_BRig_RT_dataLC_ENL1_delayOpt_Switch_l1.vi"() -> ("output_ENL1_delayOpt_Switch_l1"=w1515:i32)  [unwired: 11 in]
              n779 = local read "LC_l1_ENL1_First_Count"() -> (w1528:u16)
              n780 = local read "LC_l1_ENL1_First_Probability"() -> (w1532:u16)
              n781 = local read "LC_l1_ENL1_First_Block"() -> (w1538:u16)
              n782 = local read "LC_l1_ENL1_First_Tdelay"() -> (w1530:u16)
              n783 = local read "LC_l1_ENL1_First_OnOff"() -> (w1536:bool)
              n784 = call "myRIO_BRig_RT_dataLC_Selection_Block_Switch_l1.vi"() -> ("output_Selection_Block_Switch_l1"=w1497:i32)  [unwired: 11 in]
              n785 = call "myRIO_BRig_RT_dataLC_Selection_OnOff_Switch_l1.vi"() -> ("output_Selection_OnOff_Switch_l1"=w1496:i32)  [unwired: 11 in]
              n786 = call "myRIO_BRig_RT_dataLC_Selection_Probability_Switch_l1.vi"() -> ("output_Selection_Probability_Switch_l1"=w1495:i32)  [unwired: 11 in]
              n787 = call "myRIO_BRig_RT_dataLC_Selection_Tdelay_Switch_l1.vi"() -> ("output_Selection_Tdelay_Switch_l1"=w1494:i32)  [unwired: 11 in]
              n788 = call "myRIO_BRig_RT_dataLC_Selection_Count_Switch_l1.vi"() -> ("output_Selection_Count_Switch_l1"=w1493:i32)  [unwired: 11 in]
              n789 = local read "LC_l1_ENL1_All_OnOff"() -> (w1509:bool)
              n790 = local read "LC_l1_ENL1_All_Probability"() -> (w1507:u16)
              n791 = local read "LC_l1_ENL1_All_delayOpt"() -> (w1505:bool)
              n792 = local read "LC_l1_ENL1_All_Tdelay"() -> (w1498:u16)
              n793 = local read "LC_l1_ENL1_All_Block"() -> (w1510:u16)
              n794 = local read "LC_l1_ENL1_All_Count"() -> (w1506:u16)
              n795 = local read "LC_l1_Sel_First_Probability"() -> (w1488:u16)
              n796 = local read "LC_l1_Sel_First_Tdelay"() -> (w1487:u16)
              n797 = local read "LC_l1_Sel_First_OnOff"() -> (w1491:bool)
              n798 = local read "LC_l1_Sel_First_Count"() -> (w1486:u16)
              n799 = local read "LC_l1_Sel_First_Block"() -> (w1490:u16)
              n800 = Boolean To (0,1)(Boolean=w1516) -> (0, 1=w1517:i16)
              n801 = Boolean To (0,1)(Boolean=w1536) -> (0, 1=w1535:i16)
              n802 = Boolean To (0,1)(Boolean=w1509) -> (0, 1=w1512:i16)
              n803 = To Unsigned Word Integer(number=w1517) -> (unsigned 16bit integer=w1514:u16)
              n804 = To Unsigned Word Integer(number=w1535) -> (unsigned 16bit integer=w1534:u16)
              n805 = Boolean To (0,1)(Boolean=w1505) -> (0, 1=w1511:i16)
              n806 = To Unsigned Word Integer(number=w1512) -> (unsigned 16bit integer=w1508:u16)
              n807 = Boolean To (0,1)(Boolean=w1491) -> (0, 1=w1492:i16)
              n808 = To Unsigned Word Integer(number=w1511) -> (unsigned 16bit integer=w1504:u16)
              n809 = To Unsigned Word Integer(number=w1492) -> (unsigned 16bit integer=w1489:u16)
              n810 = Replace Array Subset(array=w1540, new element #1=w1538, index #1=w1539, new element #2=w1534, index #2=w1537, new element #3=w1532, index #3=w1533, new element #4=w1530, index #4=w1531, new element #5=w1528, index #5=w1529, new element #6=w1514, index #6=w1515, new element #7=w1510, index #7=w1513, new element #8=w1508, index #8=w1503, new element #9=w1507, index #9=w1502, new element #10=w1498, index #10=w1501, new element #11=w1506, index #11=w1500, new element #12=w1504, index #12=w1499, new element #13=w1490, index #13=w1497, new element #14=w1489, index #14=w1496, new element #15=w1488, index #15=w1495, new element #16=w1487, index #16=w1494, new element #17=w1486, index #17=w1493) -> (w1541:u16[])
            }
            frame 8 {
              # "Selection All"
              # "Count"
              # "Tdelay"
              # "Probability"
              # "OnOff"
              # "Block"
              # "delayOpt"
              # "Count"
              # "Tdelay"
              # "Probability"
              # "OnOff"
              # "Block"
              # "Cue1 All"
              # "delayOpt"
              # "Count"
              # "Tdelay"
              # "Probability"
              # "OnOff"
              # "Block"
              # "Cue1 First"
              n811 = call "myRIO_BRig_RT_dataLC_Cue1_delayOpt_Switch_l1.vi"() -> ("output_Cue1_delayOpt_Switch_l1"=w1580:i32)  [unwired: 11 in]
              n812 = call "myRIO_BRig_RT_dataLC_Cue1_Block_Switch_l1.vi"() -> ("output_Cue1_Block_Switch_l1"=w1603:i32)  [unwired: 11 in]
              n813 = call "myRIO_BRig_RT_dataLC_Cue1_OnOff_Switch_l1.vi"() -> ("output_Cue1_OnOff_Switch_l1"=w1601:i32)  [unwired: 11 in]
              n814 = call "myRIO_BRig_RT_dataLC_Cue1_Probability_Switch_l1.vi"() -> ("output_Cue1_Probability_Switch_l1"=w1597:i32)  [unwired: 11 in]
              n815 = call "myRIO_BRig_RT_dataLC_Cue1_Tdelay_Switch_l1.vi"() -> ("output_Cue1_Tdelay_Switch_l1"=w1595:i32)  [unwired: 11 in]
              n816 = call "myRIO_BRig_RT_dataLC_Cue1_Count_Switch_l1.vi"() -> ("output_Cue1_Count_Switch_l1"=w1593:i32)  [unwired: 11 in]
              n817 = call "myRIO_BRig_RT_dataLC_Cue1_Block_NS_l1.vi"() -> ("output_Cue1_Block_NS_l1"=w1577:i32)  [unwired: 11 in]
              n818 = call "myRIO_BRig_RT_dataLC_Cue1_OnOff_NS_l1.vi"() -> ("output_Cue1_OnOff_NS_l1"=w1576:i32)  [unwired: 11 in]
              n819 = call "myRIO_BRig_RT_dataLC_Cue1_Probability_NS_l1.vi"() -> ("output_Cue1_l1_All_Probability"=w1575:i32)  [unwired: 11 in]
              n820 = call "myRIO_BRig_RT_dataLC_Cue1_Tdelay_NS_l1.vi"() -> ("output_Cue1_Tdelay_NS_l1"=w1574:i32)  [unwired: 11 in]
              n821 = call "myRIO_BRig_RT_dataLC_Cue1_Count_NS_l1.vi"() -> ("output_Cue1_Count_NS_l1"=w1573:i32)  [unwired: 11 in]
              n822 = call "myRIO_BRig_RT_dataLC_Cue1_delayOpt_NS_l1.vi"() -> ("output_Cue1_delayOpt_NS_l1"=w1572:i32)  [unwired: 11 in]
              n823 = local read "LC_l1_Cue1_First_delayOpt"() -> (w1579:bool)
              n824 = local read "LC_l1_Cue1_First_Count"() -> (w1592:u16)
              n825 = local read "LC_l1_Cue1_First_Probability"() -> (w1596:u16)
              n826 = local read "LC_l1_Cue1_First_Block"() -> (w1602:u16)
              n827 = local read "LC_l1_Cue1_First_Tdelay"() -> (w1594:u16)
              n828 = local read "LC_l1_Cue1_First_OnOff"() -> (w1600:bool)
              n829 = local read "LC_l1_Cue1_All_OnOff"() -> (w1568:bool)
              n830 = call "myRIO_BRig_RT_dataLC_Selection_Block_NS_l1.vi"() -> ("output_Selection_Block_NS_l1"=w1561:i32)  [unwired: 11 in]
              n831 = call "myRIO_BRig_RT_dataLC_Selection_OnOff_NS_l1.vi"() -> ("output_Selection_OnOff_NS_l1"=w1560:i32)  [unwired: 11 in]
              n832 = call "myRIO_BRig_RT_dataLC_Selection_Probability_NS_l1.vi"() -> ("output_Selection_Probability_NS_l1"=w1559:i32)  [unwired: 11 in]
              n833 = call "myRIO_BRig_RT_dataLC_Selection_Tdelay_NS_l1.vi"() -> ("output_Selection_Tdelay_NS_l1"=w1558:i32)  [unwired: 11 in]
              n834 = call "myRIO_BRig_RT_dataLC_Selection_Count_NS_l1.vi"() -> ("output_Selection_Count_NS_l1"=w1551:i32)  [unwired: 11 in]
              n835 = local read "LC_l1_Cue1_All_delayOpt"() -> (w1569:bool)
              n836 = local read "LC_l1_Cue1_All_Probability"() -> (w1565:u16)
              n837 = local read "LC_l1_Cue1_All_Tdelay"() -> (w1564:u16)
              n838 = local read "LC_l1_Cue1_All_Count"() -> (w1563:u16)
              n839 = local read "LC_l1_Cue1_All_Block"() -> (w1567:u16)
              n840 = local read "LC_l1_Sel_All_Probability"() -> (w1553:u16)
              n841 = local read "LC_l1_Sel_All_Tdelay"() -> (w1552:u16)
              n842 = local read "LC_l1_Sel_All_OnOff"() -> (w1555:bool)
              n843 = local read "LC_l1_Sel_All_Count"() -> (w1550:u16)
              n844 = local read "LC_l1_Sel_All_Block"() -> (w1557:u16)
              n845 = Boolean To (0,1)(Boolean=w1579) -> (0, 1=w1581:i16)
              n846 = Boolean To (0,1)(Boolean=w1600) -> (0, 1=w1599:i16)
              n847 = Boolean To (0,1)(Boolean=w1568) -> (0, 1=w1571:i16)
              n848 = To Unsigned Word Integer(number=w1581) -> (unsigned 16bit integer=w1578:u16)
              n849 = To Unsigned Word Integer(number=w1599) -> (unsigned 16bit integer=w1598:u16)
              n850 = To Unsigned Word Integer(number=w1571) -> (unsigned 16bit integer=w1566:u16)
              n851 = Boolean To (0,1)(Boolean=w1569) -> (0, 1=w1570:i16)
              n852 = Boolean To (0,1)(Boolean=w1555) -> (0, 1=w1556:i16)
              n853 = To Unsigned Word Integer(number=w1570) -> (unsigned 16bit integer=w1562:u16)
              n854 = To Unsigned Word Integer(number=w1556) -> (unsigned 16bit integer=w1554:u16)
              n855 = Replace Array Subset(array=w1604, new element #1=w1602, index #1=w1603, new element #2=w1598, index #2=w1601, new element #3=w1596, index #3=w1597, new element #4=w1594, index #4=w1595, new element #5=w1592, index #5=w1593, new element #6=w1578, index #6=w1580, new element #7=w1567, index #7=w1577, new element #8=w1566, index #8=w1576, new element #9=w1565, index #9=w1575, new element #10=w1564, index #10=w1574, new element #11=w1563, index #11=w1573, new element #12=w1562, index #12=w1572, new element #13=w1557, index #13=w1561, new element #14=w1554, index #14=w1560, new element #15=w1553, index #15=w1559, new element #16=w1552, index #16=w1558, new element #17=w1550, index #17=w1551) -> (w1605:u16[])
            }
            frame 9 {
              # "Selection All"
              # "Count"
              # "Tdelay"
              # "Probability"
              # "OnOff"
              # "Block"
              # "delayOpt"
              # "Count"
              # "Tdelay"
              # "Probability"
              # "OnOff"
              # "Block"
              # "Cue1 All"
              # "delayOpt"
              # "Count"
              # "Tdelay"
              # "Probability"
              # "OnOff"
              # "Block"
              # "Cue1 First"
              n856 = call "myRIO_BRig_RT_dataLC_Cue1_delayOpt_Switch_l2.vi"() -> ("output_Cue1_delayOpt_Switch_l2"=w1644:i32)  [unwired: 11 in]
              n857 = call "myRIO_BRig_RT_dataLC_Cue1_Block_Switch_l2.vi"() -> ("output_Cue1_Block_Switch_l2"=w1667:i32)  [unwired: 11 in]
              n858 = call "myRIO_BRig_RT_dataLC_Cue1_OnOff_Switch_l2.vi"() -> ("output_Cue1_OnOff_Switch_l2"=w1665:i32)  [unwired: 11 in]
              n859 = call "myRIO_BRig_RT_dataLC_Cue1_Probability_Switch_l2.vi"() -> ("output_Cue1_l2_First_Probability"=w1661:i32)  [unwired: 11 in]
              n860 = call "myRIO_BRig_RT_dataLC_Cue1_Tdelay_Switch_l2.vi"() -> ("output_Cue1_Tdelay_Switch_l2"=w1659:i32)  [unwired: 11 in]
              n861 = call "myRIO_BRig_RT_dataLC_Cue1_Count_Switch_l2.vi"() -> ("output_Cue1_Count_Switch_l2"=w1657:i32)  [unwired: 11 in]
              n862 = call "myRIO_BRig_RT_dataLC_Cue1_Block_NS_l2.vi"() -> ("output_Cue1_Block_NS_l2"=w1641:i32)  [unwired: 11 in]
              n863 = call "myRIO_BRig_RT_dataLC_Cue1_OnOff_NS_l2.vi"() -> ("output_Cue1_OnOff_NS_l2"=w1640:i32)  [unwired: 11 in]
              n864 = call "myRIO_BRig_RT_dataLC_Cue1_Probability_NS_l2.vi"() -> ("output_Cue1_l2_All_Probability"=w1639:i32)  [unwired: 11 in]
              n865 = call "myRIO_BRig_RT_dataLC_Cue1_Tdelay_NS_l2.vi"() -> ("output_Cue1_Tdelay_NS_l2"=w1638:i32)  [unwired: 11 in]
              n866 = call "myRIO_BRig_RT_dataLC_Cue1_Count_NS_l2.vi"() -> ("output_Cue1_Count_NS_l2"=w1637:i32)  [unwired: 11 in]
              n867 = call "myRIO_BRig_RT_dataLC_Cue1_delayOpt_NS_l2.vi"() -> ("output_Cue1_delayOpt_NS_l2"=w1636:i32)  [unwired: 11 in]
              n868 = local read "LC_l2_Cue1_First_delayOpt"() -> (w1643:bool)
              n869 = local read "LC_l2_Cue1_First_Count"() -> (w1656:u16)
              n870 = local read "LC_l2_Cue1_First_Probability"() -> (w1660:u16)
              n871 = local read "LC_l2_Cue1_First_Block"() -> (w1666:u16)
              n872 = local read "LC_l2_Cue1_First_Tdelay"() -> (w1658:u16)
              n873 = local read "LC_l2_Cue1_First_OnOff"() -> (w1664:bool)
              n874 = local read "LC_l2_Cue1_All_OnOff"() -> (w1632:bool)
              n875 = call "myRIO_BRig_RT_dataLC_Selection_Block_NS_l1.vi"() -> ("output_Selection_Block_NS_l1"=w1625:i32)  [unwired: 11 in]
              n876 = call "myRIO_BRig_RT_dataLC_Selection_OnOff_NS_l1.vi"() -> ("output_Selection_OnOff_NS_l1"=w1624:i32)  [unwired: 11 in]
              n877 = call "myRIO_BRig_RT_dataLC_Selection_Probability_NS_l1.vi"() -> ("output_Selection_Probability_NS_l1"=w1623:i32)  [unwired: 11 in]
              n878 = call "myRIO_BRig_RT_dataLC_Selection_Tdelay_NS_l1.vi"() -> ("output_Selection_Tdelay_NS_l1"=w1622:i32)  [unwired: 11 in]
              n879 = call "myRIO_BRig_RT_dataLC_Selection_Count_NS_l1.vi"() -> ("output_Selection_Count_NS_l1"=w1615:i32)  [unwired: 11 in]
              n880 = local read "LC_l2_Cue1_All_delayOpt"() -> (w1633:bool)
              n881 = local read "LC_l2_Cue1_All_Probability"() -> (w1629:u16)
              n882 = local read "LC_l2_Cue1_All_Tdelay"() -> (w1628:u16)
              n883 = local read "LC_l2_Cue1_All_Count"() -> (w1627:u16)
              n884 = local read "LC_l2_Cue1_All_Block"() -> (w1631:u16)
              n885 = local read "LC_l1_Sel_All_Probability"() -> (w1617:u16)
              n886 = local read "LC_l1_Sel_All_Tdelay"() -> (w1616:u16)
              n887 = local read "LC_l1_Sel_All_OnOff"() -> (w1619:bool)
              n888 = local read "LC_l1_Sel_All_Count"() -> (w1614:u16)
              n889 = local read "LC_l1_Sel_All_Block"() -> (w1621:u16)
              n890 = Boolean To (0,1)(Boolean=w1643) -> (0, 1=w1645:i16)
              n891 = Boolean To (0,1)(Boolean=w1664) -> (0, 1=w1663:i16)
              n892 = Boolean To (0,1)(Boolean=w1632) -> (0, 1=w1635:i16)
              n893 = To Unsigned Word Integer(number=w1645) -> (unsigned 16bit integer=w1642:u16)
              n894 = To Unsigned Word Integer(number=w1663) -> (unsigned 16bit integer=w1662:u16)
              n895 = To Unsigned Word Integer(number=w1635) -> (unsigned 16bit integer=w1630:u16)
              n896 = Boolean To (0,1)(Boolean=w1633) -> (0, 1=w1634:i16)
              n897 = Boolean To (0,1)(Boolean=w1619) -> (0, 1=w1620:i16)
              n898 = To Unsigned Word Integer(number=w1634) -> (unsigned 16bit integer=w1626:u16)
              n899 = To Unsigned Word Integer(number=w1620) -> (unsigned 16bit integer=w1618:u16)
              n900 = Replace Array Subset(array=w1668, new element #1=w1666, index #1=w1667, new element #2=w1662, index #2=w1665, new element #3=w1660, index #3=w1661, new element #4=w1658, index #4=w1659, new element #5=w1656, index #5=w1657, new element #6=w1642, index #6=w1644, new element #7=w1631, index #7=w1641, new element #8=w1630, index #8=w1640, new element #9=w1629, index #9=w1639, new element #10=w1628, index #10=w1638, new element #11=w1627, index #11=w1637, new element #12=w1626, index #12=w1636, new element #13=w1621, index #13=w1625, new element #14=w1618, index #14=w1624, new element #15=w1617, index #15=w1623, new element #16=w1616, index #16=w1622, new element #17=w1614, index #17=w1615) -> (w1669:u16[])
            }
            frame 11 {
              # "Trial"
              # "Tdelay"
              # "Probability"
              # "OnOff"
              # "Block"
              # "Wrong"
              # "Trial"
              # "Tdelay"
              # "Probability"
              # "OnOff"
              # "Block"
              # "Reward"
              n901 = call "myRIO_BRig_RT_dataLC_Wrong_Block_l1.vi"() -> ("output_Wrong_Block_l1"=w1698:i32)  [unwired: 11 in]
              n902 = call "myRIO_BRig_RT_dataLC_Wrong_OnOff_l1.vi"() -> ("output_Wrong_OnOff_l1"=w1697:i32)  [unwired: 11 in]
              n903 = call "myRIO_BRig_RT_dataLC_Wrong_Probability_l1.vi"() -> ("output_Wrong_Probability_l1"=w1696:i32)  [unwired: 11 in]
              n904 = call "myRIO_BRig_RT_dataLC_Wrong_Tdelay_l1.vi"() -> ("output_Wrong_Tdelay_l1"=w1695:i32)  [unwired: 11 in]
              n905 = call "myRIO_BRig_RT_dataLC_Wrong_Trial_l1.vi"() -> ("output_Wrong_Trial_l1"=w1694:i32)  [unwired: 11 in]
              n906 = call "myRIO_BRig_RT_dataLC_Reward_Block_l1.vi"() -> ("output_Reward_Block_l1"=w1710:i32)  [unwired: 11 in]
              n907 = call "myRIO_BRig_RT_dataLC_Reward_OnOff_l1.vi"() -> ("output_Reward_OnOff_l1"=w1708:i32)  [unwired: 11 in]
              n908 = call "myRIO_BRig_RT_dataLC_Reward_Probability_l1.vi"() -> ("output_Reward_Probability_l1"=w1704:i32)  [unwired: 11 in]
              n909 = call "myRIO_BRig_RT_dataLC_Reward_Tdelay_l1.vi"() -> ("output_Reward_Tdelay_l1"=w1702:i32)  [unwired: 11 in]
              n910 = call "myRIO_BRig_RT_dataLC_Reward_Trial_l1.vi"() -> ("output_Reward_Trial_l1"=w1700:i32)  [unwired: 11 in]
              n911 = local read "LC_l1_Wrong_OnOff"() -> (w1692:bool)
              n912 = local read "LC_l1_Wrong_Probability"() -> (w1689:u16)
              n913 = local read "LC_l1_Wrong_Block"() -> (w1691:u16)
              n914 = local read "LC_l1_Wrong_Tdelay"() -> (w1688:u16)
              n915 = local read "LC_l1_Wrong_Trial"() -> (w1687:u16)
              n916 = local read "LC_l1_Reward_Probability"() -> (w1703:u16)
              n917 = local read "LC_l1_Reward_Block"() -> (w1709:u16)
              n918 = local read "LC_l1_Reward_Tdelay"() -> (w1701:u16)
              n919 = local read "LC_l1_Reward_OnOff"() -> (w1707:bool)
              n920 = local read "LC_l1_Reward_Trial"() -> (w1699:u16)
              n921 = Boolean To (0,1)(Boolean=w1692) -> (0, 1=w1693:i16)
              n922 = Boolean To (0,1)(Boolean=w1707) -> (0, 1=w1706:i16)
              n923 = To Unsigned Word Integer(number=w1693) -> (unsigned 16bit integer=w1690:u16)
              n924 = To Unsigned Word Integer(number=w1706) -> (unsigned 16bit integer=w1705:u16)
              n925 = Replace Array Subset(array=w1711, new element #1=w1709, index #1=w1710, new element #2=w1705, index #2=w1708, new element #3=w1703, index #3=w1704, new element #4=w1701, index #4=w1702, new element #5=w1699, index #5=w1700, new element #6=w1691, index #6=w1698, new element #7=w1690, index #7=w1697, new element #8=w1689, index #8=w1696, new element #9=w1688, index #9=w1695, new element #10=w1687, index #10=w1694) -> (w1712:u16[])
            }
            frame 12 {
              # "Trial"
              # "Tdelay"
              # "Probability"
              # "OnOff"
              # "Block"
              # "Wrong"
              # "Trial"
              # "Tdelay"
              # "Probability"
              # "OnOff"
              # "Block"
              # "Reward"
              n926 = call "myRIO_BRig_RT_dataLC_Wrong_Block_l1.vi"() -> ("output_Wrong_Block_l1"=w1742:i32)  [unwired: 11 in]
              n927 = call "myRIO_BRig_RT_dataLC_Wrong_OnOff_l1.vi"() -> ("output_Wrong_OnOff_l1"=w1741:i32)  [unwired: 11 in]
              n928 = call "myRIO_BRig_RT_dataLC_Wrong_Probability_l1.vi"() -> ("output_Wrong_Probability_l1"=w1740:i32)  [unwired: 11 in]
              n929 = call "myRIO_BRig_RT_dataLC_Wrong_Tdelay_l1.vi"() -> ("output_Wrong_Tdelay_l1"=w1739:i32)  [unwired: 11 in]
              n930 = call "myRIO_BRig_RT_dataLC_Wrong_Trial_l1.vi"() -> ("output_Wrong_Trial_l1"=w1738:i32)  [unwired: 11 in]
              n931 = call "myRIO_BRig_RT_dataLC_Reward_Block_l1.vi"() -> ("output_Reward_Block_l1"=w1754:i32)  [unwired: 11 in]
              n932 = call "myRIO_BRig_RT_dataLC_Reward_OnOff_l1.vi"() -> ("output_Reward_OnOff_l1"=w1752:i32)  [unwired: 11 in]
              n933 = call "myRIO_BRig_RT_dataLC_Reward_Probability_l1.vi"() -> ("output_Reward_Probability_l1"=w1748:i32)  [unwired: 11 in]
              n934 = call "myRIO_BRig_RT_dataLC_Reward_Tdelay_l1.vi"() -> ("output_Reward_Tdelay_l1"=w1746:i32)  [unwired: 11 in]
              n935 = call "myRIO_BRig_RT_dataLC_Reward_Trial_l1.vi"() -> ("output_Reward_Trial_l1"=w1744:i32)  [unwired: 11 in]
              n936 = local read "LC_l1_Wrong_OnOff"() -> (w1736:bool)
              n937 = local read "LC_l1_Wrong_Probability"() -> (w1733:u16)
              n938 = local read "LC_l1_Wrong_Block"() -> (w1735:u16)
              n939 = local read "LC_l1_Wrong_Tdelay"() -> (w1732:u16)
              n940 = local read "LC_l1_Wrong_Trial"() -> (w1731:u16)
              n941 = local read "LC_l1_Reward_Probability"() -> (w1747:u16)
              n942 = local read "LC_l1_Reward_Block"() -> (w1753:u16)
              n943 = local read "LC_l1_Reward_Tdelay"() -> (w1745:u16)
              n944 = local read "LC_l1_Reward_OnOff"() -> (w1751:bool)
              n945 = local read "LC_l1_Reward_Trial"() -> (w1743:u16)
              n946 = Boolean To (0,1)(Boolean=w1736) -> (0, 1=w1737:i16)
              n947 = Boolean To (0,1)(Boolean=w1751) -> (0, 1=w1750:i16)
              n948 = To Unsigned Word Integer(number=w1737) -> (unsigned 16bit integer=w1734:u16)
              n949 = To Unsigned Word Integer(number=w1750) -> (unsigned 16bit integer=w1749:u16)
              n950 = Replace Array Subset(array=w1755, new element #1=w1753, index #1=w1754, new element #2=w1749, index #2=w1752, new element #3=w1747, index #3=w1748, new element #4=w1745, index #4=w1746, new element #5=w1743, index #5=w1744, new element #6=w1735, index #6=w1742, new element #7=w1734, index #7=w1741, new element #8=w1733, index #8=w1740, new element #9=w1732, index #9=w1739, new element #10=w1731, index #10=w1738) -> (w1756:u16[])
            }
            frame 13 {
              # "amp_L"
              # "amp_R"
              # "freq_L"
              # "freq_R"
              n951 = call "myRIO_BRig_RT_dataExp_Audio_amp__L.vi"() -> ("output_Audio_amp__L"=w1781:i32)  [unwired: 11 in]
              n952 = call "myRIO_BRig_RT_dataExp_Audio_amp__R.vi"() -> ("output_Audio_amp__R"=w1780:i32)  [unwired: 11 in]
              n953 = call "myRIO_BRig_RT_dataExp_Audio_freq__L.vi"() -> ("output_Audio_freq__L"=w1779:i32)  [unwired: 11 in]
              n954 = call "myRIO_BRig_RT_dataExp_Audio_freq__R.vi"() -> ("output_Audio_freq__R"=w1778:i32)  [unwired: 11 in]
              n955 = Index Array(array=w1777, index #1=w1781, index #2=w1780, index #3=w1779, index #4=w1778) -> (element #1=w1776:u16, element #2=w1775:u16, element #3=w1768:u16, element #4=w1766:u16)
              n956 = To Unsigned Byte Integer(number=w1768) -> (unsigned 8bit integer=w1767:u8)
              n957 = To Unsigned Byte Integer(number=w1766) -> (unsigned 8bit integer=w1765:u8)
            }
            frame 14 {
              w1790 = u32 0 ("laser2_selRew_Ndelay")
              # "tDelay"
              # "Wrong l1"
              # "Reward l1"
              n958 = local read "laser1_Tpeak"() -> (w1805:dbl)
              n959 = local read "laser1_Freq"() -> (w1804:dbl)
              n960 = local read "laser1_Tshutter"() -> (w1803:dbl)
              n961 = local read "laser1_duration"() -> (w1800:u16)
              n962 = local read "laser2_Tpeak"() -> (w1798:dbl)
              n963 = local read "laser2_Freq"() -> (w1797:dbl)
              n964 = local read "laser2_Tshutter"() -> (w1796:dbl)
              n965 = local read "laser2_duration"() -> (w1795:u16)
              n966 = call "myRIO_BRig_RT_dataLC_Reward_Tdelay_l1.vi"() -> ("output_Reward_Tdelay_l1"=w1821:i32)  [unwired: 11 in]
              n967 = call "myRIO_BRig_RT_dataLC_Wrong_Tdelay_l1.vi"() -> ("output_Wrong_Tdelay_l1"=w1822:i32)  [unwired: 11 in]
              n968 = local read "FPGA_count2ms"() -> (w1799:dbl)
              n969 = Index Array(array=w1818, index #1=w1821, index #2=w1822) -> (element #1=w1820:u16, element #2=w1819:u16)
              n970 = To Double Precision Float(number=w1820) -> (double precision float=w1815:dbl)
              n971 = To Double Precision Float(number=w1819) -> (double precision float=w1812:dbl)
              n972 = To Unsigned Word Integer(number=w1799) -> (unsigned 16bit integer=w1809:u16)
              n973 = call "myRIO_BRig_RT__calc_laser_FPGA_N.vi"("input_FPGA_count2ms"=w1799, "input_Tpeak"=w1805, "input_Freq"=w1804, "input_Tshutter"=w1803, "input_duration"=w1800) -> ("output_laser_Npeak"=w1808:u32, "output_laser_Nvalley"=w1807:u32, "output_laser_Nshutter"=w1806:u32, "output_laser_Nduration"=w1802:u32, "output_laser_Tduration"=w1801:u16)  [unwired: 6 in]
              n974 = Multiply(x=w1799, y=w1815) -> (x*y=w1816:dbl)
              n975 = Multiply(x=w1799, y=w1812) -> (x*y=w1813:dbl)
              n976 = call "myRIO_BRig_RT__calc_laser_FPGA_N.vi"("input_FPGA_count2ms"=w1799, "input_Tpeak"=w1798, "input_Freq"=w1797, "input_Tshutter"=w1796, "input_duration"=w1795) -> ("output_laser_Npeak"=w1794:u32, "output_laser_Nvalley"=w1793:u32, "output_laser_Nshutter"=w1792:u32, "output_laser_Nduration"=w1791:u32)  [unwired: 6 in, 1 out]
              n977 = Round Toward +Infinity(x=w1816) -> (ceil(x): smallest int >= x=w1817:dbl)
              n978 = Round Toward +Infinity(x=w1813) -> (ceil(x): smallest int >= x=w1814:dbl)
              n979 = To Unsigned Long Integer(number=w1817) -> (unsigned 32bit integer=w1811:u32)
              n980 = To Unsigned Long Integer(number=w1814) -> (unsigned 32bit integer=w1810:u32)
              n981 = xnode "Read/Write Control"("FPGA VI Reference In"=w1825, "error in"=w1826, "laser1_Npeak"=w1808, "laser1_Nvalley"=w1807, "laser1_Nshutter"=w1806, "laser1_selRew_Ndelay"=w1811, "laser1_selWro_Ndelay"=w1810, "laser1_selRew_Ntotal"=w1802, "laser1_selWro_Ntotal"=w1802, "k1__counter_per_ms"=w1809, "laser2_Npeak"=w1794, "laser2_Nvalley"=w1793, "laser2_Nshutter"=w1792, "laser2_selRew_Ndelay"=w1790, "laser2_selWro_Ndelay"=w1790, "laser2_selRew_Ntotal"=w1791, "laser2selWro_Ntotal"=w1791) -> ("error out"=→"error out":errorcluster)  [unwired: 1 out]
              n982 = call "myRIO_BRig_RT_dataCurrent_laser1_pulse_duration.vi"() -> ("output_laser1_pulse_duration"=w1823:i32)  [unwired: 11 in]
              n983 = Replace Array Subset(array=w1818, new element=w1801, index=w1823) -> (w1824:u16[])
            }
            frame 16 {
              n984 = call "myRIO_Brig_RT__Case_Exp_State_initBlock.vi"("input_spout"=w1870, "input_dataExp"=w1868, "input_dataCurrent"=w1869) -> ("output_spout"=w1848:enum16{"Left", "Right"}, "output_state"=w1871:T2, "output_dataExp"=w1867:u16[], "output_dataCurrent"=w1853:u16[], "output_TpB_target"=→"TpB_target":u16)  [unwired: 4 in]
              "cSpout" <- w1848
              n985 = call "myRIO_BRig_RT_dataCurrent_iBlock.vi"() -> ("output_iBlock"=w1852:i32)  [unwired: 11 in]
              n986 = Index Array(array=w1853, index=w1852) -> (element=w1846:u16)
              "iBlock" <- w1846
            }
            frame 17 {
              n987 = local write "nRewards_cur"(u16 0 ("nRewards_cur")) -> ()
              n988 = call "myRIO_BRig_RT__Case_Exp_State_initBlock2.vi"("input_spout"=w1879, "input_dataBlock"=w1880, "input_dataCurrent"=w1878) -> ("idxDataBlock"=w1875:i32, "output_dataBlock"=w1877:u16[][])  [unwired: 7 in]
            }
            frame 20 {
              n989 = call "myRIO_Brig_RT__Case_Exp_State_initTrial.vi"("input_spout"=w1898, "input_dataExp"=w1914, "input_dataCurrent"=w1915) -> ("output_state"=w1916:T2, "output_dataExp"=w1913:u16[], "output_dataCurrent"=w1903:u16[])  [unwired: 6 in]
              n990 = call "myRIO_BRig_RT_dataCurrent_iTrial.vi"() -> ("output_iTrial"=w1902:i32)  [unwired: 11 in]
              n991 = call "myRIO_BRig_RT_dataCurrent_SolenoidReward.vi"() -> ("output_SolenoidReward"=w1897:i32)  [unwired: 11 in]
              n992 = Index Array(array=w1903, index #1=w1902, index #2=w1897) -> (element #1=w1893:u16, element #2=w1896:u16)
              "iTrial" <- w1893
              n993 = Not Equal To 0?(x=w1896) -> (x != 0?=→"SolenoidReward":bool)
            }
            frame 21 {
              # "trialUntilReward"
              n994 = call "myRIO_BRig_RT__Case_Exp_subState_LC__initTrial.vi"("input_dataTrial"=w1923, "input_spout"=w1932, "input_dataCurrent"=w1921, "input_dataLC"=w1920) -> ("output_LC_Wrong"=w1933:bool, "output_LC_led_Wrong"=w1925:bool, "output_LC_Reward"=w1934:bool, "output_LC_led_Reward"=w1924:bool, "output_dataTrial"=w1922:u16[][])  [unwired: 2 in]
              n995 = Equal?(x=w1932, y=enum16{"Left", "Right"}."Right") -> (x = y?=w1930:bool)
              n996 = call "myRIO_BRig_RT_dataExp_ItrialUntilReward.vi"() -> ("output_I_trialUntilReward"=w1928:i32)  [unwired: 11 in]
              n997 = Index Array(array=w1929, index=w1928) -> (element=w1927:u16)
              n998 = Not Equal To 0?(x=w1927) -> (x != 0?=w1926:bool)
              n999 = xnode "Read/Write Control"("FPGA VI Reference In"=w1947, "error in"=w1946, "SelectionState"=FALSE, "laserResponse_reward"=w1934, "laserResponse_wrong"=w1933, "laserResponse_reward_LED"=w1924, "laserResponse_wrong_LED"=w1925, "Left(F)_or_Right(T)"=w1930, "ignoreWrong"=w1926) -> ("error out"=→"error_initTrial":errorcluster)  [unwired: 1 out]
            }
            frame 22 {
              n1000 = call "myRIO_BRig_RT_arrTrig_init.vi"() -> ("output_arrTrig"=w1953:bool[])  [unwired: 11 in]
              n1001 = call "myRIO_BRig_RT__Case_Exp_State_initTrial_dataTrial.vi"("input_spout"=w1963, "input_dataCurrent"=w1964, "input_dataExp"=w1962, "input_dataTrial"=w1966) -> ("output_dataTrial"=w1965:u16[][], "output_laserPower_l1"=w1959:u16)  [unwired: 5 in, 1 out]
              n1002 = To Double Precision Float(number=w1959) -> (double precision float=w1961:dbl)
              n1003 = Divide(x=w1961, y=100.0 ("x")) -> (x/y=w1955:dbl)
              "output_PortA" <- w1955
              n1004 = call "myRIO__convert__Voltage_to_FPGAvalue.vi"("input_voltage"=w1955) -> ("output_PortC"=w1954:i16)  [unwired: 9 in, 1 out]
              n1005 = xnode "Read/Write Control"("FPGA VI Reference In"=w1958, "error in"=w1957, "AnaOut_0"=w1954) -> ("error out"=→"error out 4":errorcluster)  [unwired: 1 out]
            }
            frame 23 {
              n1006 = call "myRIO_BRig_RT_dataCurrent_idxDataTrial.vi"() -> ("output_idxDataTrial"=w1992:i32)  [unwired: 11 in]
              n1007 = call "myRIO_BRig_RT_dataTrial_activeRecording.vi"() -> ("output_activeRecording"=w1989:i32)  [unwired: 11 in]
              n1008 = Index Array(array=w1994, index=w1992) -> (element=w1991:u16)
              n1009 = Boolean To (0,1)(Boolean="Recording") -> (0, 1=w1988:i16)
              n1010 = To Long Integer(number=w1991) -> (32bit integer=w1990:i32)
              n1011 = To Unsigned Word Integer(number=w1988) -> (unsigned 16bit integer=w1987:u16)
              n1012 = Replace Array Subset(array=w1993, new element=w1987, index (row)=w1990, index (col)=w1989) -> (w1986:u16[][])
            }
            frame 24 {
              n1013 = call "myRIO_BRig_RT__Case_Exp_State_initTrial_LC_ENL1__v2.vi"("input_dataTrial"=w2019, "input_spout"=w2024, "input_dataBlock"=w2017, "input_dataLC"=w2025, "input_dataCurrent"=w2021) -> ("output_LC__ENL1"=w2023:bool, "output_LC_led__ENL1"=w2022:bool, "output_dataTrial"=w2018:u16[][], "output_dataCurrent"=w2020:u16[])  [unwired: 3 in]
            }
            frame 25 {
              w2042 = TRUE ("Recording")
              n1014 = call "myRIO_BRig_RT__Case_Exp_State_initTrial_LC_Cue1__v3.vi"("input_dataTrial"=w2047, "input_spout"=w2050, "input_arrTrig"=w2041, "input_dataBlock"=w2045, "input_dataLC"=w2051, "input_dataCurrent"=w2049) -> ("output_arrTrig"=w2040:bool[], "output_dataTrial"=w2046:u16[][], "output_dataCurrent"=w2048:u16[])  [unwired: 3 in]
            }
            frame 27 {
              n1015 = call "myRIO_BRig_RT__Case_Exp_State_initTrial_LC_Sel__v2.vi"("input_dataTrial"=w2077, "input_spout"=w2080, "input_dataBlock"=w2075, "input_dataLC"=w2081, "input_dataCurrent"=w2079) -> ("output_LC__Sel"=w2067:bool, "output_LC_led__Sel"=w2068:bool, "output_dataTrial"=w2076:u16[][], "output_dataCurrent"=w2078:u16[])  [unwired: 3 in]
              n1016 = local read "Recording"() -> (w2072:bool)
            }
            frame 29 {
              # "ENL1_n"
              # "Tcycle"
              # "counter"
              n1017 = call "myRIO_BRig_RT_dataCurrent_Tcycle_generic.vi"() -> ("output_Tcycle_generic"=w2128:i32)  [unwired: 11 in]
              n1018 = call "myRIO_BRig_RT_dataCurrent_count_generic.vi"() -> ("output_count_generic"=w2130:i32)  [unwired: 11 in]
              n1019 = call "myRIO_BRig_RT_dataCurrent_Tcycle_ENL.vi"() -> ("output_ENL"=w2127:i32)  [unwired: 11 in]
              n1020 = call "myRIO_BRig_RT_dataCurrent_nENL1.vi"() -> ("output_nENL1"=w2101:i32)  [unwired: 11 in]
              n1021 = Index Array(array=w2121, index #1=w2127, index #2=w2101) -> (element #1=w2126:u16, element #2=w2100:u16)
              n1022 = Increment(x=w2100) -> (x+1=w2099:u16)
              n1023 = Replace Array Subset(array=w2121, new element #1=u16 0 ("new element/subarray"), index #1=w2130, new element #2=w2126, index #2=w2128, new element #3=w2099, index #3=w2101) -> (w2125:u16[])
              n1024 = Select(t=myRIO_BRig_RT__Case_Exp_stateList."ENL1Penalty_pre" ("Enum"), s=w2109, f=myRIO_BRig_RT__Case_Exp_stateList."ENL1" ("Enum")) -> (s? t:f=w2106:T2)
            }
            frame 30 {
              n1025 = call "myRIO_BRig_RT__Case_Exp_State_ENL1__v2.vi"("input_LC"=w2138, "I_lick"=w2141, "input_LC_led"=w2139, "input_state"=w2147, "input_dataCurrent"=w2146) -> ("output_trigger_laser_led"=w2137:bool, "output_state"=w2144:T2, "output_dataCurrent"=w2145:u16[], "output_trigger_laser"=w2136:bool)  [unwired: 3 in]
            }
            frame 32 {
              # "Tcycle"
              # "counter"
              n1026 = call "myRIO_BRig_RT_dataCurrent_Tcycle_generic.vi"() -> ("output_Tcycle_generic"=w2188:i32)  [unwired: 11 in]
              n1027 = call "myRIO_BRig_RT_dataCurrent_count_generic.vi"() -> ("output_count_generic"=w2190:i32)  [unwired: 11 in]
              n1028 = call "myRIO_BRig_RT_dataExp_ENL_penalty.vi"() -> ("output_ENL_penalty"=w2183:i32)  [unwired: 11 in]
              n1029 = Index Array(array=w2184, index=w2183) -> (element=w2187:u16)
              n1030 = Replace Array Subset(array=w2185, new element #1=u16 0 ("new element/subarray"), index #1=w2190, new element #2=w2187, index #2=w2188) -> (w2186:u16[])
            }
            frame 33 {
              n1031 = call "myRIO_BRig_RT__Case_Exp_State_ENL1Penalty.vi"("input_state"=w2214, "input_dataCurrent"=w2218) -> ("output_state"=w2215:T2, "output_dataCurrent"=w2217:u16[])  [unwired: 8 in]
            }
            frame 34 {
            }
            frame 35 {
            }
            frame 36 {
            }
            frame 37 {
            }
            frame 38 {
              # "Cue1_n"
              # "Tcycle_Cue1"
              # "0 = L, 1 = R, 2 = both"
              # "sp_R"
              # "sp_L"
              # "Tcycle"
              # "counter"
              n1032 = Equal?(x=w2330, y=enum16{"Left", "Right"}."Left") -> (x = y?=w2329:bool)
              n1033 = call "myRIO_BRig_RT_dataExp_Audio_sp__L.vi"() -> ("output_Audio_sp__L"=w2328:i32)  [unwired: 11 in]
              n1034 = call "myRIO_BRig_RT_dataExp_Audio_sp__R.vi"() -> ("output_Audio_sp__R"=w2327:i32)  [unwired: 11 in]
              n1035 = call "myRIO_BRig_RT_dataCurrent_Tcycle_generic.vi"() -> ("output_Tcycle_generic"=w2340:i32)  [unwired: 11 in]
              n1036 = call "myRIO_BRig_RT_dataCurrent_count_generic.vi"() -> ("output_count_generic"=w2342:i32)  [unwired: 11 in]
              n1037 = Select(t=w2328, s=w2329, f=w2327) -> (s? t:f=w2326:i32)
              n1038 = call "myRIO_BRig_RT_dataCurrent_nCue1.vi"() -> ("output_nCue1"=w2304:i32)  [unwired: 11 in]
              n1039 = call "myRIO_BRig_RT_dataCurrent_Tcycle_cue.vi"() -> ("output_Tcycle_cue"=w2313:i32)  [unwired: 11 in]
              n1040 = Index Array(array=w2332, index=w2326) -> (element=w2324:u16)
              n1041 = Index Array(array=w2314, index #1=w2313, index #2=w2304) -> (element #1=w2315:u16, element #2=w2306:u16)
              n1042 = Increment(x=w2306) -> (x+1=w2305:u16)
              n1043 = Not Equal To 0?(x=w2324) -> (x != 0?=w2322:bool)
              n1044 = Not Equal?(x=w2324, y=u16 1) -> (x != y?=w2323:bool)
              n1045 = Replace Array Subset(array=w2314, new element #1=u16 0 ("new element/subarray"), index #1=w2342, new element #2=w2315, index #2=w2340, new element #3=w2305, index #3=w2304) -> (w2339:u16[])
              n1046 = Select(t=myRIO_BRig_RT__Case_Exp_stateList."Cue1Penalty_pre" ("Enum"), s=w2310, f=myRIO_BRig_RT__Case_Exp_stateList."Cue1" ("Enum")) -> (s? t:f=w2311:T2)
            }
            frame 39 {
              n1047 = call "myRIO_BRig_RT__Case_Exp_State_Cue1__v3.vi"("I_lick"=w2357, "input_arrTrig"=w2349, "input_state"=w2359, "input_dataCurrent"=w2377) -> ("output_l1_laserOn"=w2347:bool, "output_l1_laserEvent"=w2348:bool, "output_state"=w2358:T2, "output_dataCurrent"=w2376:u16[], "output_l2_laserEvent"=w2346:bool, "output_l2_laserOn"=w2345:bool)  [unwired: 1 in, 1 out]
              n1048 = Equal?(x=myRIO_BRig_RT__Case_Exp_stateList."Selection_pre", y=w2358) -> (x = y?=w2362:bool)
              n1049 = xnode "Read/Write Control"("FPGA VI Reference In"=w2361, "error in"=w2360, "SelectionState"=w2362) -> ()  [unwired: 2 out]
            }
            frame 41 {
              # "Tcycle"
              # "counter"
              n1050 = call "myRIO_BRig_RT_dataCurrent_Tcycle_generic.vi"() -> ("output_Tcycle_generic"=w2408:i32)  [unwired: 11 in]
              n1051 = call "myRIO_BRig_RT_dataCurrent_count_generic.vi"() -> ("output_count_generic"=w2410:i32)  [unwired: 11 in]
              n1052 = call "myRIO_BRig_RT_dataExp_Tcycle_CuePenalty.vi"() -> ("output_Tcycle_CuePenalty"=w2407:i32)  [unwired: 11 in]
              n1053 = Index Array(array=w2402, index=w2407) -> (element=w2406:u16)
              n1054 = Replace Array Subset(array=w2404, new element #1=u16 0 ("new element/subarray"), index #1=w2410, new element #2=w2406, index #2=w2408) -> (w2403:u16[])
            }
            frame 42 {
              # "reset laserOccurred"
              n1055 = call "myRIO_BRig_RT__Case_Exp_State_Cue1Penalty.vi"("input_state"=w2436, "input_dataCurrent"=w2437) -> ("output_state"=w2434:T2, "output_dataCurrent"=w2435:u16[])  [unwired: 8 in]
            }
            frame 43 {
              n1056 = call "myRIO_BRig_RT__Case_Exp_subState_LC__Cue2.vi"("input_spout"=w2454, "input_dataCurrent"=w2455, "input_dataLC"=w2453) -> ()  [unwired: 6 in, 2 out]
            }
            frame 44 {
            }
            frame 45 {
            }
            frame 46 {
            }
            frame 47 {
              # "Tcycle"
              # "counter"
              n1057 = call "myRIO_BRig_RT_dataCurrent_laser1_tSel_start.vi"() -> ("output_laser1_tSel_start"=w2525:i32)  [unwired: 11 in]
              n1058 = xnode "Read/Write Control"("FPGA VI Reference In"=w2535, "error in"=w2536) -> ("error out"=→"error_Selection_pre":errorcluster, "SelectReward"=w2529:bool, "SelectWrong"=w2530:bool)  [unwired: 1 out]
              n1059 = call "myRIO_BRig_RT_dataExp_Tcycle_Selection.vi"() -> ("output_Tcycle_Selection"=w2555:i32)  [unwired: 11 in]
              n1060 = call "myRIO_BRig_RT_dataCurrent_Tcycle_generic.vi"() -> ("output_Tcycle_generic"=w2556:i32)  [unwired: 11 in]
              n1061 = call "myRIO_BRig_RT_dataCurrent_count_generic.vi"() -> ("output_count_generic"=w2558:i32)  [unwired: 11 in]
              n1062 = Index Array(array=w2526, index=w2525) -> (element=w2524:u16)
              n1063 = Index Array(array=w2552, index=w2555) -> (element=w2554:u16)
              n1064 = Equal To 0?(x=w2524) -> (x = 0?=w2522:bool)
              n1065 = Replace Array Subset(array=w2526, new element #1=u16 0 ("new element/subarray"), index #1=w2558, new element #2=w2554, index #2=w2556) -> (w2553:u16[])
              n1066 = Or(x=w2529, y=w2530) -> (x .or. y?=w2520:bool)
              n1067 = Not(x=w2520) -> (.not. x?=w2523:bool)
              n1068 = Compound Arithmetic op=AND(w2523, w2522, w2521) -> (w2518:bool)
              n1069 = And(x=w2518, y=w2519) -> (x .and. y?=w2517:bool)
              n1070 = Select(t=myRIO_BRig_RT__Case_Exp_stateList."SelectReward_pre" ("Enum"), s=w2529, f=myRIO_BRig_RT__Case_Exp_stateList."SelectWrong_pre" ("Enum")) -> (s? t:f=w2534:T2)
              n1071 = Select(t=w2534, s=w2520, f=myRIO_BRig_RT__Case_Exp_stateList."Selection" ("Enum")) -> (s? t:f=w2531:T2)
            }
            frame 48 {
              # "counter\nSelection"
              # "increment"
              # "get Tcycle"
              # "get count"
              n1072 = call "myRIO_BRig_RT_dataCurrent_Tcycle_generic.vi"() -> ("output_Tcycle_generic"=w2592:i32)  [unwired: 11 in]
              n1073 = call "myRIO_BRig_RT_dataCurrent_count_generic.vi"() -> ("output_count_generic"=w2588:i32)  [unwired: 11 in]
              n1074 = call "myRIO_BRig_RT_dataCurrent_laser1_tSel_start.vi"() -> ("output_laser1_tSel_start"=w2580:i32)  [unwired: 11 in]
              n1075 = call "myRIO_BRig_RT_dataCurrent_laser1_tSel_end.vi"() -> ("output_laser1_tSel_end"=w2579:i32)  [unwired: 11 in]
              n1076 = call "myRIO_BRig_RT__increment_u16.vi"() -> ("output_increment__u16"=w2566:u16)  [unwired: 11 in]
              n1077 = xnode "Read/Write Control"("FPGA VI Reference In"=w2599, "error in"=w2598) -> ("error out"=→"error_Selection":errorcluster, "SelectReward"=w2595:bool, "SelectWrong"=w2596:bool)  [unwired: 1 out]
              n1078 = call "myRIO_BRig_RT_dataCurrent_laser1_triggered_Sel.vi"() -> ("output_laser1_triggered_Selection"=w2567:i32)  [unwired: 11 in]
              n1079 = Index Array(array=w2593, index #1=w2592, index #2=w2588, index #3=w2580, index #4=w2579, index #5=w2567) -> (element #1=w2587:u16, element #2=w2565:u16, element #3=w2564:u16, element #4=w2570:u16, element #5=w2561:u16)
              n1080 = Increment(x=w2561) -> (x+1=w2562:u16)
              n1081 = Equal?(x=w2565, y=w2564) -> (x = y?=w2563:bool)
              n1082 = Add(x=w2565, y=w2566) -> (x+y=w2571:u16)
              n1083 = Greater Or Equal?(x=w2571, y=w2564) -> (x >= y?=w2568:bool)
              n1084 = Less Or Equal?(x=w2571, y=w2570) -> (x <= y?=w2569:bool)
              n1085 = Greater?(x=w2587, y=w2571) -> (0:w2573:bool)
              n1086 = Select(t=w2562, s=w2563, f=w2561) -> (s? t:f=w2560:u16)
              n1087 = Select(t=myRIO_BRig_RT__Case_Exp_stateList."SelectReward_pre" ("Enum"), s=w2595, f=myRIO_BRig_RT__Case_Exp_stateList."SelectWrong_pre" ("Enum")) -> (s? t:f=w2594:T2)
              n1088 = Or(x=w2595, y=w2596) -> (x .or. y?=w2574:bool)
              n1089 = Not(x=w2574) -> (.not. x?=w2575:bool)
              n1090 = Select(t=w2591, s=w2573, f=myRIO_BRig_RT__Case_Exp_stateList."SelectTimeout_pre" ("Enum")) -> (s? t:f=w2582:u16)
              n1091 = Compound Arithmetic op=AND(w2573, w2575, w2568, w2569, w2572) -> (w2577:bool)
              n1092 = Select(t=w2571, s=w2573, f=w2587) -> (s? t:f=w2585:u16)
              n1093 = Select(t=w2594, s=w2574, f=w2582) -> (s? t:f=w2597:u16)
              n1094 = And(x=w2577, y=w2576) -> (x .and. y?=w2578:bool)
              n1095 = call "myRIO_BRig_RT_dataCurrent_count_selection.vi"() -> ("output_count_generic"=w2586:i32)  [unwired: 11 in]
              n1096 = Replace Array Subset(array=w2593, new element #1=w2585, index #1=w2588, new element #2=w2585, index #2=w2586, new element #3=w2560, index #3=w2567) -> (w2590:u16[])
            }
            frame 50 {
              # "iState"
              # "Tcycle\nReward"
              # "nRewTrials"
              # "Tcycle\nGeneric"
              # "counter"
              n1097 = call "myRIO_BRig_RT_dataCurrent_nRewTrials.vi"() -> ("output_nRewTrials"=w2631:i32)  [unwired: 11 in]
              n1098 = Equal?(x=w2640, y=enum16{"Left", "Right"}."Left") -> (x = y?=w2641:bool)
              n1099 = Index Array(array=w2632, index=w2631) -> (element=w2630:u16)
              n1100 = call "myRIO_BRig_RT_dataExp_Tcycle_Reward__L.vi"() -> ("output_Tcycle_Reward__L"=w2644:i32)  [unwired: 11 in]
              n1101 = call "myRIO_BRig_RT_dataExp_Tcycle_Reward__R.vi"() -> ("output_Tcycle_Reward__R"=w2645:i32)  [unwired: 11 in]
              n1102 = Increment(x=w2630) -> (x+1=w2629:u16)
              n1103 = Select(t=w2644, s=w2641, f=w2645) -> (s? t:f=w2643:i32)
              n1104 = call "myRIO_BRig_RT__Case_Exp_subState_LC__Reward.vi"("input_spout"=w2640, "input_dataCurrent"=w2632, "input_dataLC"=w2639) -> ()  [unwired: 6 in, 2 out]
              n1105 = call "myRIO_BRig_RT_dataCurrent_count_generic.vi"() -> ("output_count_generic"=w2634:i32)  [unwired: 11 in]
              n1106 = call "myRIO_BRig_RT_dataCurrent_Tcycle_generic.vi"() -> ("output_Tcycle_generic"=w2635:i32)  [unwired: 11 in]
              n1107 = Index Array(array=w2646, index=w2643) -> (element=w2636:u16)
              n1108 = call "myRIO_BRig_RT_dataCurrent_iState.vi"() -> ("output_iState"=w2624:i32)  [unwired: 11 in]
              n1109 = Replace Array Subset(array=w2632, new element #1=w2629, index #1=w2631, new element #2=u16 0 ("new element/subarray"), index #2=w2634, new element #3=w2636, index #3=w2635, new element #4=u16 1 ("new element/subarray"), index #4=w2624) -> (w2647:u16[])
            }
            frame 51 {
              n1110 = call "myRIO_BRig_RT__Case_Exp_State_Reward.vi"("input_dataCurrent"=w2668, "input_state"=w2665, "input_spout"=w2663) -> ("output_dataCurrent"=w2667:u16[], "output_state"=w2666:T2, "output__L"=w2661:bool, "output__R"=w2662:bool)  [unwired: 9 in]
            }
            frame 52 {
              # "nRewards"
              # "nRewTrials"
              # "Tcycle"
              # "counter"
              n1111 = call "myRIO_BRig_RT_dataBlock_nRewards__L.vi"() -> ("output_nRewards__L"=w2684:i32)  [unwired: 11 in]
              n1112 = call "myRIO_BRig_RT_dataBlock_nRewards__R.vi"() -> ("output_nRewards__R"=w2683:i32)  [unwired: 11 in]
              n1113 = call "myRIO_BRig_RT_dataCurrent_Tcycle_generic.vi"() -> ("output_Tcycle_generic"=w2703:i32)  [unwired: 11 in]
              n1114 = call "myRIO_BRig_RT_dataCurrent_count_generic.vi"() -> ("output_count_generic"=w2705:i32)  [unwired: 11 in]
              n1115 = case shown="\"Left\", Default" w2677 {
                tunnel: w2689 -> [w2710 w2714]
                tunnel: [w2709 w2714] -> w2688
                tunnel: [w2711 w2712] -> w2687
                tunnel: w2686 -> [w2711 w2713]
                frame "Left", Default {
                  n1116 = Increment(x=w2710) -> (x+1=w2709:u16)
                }
                frame "Right" {
                  n1117 = Increment(x=w2713) -> (x+1=w2712:u16)
                }
              }
              "nRewards_Left" <- w2688
              "nRewards_Right" <- w2687
              n1118 = Equal?(x=w2677, y=enum16{"Left", "Right"}."Left") -> (x = y?=w2676:bool)
              n1119 = Select(t=w2684, s=w2676, f=w2683) -> (s? t:f=w2682:i32)
              n1120 = call "myRIO_BRig_RT_dataExp_Tcycle_RewardPost.vi"() -> ("output_Tcycle_RewardPost"=w2699:i32)  [unwired: 11 in]
              n1121 = call "myRIO_BRig_RT_dataCurrent_nRewTrials.vi"() -> ("output_nRewTrials"=w2685:i32)  [unwired: 11 in]
              n1122 = Index Array(array=w2700, index=w2699) -> (element=w2702:u16)
              n1123 = Index Array(array=w2679, index=w2685) -> (element=w2674:u16)
              n1124 = Replace Array Subset(array=w2679, new element #1=u16 0 ("new element/subarray"), index #1=w2705, new element #2=w2702, index #2=w2703) -> (w2701:u16[])
              n1125 = Replace Array Subset(array=w2681, new element=w2674, index (row)=w2675, index (col)=w2682) -> (w2680:u16[][])
              n1126 = local write "nRewards_cur"(w2674) -> ()
            }
            frame 53 {
              n1127 = call "myRIO_BRig_RT__Case_Exp_State_RewardPost.vi"("input_state"=w2729, "input_dataCurrent"=w2732) -> ("output_state"=w2730:T2, "output_dataCurrent"=w2731:u16[])  [unwired: 8 in]
            }
            frame 54 {
              # "iState"
              # "Tcycle"
              # "counter"
              n1128 = call "myRIO_BRig_RT_dataCurrent_Tcycle_generic.vi"() -> ("output_Tcycle_generic"=w2757:i32)  [unwired: 11 in]
              n1129 = call "myRIO_BRig_RT_dataCurrent_count_generic.vi"() -> ("output_count_generic"=w2759:i32)  [unwired: 11 in]
              n1130 = call "myRIO_BRig_RT_dataExp_Tcycle_Wrong.vi"() -> ("output_Tcycle_Wrong"=w2755:i32)  [unwired: 11 in]
              n1131 = call "myRIO_BRig_RT__Case_Exp_subState_LC__Wrong.vi"("input_spout"=w2751, "input_dataCurrent"=w2752, "input_dataLC"=w2749) -> ()  [unwired: 6 in, 2 out]
              n1132 = Index Array(array=w2753, index=w2755) -> (element=w2756:u16)
              n1133 = call "myRIO_BRig_RT_dataCurrent_iState.vi"() -> ("output_iState"=w2743:i32)  [unwired: 11 in]
              n1134 = Replace Array Subset(array=w2752, new element #1=u16 0 ("new element/subarray"), index #1=w2759, new element #2=w2756, index #2=w2757, new element #3=u16 2 ("new element/subarray"), index #3=w2743) -> (w2754:u16[])
            }
            frame 55 {
              n1135 = call "myRIO_BRig_RT__Case_Exp_State_Wrong.vi"("input_state"=w2773, "input_dataCurrent"=w2782) -> ("output_state"=w2770:T2, "output_dataCurrent"=w2781:u16[])  [unwired: 8 in]
              n1136 = Not Equal?(x=w2773, y=w2770) -> (x != y?=w2772:bool)
              n1137 = Select(t=myRIO_BRig_RT__Case_Exp_stateList."SelectWrong_post" ("Enum"), s=w2772, f=w2770) -> (s? t:f=w2769:T2)
            }
            frame 56 {
            }
            frame 57 {
              # "iState"
              # "Tcycle"
              # "counter"
              n1138 = xnode "Read/Write Control"("FPGA VI Reference In"=w2809, "error in"=w2808, "SelectionState"=FALSE) -> ("error out"=→"error out 3":errorcluster)  [unwired: 1 out]
              n1139 = call "myRIO_BRig_RT_dataCurrent_Tcycle_generic.vi"() -> ("output_Tcycle_generic"=w2831:i32)  [unwired: 11 in]
              n1140 = call "myRIO_BRig_RT_dataCurrent_count_generic.vi"() -> ("output_count_generic"=w2829:i32)  [unwired: 11 in]
              n1141 = call "myRIO_BRig_RT_dataExp_Tcycle_Timeout.vi"() -> ("output_Tcycle_Timeout"=w2833:i32)  [unwired: 11 in]
              n1142 = call "myRIO_BRig_RT__Case_Exp_subState_LC__Timeout.vi"("input_spout"=w2824, "input_dataCurrent"=w2825, "input_dataLC"=w2823) -> ()  [unwired: 6 in, 2 out]
              n1143 = Index Array(array=w2827, index=w2833) -> (element=w2832:u16)
              n1144 = call "myRIO_BRig_RT_dataCurrent_iState.vi"() -> ("output_iState"=w2817:i32)  [unwired: 11 in]
              n1145 = Replace Array Subset(array=w2825, new element #1=u16 0 ("new element/subarray"), index #1=w2829, new element #2=w2832, index #2=w2831, new element #3=u16 3 ("new element/subarray"), index #3=w2817) -> (w2828:u16[])
            }
            frame 58 {
              n1146 = call "myRIO_BRig_RT__Case_Exp_State_Timeout.vi"("input_dataLC"=w2852, "input_state"=w2843, "input_dataCurrent"=w2857) -> ("output_state"=w2844:T2, "output_dataCurrent"=w2856:u16[])  [unwired: 6 in, 1 out]
              n1147 = Not Equal?(x=w2843, y=w2844) -> (x != y?=w2847:bool)
              n1148 = Select(t=myRIO_BRig_RT__Case_Exp_stateList."SelectTimeout_post" ("Enum"), s=w2847, f=w2844) -> (s? t:f=w2845:T2)
            }
            frame 59 {
            }
            frame 61 {
              # "Update dataBlock"
              n1149 = call "myRIO_BRig_RT__Case_Exp_State_endTrial1.vi"("input_spout"=w2890, "input_dataBlock"=w2889, "input_dataCurrent"=w2887) -> ("output_dataBlock"=w2888:u16[][], "output_dataCurrent"=w2886:u16[])  [unwired: 7 in]
            }
            frame 62 {
              # "update dataTrial"
              n1150 = call "myRIO_BRig_RT__Case_Exp_State_endTrial2.vi"("input_spout"=w2909, "input_dataTrial"=w2913, "input_dataCurrent"=w2911) -> ("output_dataTrial"=w2912:u16[][], "output_dataCurrent"=w2910:u16[])  [unwired: 7 in]
            }
            frame 63 {
              # "nRewTrials"
              # "iTrial"
              # "I_blockUntilReward"
              # "TPB"
              # "end block?"
              n1151 = local read "STOP_endTrial"() -> (w2939:bool)
              n1152 = local read "STOP_abort"() -> (w2938:bool)
              n1153 = xnode "Read/Write Control"("FPGA VI Reference In"=w2929, "error in"=w2928, "SelectionState"=FALSE) -> ("error out"=→"error out 2":errorcluster)  [unwired: 1 out]
              n1154 = local read "START"() -> (w2936:bool)
              n1155 = call "myRIO_BRig_RT_dataExp_IblockUntilReward.vi"() -> ("output_I_blockUntilReward"=w2946:i32)  [unwired: 11 in]
              n1156 = Index Array(array=w2932, index=w2946) -> (element=w2930:u16)
              n1157 = Not(x=w2936) -> (.not. x?=w2937:bool)
              n1158 = Not Equal To 0?(x=w2930) -> (x != 0?=w2944:bool)
              n1159 = Compound Arithmetic op=OR(w2939, w2937, w2938) -> (w2924:bool)
              n1160 = call "myRIO_BRig_RT_dataCurrent_nRewTrials.vi"() -> ("output_nRewTrials"=w2942:i32)  [unwired: 11 in]
              n1161 = call "myRIO_BRig_RT_dataCurrent_iTrial.vi"() -> ("output_iTrial"=w2943:i32)  [unwired: 11 in]
              n1162 = Select(t=w2942, s=w2944, f=w2943) -> (s? t:f=w2941:i32)
              n1163 = call "myRIO_BRig_RT_dataCurrent_TpB.vi"() -> ("output_TpB"=w2945:i32)  [unwired: 11 in]
              n1164 = Index Array(array=w2933, index #1=w2945, index #2=w2941) -> (element #1=w2934:u16, element #2=w2935:u16)
              n1165 = Less Or Equal?(x=w2934, y=w2935) -> (x <= y?=w2925:bool)
              n1166 = Or(x=w2924, y=w2925) -> (x .or. y?=w2922:bool)
              n1167 = Select(t=myRIO_BRig_RT__Case_Exp_stateList."saveData_dataBlock" ("Enum"), s=w2922, f=myRIO_BRig_RT__Case_Exp_stateList."dummyState" ("Enum")) -> (s? t:f=w2931:T2)
            }
            frame 66 {
              # "R"
              # "L"
              # "idxDataBlock"
              n1168 = Equal?(x=w2970, y=enum16{"Left", "Right"}."Left") -> (x = y?=w2969:bool)
              n1169 = call "myRIO_BRig_RT_dataCurrent_idxDataBlockL.vi"() -> ("output_idxDataBlock__L"=w2973:i32)  [unwired: 11 in]
              n1170 = call "myRIO_BRig_RT_dataCurrent_idxDataBlockR.vi"() -> ("output_idxDataBlock__R"=w2972:i32)  [unwired: 11 in]
              n1171 = Increment(x=w2964) -> (x+1=w2963:i32)
              n1172 = local read "START"() -> (w2993:bool)
              n1173 = local read "STOP_endBlock"() -> (w2988:bool)
              n1174 = local read "STOP_endTrial"() -> (w2991:bool)
              n1175 = local read "STOP_abort"() -> (w2990:bool)
              n1176 = Select(t=w2973, s=w2969, f=w2972) -> (s? t:f=w2967:i32)
              n1177 = To Unsigned Word Integer(number=w2963) -> (unsigned 16bit integer=w2965:u16)
              n1178 = Not(x=w2993) -> (.not. x?=w2992:bool)
              n1179 = Replace Array Subset(array=w2968, new element=w2965, index=w2967) -> (w2966:u16[])
              n1180 = Compound Arithmetic op=OR(w2992, w2988, w2991, w2990) -> (w2989:bool)
              n1181 = Select(t=myRIO_BRig_RT__Case_Exp_stateList."endExp" ("Enum"), s=w2989, f=myRIO_BRig_RT__Case_Exp_stateList."dummyState_endBlock" ("Enum")) -> (s? t:f=w2997:T2)
            }
            frame 68 {
            }
            frame 69 {
              n1182 = call "myRIO_BRig_RT_comm_webdav_connect.vi"("input_password"="Host Password", "input_username"="Host UserName") -> ("output_Iconnected"=w3018:bool, "output_hSession"=w3036:T7)  [unwired: 7 in, 1 out]
              "Connected To Host?" <- w3018
              n1183 = case shown="False" w3018 {
                frame False {
                  n1184 = One Button Dialog(message="Connection Failed!\nData not being saved!") -> ()  [unwired: 1 in, 1 out]
                }
                frame True {
                }
              }
            }
            frame 70 {
              n1185 = Select(t=myRIO_BRig_RT__Case_Exp_stateList."commUpload_dataBlock" ("Enum"), s=w3043, f=myRIO_BRig_RT__Case_Exp_stateList."endBlock") -> (s? t:f=w3041:T2)
            }
            frame 71 {
              n1186 = call "myRIO_BRig_RT_comm_webdav_uploadFile__data.vi"("input_fileName_prefix"=w3064, "input_fileName"="dataBlock" ("input_filename"), "input_hSession"=w3066) -> ()  [unwired: 8 in, 1 out]
            }
            frame 72 {
              n1187 = call "myRIO_BRig_RT_comm_webdav_uploadFile__data.vi"("input_fileName_prefix"=w3085, "input_fileName"="dataCurrent" ("input_filename"), "input_hSession"=w3087) -> ()  [unwired: 8 in, 1 out]
            }
            frame 73 {
              n1188 = call "myRIO_BRig_RT_comm_webdav_uploadFile__data.vi"("input_fileName_prefix"=w3106, "input_fileName"="dataExp" ("input_filename"), "input_hSession"=w3108) -> ()  [unwired: 8 in, 1 out]
            }
            frame 74 {
              n1189 = call "myRIO_BRig_RT_comm_webdav_uploadFile__data.vi"("input_fileName_prefix"=w3127, "input_fileName"="dataLC" ("input_filename"), "input_hSession"=w3129) -> ()  [unwired: 8 in, 1 out]
            }
            frame 75 {
              n1190 = call "myRIO_BRig_RT_comm_webdav_uploadFile__data.vi"("input_fileName_prefix"=w3151, "input_fileName"="dataTrial" ("input_filename"), "input_hSession"=w3153) -> ()  [unwired: 8 in, 1 out]
            }
            frame 78 {
              # "idxDataBlockR"
              # "idxDataBlockL"
              n1191 = call "myRIO_BRig_RT_dataCurrent_idxDataBlockL.vi"() -> ("output_idxDataBlock__L"=w3177:i32)  [unwired: 11 in]
              n1192 = call "myRIO_BRig_RT_dataCurrent_idxDataBlockR.vi"() -> ("output_idxDataBlock__R"=w3178:i32)  [unwired: 11 in]
              n1193 = Index Array(array=w3179, index #1=w3177, index #2=w3178) -> (element #1=w3176:u16, element #2=w3175:u16)
              n1194 = Greater?(x=w3176, y=w3175) -> (0:w3174:bool)
              n1195 = Select(t=w3176, s=w3174, f=w3175) -> (s? t:f=w3172:u16)
              n1196 = Increment(x=w3172) -> (x+1=w3171:u16)
              n1197 = To Long Integer(number=w3171) -> (32bit integer=w3170:i32)
              n1198 = Array Subset(array=w3173, length (row)=w3170) -> (w3169:u16[][])  [unwired: 3 in]
              n1199 = call "myRIO_BRig_RT_comm_webdav_saveArrayToFile__2D_u16.vi"("Array"=w3169, "input_filename"="dataBlock") -> ()  [unwired: 10 in]
            }
            frame 79 {
              n1200 = call "myRIO_BRig_RT_comm_webdav_saveArrayToFile__1D_u16.vi"("Array"=w3198, "input_filename"="dataCurrent") -> ()  [unwired: 10 in]
            }
            frame 80 {
              # "runTime"
              n1201 = Get Date/Time In Seconds() -> (seconds since 1Jan1904=w3226:timestamp)
              n1202 = To Double Precision Float(number=w3226) -> (double precision float=w3225:dbl)
              n1203 = call "myRIO_BRig_RT_dataExp_runTime_seconds.vi"() -> ("output_RunTime_minutes"=w3224:i32)  [unwired: 11 in]
              n1204 = Subtract(x=w3225, y=w3223) -> (x-y=w3220:dbl)
              n1205 = To Unsigned Word Integer(number=w3220) -> (unsigned 16bit integer=w3219:u16)
              n1206 = Replace Array Subset(array=w3218, new element=w3219, index=w3224) -> (w3221:u16[])
              n1207 = call "myRIO_BRig_RT_comm_webdav_saveArrayToFile__1D_u16.vi"("Array"=w3221, "input_filename"="dataExp") -> ()  [unwired: 10 in]
            }
            frame 81 {
              n1208 = call "myRIO_BRig_RT_comm_webdav_saveArrayToFile__1D_u16.vi"("Array"=w3245, "input_filename"="dataLC") -> ()  [unwired: 10 in]
            }
            frame 82 {
              # "idxTrial"
              n1209 = call "myRIO_BRig_RT_dataCurrent_idxDataTrial.vi"() -> ("output_idxDataTrial"=w3269:i32)  [unwired: 11 in]
              n1210 = Index Array(array=w3270, index=w3269) -> (element=w3262:u16)
              n1211 = Increment(x=w3262) -> ()  [unwired: 1 out]
              n1212 = To Long Integer(number=w3262) -> (32bit integer=w3266:i32)
              n1213 = Array Subset(array=w3267, length (row)=w3266) -> (w3268:u16[][])  [unwired: 3 in]
              n1214 = call "myRIO_BRig_RT_comm_webdav_saveArrayToFile__2D_u16.vi"("Array"=w3268, "input_filename"="dataTrial") -> ()  [unwired: 10 in]
            }
            frame 91 {
              n1215 = call "myRIO_BRig_RT_dataCurrent_iTrial.vi"() -> ("output_iTrial"=w3292:i32)  [unwired: 11 in]
              n1216 = Index Array(array=w3293, index=w3292) -> (element=w3291:u16)
              n1217 = Equal?(x=w3291, y=u16 1) -> (x = y?=w3289:bool)
              n1218 = Equal To 0?(x=w3300) -> (x = 0?=w3301:bool)
              n1219 = Select(t=u16 13, s=w3289, f=u16 15) -> (s? t:f=w3286:u16)
              n1220 = Select(t=w3286, s=w3301, f=w3300) -> (s? t:f=w3299:u16)
              n1221 = Decrement(x=w3299) -> (x-1=w3298:u16)
              n1222 = Equal To 0?(x=w3298) -> (x = 0?=w3297:bool)
              n1223 = Select(t=myRIO_BRig_RT__Case_Exp_stateList."initTrial" ("Enum"), s=w3297, f=w3295) -> (s? t:f=w3294:u16)
            }
            frame 92 {
              n1224 = call "myRIO_BRig_RT_dataCurrent_iTrial.vi"() -> ("output_iTrial"=w3325:i32)  [unwired: 11 in]
              n1225 = Index Array(array=w3326, index=w3325) -> (element=w3324:u16)
              n1226 = Equal?(x=w3324, y=u16 1) -> (x = y?=w3322:bool)
              n1227 = Equal To 0?(x=w3333) -> (x = 0?=w3334:bool)
              n1228 = Select(t=u16 1, s=w3322, f=u16 3) -> (s? t:f=w3319:u16)
              n1229 = Select(t=w3319, s=w3334, f=w3333) -> (s? t:f=w3332:u16)
              n1230 = Decrement(x=w3332) -> (x-1=w3331:u16)
              n1231 = Equal To 0?(x=w3331) -> (x = 0?=w3330:bool)
              n1232 = Select(t=myRIO_BRig_RT__Case_Exp_stateList."initBlock" ("Enum"), s=w3330, f=w3328) -> (s? t:f=w3327:u16)
            }
          }
          n1233 = Select(t=w1090, s=w1093, f=w1091) -> (s? t:f=w1092:bool)
          n1234 = Or(x=w1052, y=w1053) -> (x .or. y?=w1051:bool)
          n1235 = Or(x=w1132, y=w1131) -> (x .or. y?=w1050:bool)
          n1236 = case shown="True" w1160 {
            tunnel: w1157 -> [w1181 w1189]
            tunnel: w1159 -> [_ w1185]
            tunnel: w1158 -> [_ w1184]
            tunnel: w1064 -> [_ w1183]
            tunnel: w1129 -> [_ w1182]
            tunnel: [w1181 w1188] -> w1156
            tunnel: w1155 -> [w1180 w1187]
            tunnel: [w1180 w1186] -> w1154
            frame False {
            }
            frame True {
              n1237 = call "myRIO_BRig_RT__Case_Exp__recordLick.vi"("intput_state__trialEnd"=w1182, "intput_state__trialStart"=w1183, "input_lick__R"=w1184, "input_lick__L"=w1185, "input_dataCurrent"=w1187, "input_dataLick"=w1189) -> ("output_dataCurrent"=w1186:u16[], "output_dataLick"=w1188:u16[][])  [unwired: 4 in]
            }
          }
          n1238 = Or(x=w1133, y=w1117) -> (x .or. y?=w1106:bool)
          n1239 = Or(x=w1116, y=w1134) -> (x .or. y?=w1130:bool)
          n1240 = Or(x=w1161, y="STOP_abort") -> (x .or. y?=w1163:bool)
          n1241 = Or(x=w1096, y=w1097) -> (x .or. y?=w1094:bool)
          n1242 = Or(x=w1098, y=w1097) -> (x .or. y?=w1095:bool)
          n1243 = Select(t=w1079, s=w1080, f=w1078) -> (s? t:f=w1063:u16)
          n1244 = Select(t=w1081, s=w1083, f=w1082) -> (s? t:f=w1062:u16)
          n1245 = Select(t=u16 0, s=w1086, f=w1085) -> (s? t:f=w1070:u16)
          n1246 = xnode "Read/Write Control"("FPGA VI Reference In"=w1108, "error in"=w1107, "A3_SL"=w1051, "A1_SR"=w1050, "A6_Act"=w1092, "audioTrigger_L"=w1106, "audioAmp_L"=w1143, "audioFreq_L_kHz"=w1115, "audioTrigger_R"=w1130, "audioAmp_R"=w1144, "audioFreq_R_kHz"=w1145, "laser1_Event"=w1094, "laser1_On"=w1095, "laser2_Event"=w1049, "laser2_On"=w1048) -> ("FPGA VI Reference Out"=w1153:refnum<k20>, "error out"=w1152:errorcluster, "AnaIn_0"=w1056:i16, "AnaIn_1"=w1069:i16)
          n1247 = call "myRIO_BRig_RT_dataAnalog_enterData__PortC.vi"("input_iState"=w1064, "input_AI0"=w1056, "input_iEvent"=w1070, "input_AI1"=w1069, "input_iTrial"=w1063, "input_iBlock"=w1062, "input_index"=w1071, "input_dataAnalog"=w1089) -> ("output_dataAnalog"=w1088:u16[][])  [unwired: 3 in]
          n1248 = call "myRIO_BRig_RT_TCP__v3__PortC.vi"("input_hTCP"=w1076, "input_AI1"=w1069, "input_AI0"=w1056, "input_I_connected_TCP"=w1072, "input_iBlock"=w1062, "input_spout"=w1061, "input_iTrial"=w1063, "input_error"=w1074, "input_countTrial"=w1058, "input_iState"=w1064) -> ("output_hTCP"=w1075:refnum<k5>, "output_countTrial"=w1057:u16, "output_error"=w1073:errorcluster)  [unwired: 3 in]
          n1249 = node-c288() -> ()  [unwired: 1 in, 1 out]
          n1250 = Increment(x=w1070) -> (x+1=w1077:u16)
          n1251 = Increment(x=w1071) -> (x+1=w1087:i32)
          "cState" <- w1064
        }
        n1252 = node-c288(w998) -> ()  [unwired: 1 out]
        n1253 = flat-sequence {
          tunnel: w994 -> [w1043]
          tunnel: w993 -> [w1042]
          tunnel: [w1041] -> w986
          tunnel: [w1040] -> w985
          tunnel: [w1046] -> w987
          tunnel: [w1047] -> w992
          tunnel: w986 -> [w1047]
          tunnel: w985 -> [w1046]
          frame #0 {
            w1037 = u8 0
            w1038 = u16 0 ("AudioLeft_phase_inc")
            w1039 = FALSE
            n1254 = xnode "Read/Write Control"("FPGA VI Reference In"=w1043, "error in"=w1042, "Counts_Reset"=TRUE, "audioTrigger_L"=w1039, "audioFreq_L_kHz"=w1037, "audioAmp_L"=w1038, "audioTrigger_R"=w1039, "audioFreq_R_kHz"=w1037, "audioAmp_R"=w1038, "A3_SL"=w1039, "A1_SR"=w1039, "A6_Act"=w1039) -> ("FPGA VI Reference Out"=w1041:refnum<k20>, "error out"=w1040:errorcluster)
          }
          frame #1 {
            w1045 = FALSE ("START")
            n1255 = local write "START"(w1045) -> ()
            n1256 = local write "STOP_endTrial"(w1045) -> ()
            n1257 = local write "STOP_endBlock"(w1045) -> ()
          }
        }
        n1258 = stacked-sequence {
          tunnel: w970 -> [w1017 _]
          tunnel: w968 -> [w1018 _]
          tunnel: w967 -> [_ w1023]
          tunnel: w966 -> [_ w1022]
          tunnel: w965 -> [_ w1021]
          tunnel: w964 -> [w1011 _]
          tunnel: w939 -> [w1008 _]
          tunnel: w938 -> [w1007 _]
          frame #0 {
            n1259 = call "myRIO_BRig_RT_dataCurrent_idxDataLick.vi"() -> ("output_idxDataLick"=w1012:i32)  [unwired: 11 in]
            n1260 = Index Array(array=w1011, index=w1012) -> (element=w1014:u16)
            n1261 = Array Subset(array=w1008, length (row)=w1007) -> (w1009:u16[][])  [unwired: 3 in]
            n1262 = Increment(x=w1014) -> (x+1=w1015:u16)
            n1263 = call "myRIO_BRig_RT_comm_webdav_saveArrayToFile__1D_u16.vi"("Array"=w1018, "input_filename"="dataMTrig") -> ()  [unwired: 10 in]
            n1264 = To Long Integer(number=w1015) -> (32bit integer=w1013:i32)
            n1265 = Array Subset(array=w1017, length (row)=w1013) -> (w1016:u16[][])  [unwired: 3 in]
            n1266 = call "myRIO_BRig_RT_comm_webdav_saveArrayToFile__2D_u16.vi"("Array"=w1016, "input_filename"="dataLick") -> ()  [unwired: 10 in]
            n1267 = call "myRIO_BRig_RT_comm_webdav_saveArrayToFile__2D_u16.vi"("Array"=w1009, "input_filename"="dataAnalog") -> ()  [unwired: 10 in]
          }
          frame #1 {
            n1268 = case shown="True" w1023 {
              tunnel: w1022 -> [_ w1025]
              tunnel: w1021 -> [_ w1024]
              frame False {
              }
              frame True {
                n1269 = stacked-sequence {
                  tunnel: w1025 -> [w1027 w1034 w1036]
                  tunnel: w1024 -> [w1028 w1033 _]
                  frame #0 {
                    n1270 = call "myRIO_BRig_RT_comm_webdav_uploadFile__announce.vi"("input_addText"=TRUE, "input_fileName_prefix"=w1028, "intput_fileName"="curExp_end", "intput_hSession"=w1027) -> ("output_Isuccess"=w1026:bool)  [unwired: 6 in, 1 out]
                    n1271 = case shown="True" w1026 {
                      frame False {
                        n1272 = One Button Dialog(message="!!! Warning !!! Your data is located at C:\\BehaviorRig\\commTransfer") -> ()  [unwired: 1 in, 1 out]
                      }
                      frame True {
                        n1273 = Wait (ms)(milliseconds to wait=u32 20) -> ()  [unwired: 1 out]
                      }
                    }
                  }
                  frame #1 {
                    n1274 = call "myRIO_BRig_RT__endExp_sendData.vi"("input_fileName_prefix"=w1033, "input_hSession"=w1034) -> ()  [unwired: 8 in, 2 out]
                  }
                  frame #2 {
                    n1275 = local write "Connected To Host?"(FALSE ("Connected To Host?")) -> ()
                    n1276 = call <vilib>:"Close Session.vi"("session handle"=w1036) -> ()  [unwired: 14 in, 1 out]
                  }
                }
              }
            }
          }
        }
      }
    }
    n1277 = local read "STOP_abort"() -> (w44:bool)
  }
  n1278 = case shown="True" w5 {
    tunnel: w4 -> [_ w3357]
    tunnel: w3 -> [_ w3356]
    frame False {
    }
    frame True {
      n1279 = call "myRIO__TCP_disconnect_forWrite.vi"("input_error"=w3356, "input_hTCP"=w3357) -> ()  [unwired: 9 in, 1 out]
    }
  }
  n1280 = xnode "Read/Write Control"("FPGA VI Reference In"=w16, "error in"=w15, "FPGA_Stop"=TRUE) -> ("FPGA VI Reference Out"=w21:refnum<k20>, "error out"=w22:errorcluster)
  n1281 = xnode "Close FPGA VI Reference"("FPGA VI Reference In"=w21, "error in"=w22) -> ("error out"=w20:errorcluster)
  n1282 = call <vilib>:"Reset myRIO.vi"("error in (no error)"=w20) -> ()  [unwired: 10 in, 1 out]
